vi "BRig_RT_start_v1,18__PortC.vi"() -> ()   [LabVIEW 2014]
uses:
  myRIO_BRig_RT__Case_Exp_stateList.ctl
  myRIO_BRig_RT__Case_NonExp_stateList.ctl
  <vilib>/WebDAVClient/Advanced/SessionHandle.ctl
  <vilib>/Platform/TimedLoop/XDataNode/timing_clust.ctl
  <vilib>/Platform/TimedLoop/XDataNode/nitl_modes.ctl
  <vilib>/Platform/TimedLoop/XDataNode/wakeup.ctl
  <vilib>/myRIO/Common/Instrument Driver Framework/myRIO v1.0/UART/vis/myRIO v1.0 Close UART.vi
  <vilib>/FPGAPlugInAG/myRIO-1900/niLvFpga_Open_myRIO-1900.vi
  <vilib>/rvi/interface/common/dynamic/niFpgaDynamicAddResources.vi
  <vilib>/Utility/error.llb/Error Cluster From Error Code.vi
  <vilib>/rvi/errors/niLvFpgaAdjustHostInterfaceError.vi
  <vilib>/Utility/file.llb/Read From Spreadsheet File (I64).vi
  <vilib>/Utility/file.llb/Write To Spreadsheet File (DBL).vi
  <vilib>/FPGAPlugInAG/Dynamic/niLvFpga_Close_Dynamic.vi
  <vilib>/myRIO/Common/Instrument Driver Framework/Utilities/vis/FPGA Ref Manager.vi
  <vilib>/myRIO/Common/Instrument Driver Framework/myRIO v1.0/myRIO v1.0 Reset FPGA.vi
  <vilib>/myRIO/Common/Instrument Driver Framework/myRIO v1.0/IRQ/vis/myRIO v1.0 IRQ Info FGV.vi
  <vilib>/myRIO/Common/Instrument Driver Framework/myRIO v1.0/IRQ/vis/myRIO v1.0 Timer IRQ Info FGV.vi
  <vilib>/myRIO/Common/Instrument Driver Framework/myRIO v1.0/IRQ/vis/myRIO v1.0 ISR Agent.vi
  <vilib>/rvi/interface/nirviOpenFPGA/nirviOpenFPGA.xnode
  BRig_FPGA_v3,94__PortC__build.lvbitx
  BRig_FPGA_v3,94__PortC.vi
  <vilib>/rvi/interface/nirviReadWriteControl/nirviReadWriteControl.xnode
  <vilib>/Platform/TimedLoop/XDataNode/XDataNode.xnode
  <vilib>/rvi/interface/nirviCloseFPGA/nirviCloseFPGA.xnode
  <vilib>/Platform/TimedLoop/XDataNode/XDNodeRunTimeDep.lvlib
  <vilib>/rvi/interface/Simulation/niFpgaSimulationCallBeginRW.vi
  <vilib>/myRIO/Instrument Drivers/Utilities/Utilities.lvlib
  NiFpgaLv.dll
  <vilib>/WebDAVClient/NI_WebDAV.lvlib
panel:
  out "DAB_flipLR":bool caption="Flip?\n(DAB)"
  in  "LaserFiber_V_l2":dbl
  in  "LaserFiber_V_l1":dbl
  out "Solenoid R":bool
  out "Solenoid L":bool
  out "Laser2":bool
  out "Laser1":bool
  out "FreeReward_c_R":u16
  out "FreeReward_c_L":u16
  in  "Laser2_LED":bool
  in  "Laser1_LED":bool
  in  "lick_Rising(F)_or_Falling(T)":bool
  out "T_ExpRun_min":dbl
  out "stop_TimedLoop":bool
  out "BTPR_avg_R":dbl
  out "T2R_avg_R":dbl
  out "BTPR_avg_L":dbl
  out "T2R_avg_L":dbl
  out "BTPR_block":u16
  out "T2R_block":u16
  in  "comm_WebDAV_connect":bool
  in  "I_sendData":bool
  in  "comm_TCP_connect":bool
  out "nRewards_total":u16 caption="# Rewards in Current Block"
  out "BUR_target":u16 caption="Target Trials Per Block"
  in  "input_Threshold_reset":bool
  out "nTrial":u16
  out "allReward_R":bool
  out "allReward_L":bool
  out "Threshold":bool
  out "tLoop":dbl format="%#_2g"
  out "L_Power_l2":dbl
  out "comm_TCP":bool
  in  "get_countPerMS":bool
  out "SolenoidReward":bool
  out "L_Power_l1":dbl caption="LaserPower"
  in  "Recording":bool
  out "FPGA_count2ms":dbl=159.0
  out "error out":errorcluster
  out "cSpout":enum16{"Left", "Right"}(ring) caption="Left or Right Spout"
  out "A4":u32 caption="LickCounter_Right"
  out "A2":u32 caption="LickCounter_Left"
  out "nRewards_Right":u16 caption="# Rewards Total (Right)"
  out "nRewards_Left":u16 caption="# Rewards Total (Left)"
  out "nRewards_cur":u16 caption="# Rewards in Current Block"
  out "TpB_target":u16 caption="Target Trials Per Block"
  out "cState_NonExp":T1 caption="WarmUp State"
  out "iBlock":u16 caption="Current Block"
  out "cState":T2 caption="Experimental State"
  out "iTrial":u16 caption="Current Trial"
  in  "Data Set Prefix":string="Exp1_TM2"
  out "comm_WebDAV":bool
  in  "Host Password":string="sabalab"
  in  "Host UserName":string="Test2"
  in  "STOP_abort":bool caption="Stop LabView\n(Stops myRio and FPGA)"
  in  "STOP_endBlock":bool caption="Stop Experiment\n@ End of Block"
  in  "STOP_endTrial":bool caption="Stop Experiment\n@ End of Trial"
  in  "START":bool caption="Start Experiment"
  # "Experimental Run"
  # "Recording Rig"
  # "FPGA Conversion\n[counts per ms]"
  # "RealTime Cycle\nShould be <5ms"
  # "STOP experiment at"
  # "Exp Run Time"
  # "Reset"
  # "min"
  # "Communication with Host"
  # "Lick Counter"
  # "Block Target"
  # "Give Water?\n(Reward)"
  # "# Blocks"
  # "Experimental State"
  # "Left/Right"
  # "# Trials"
  # "# Rewards"
  # "Left           Right"
  # "Bad Trials\nPost Reward"
  # "Trials 2 Reward"
  # "Direction\n(NonSpecific Licking)"
  # "Block"
  # "Laser1"
  # "Laser2"
  # "# Trials"
  # "# Rewards"
  # "Current\nBlock"
  # "L          R"
  # "Power [V]"
  # "avg L"
  # "Toggle\nLED"
  # "Total"
  # "# Rewards"
  # "Laser Trigger"
  # "# Trials"
  # "avg R"
  # "1          2"
  # "Fiber Angle\n[V]"
  # "Left           Right"
  # "FreeRewards"
  # "Solenoid Trigger"
  # "WarmUp State"
  # "Lick Detection\nRising (F) or Falling (T)"
  # "L          R"
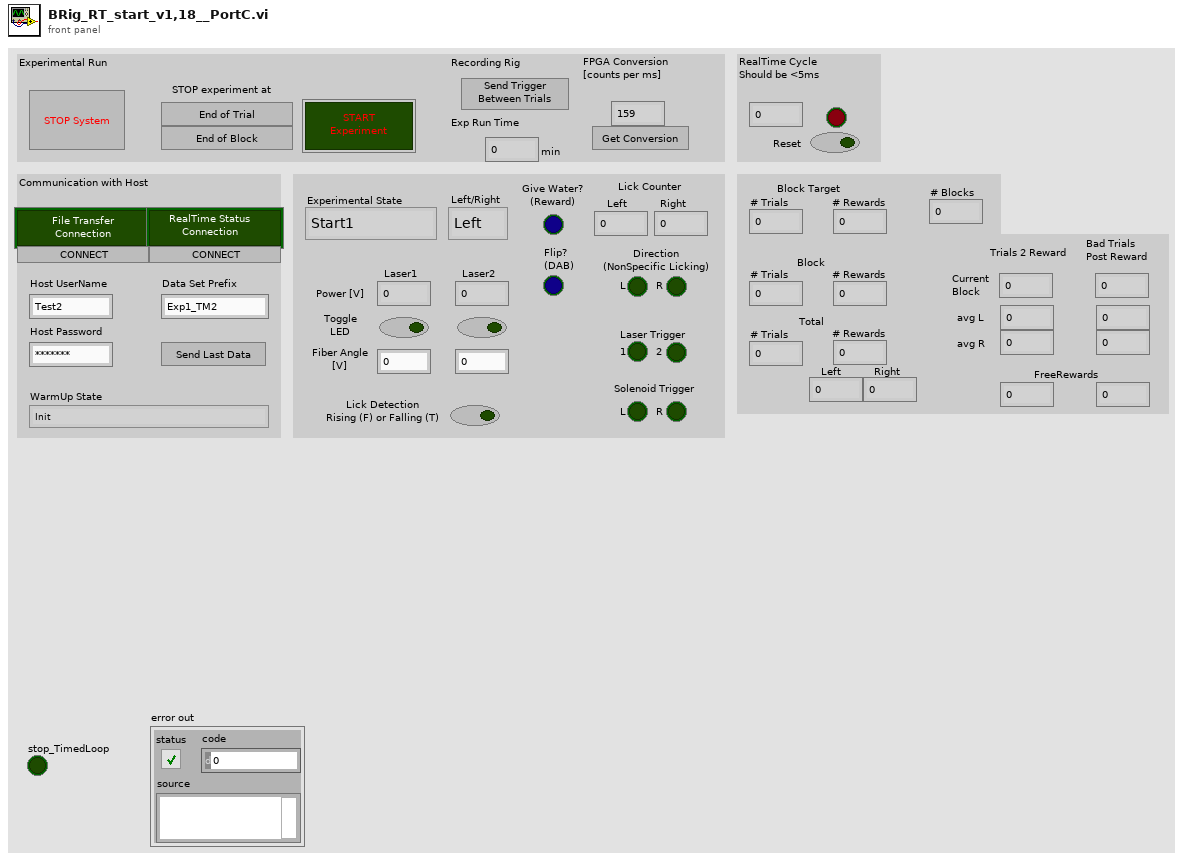
[diagram p1: front panel]
types:
  T1 = typedef "myRIO_BRig_RT__Case_NonExp_stateList.ctl" = enum16{"Init", "UploadSettings_pre", "UploadSettings_Read_dataExp", "UploadSettings_dataExp_1", "UploadSettings_dataExp_2", "UploadSettings_Read_dataLC", "UploadSettings_dataLC_1", "UploadSettings_dataLC_2", "UploadSettings_dataLC_3", "UploadSettings_dataLC_4", "UploadSettings_Read_dataMTrig", "UploadSettings_dataMTrig_1", "UploadSettings_post", "Idle_pre", "IdleEmpty", "IdleEmpty2", "IdleEmpty3", "IdleEmpty4", "Idle", "Idle_2", "Idle_3", "Idle_4", "Idle_5", "Idle_6", "Idle_post", "Cue_pre__pre", "Cue_pre", "Cue", "Cue_LED", "Cue_post", "RewardCalibration_pre", "RewardCalibration", "DispenseWater_pre__pre", "DispenseWater_pre", "DispenseWater", "DispenseWater_post", "TestConnection", "SendData", "Get_FPGA_count_per_ms", "End", "commTCP_connect"}
  T2 = typedef "myRIO_BRig_RT__Case_Exp_stateList.ctl" = enum16{"Start1", "Start2", "Start3", "saveSettings1", "saveSettings2", "saveSettings3", "saveSettings4", "saveSettings_LC_ENL_l1", "saveSettings_LC_ENL_l2", "saveSettings_LC_Cue_l1", "saveSettings_LC_Cue_l2", "saveSettings6_LC_l1_Other", "SaveSettings6_LC_l2_Other", "setSettings_Audio", "setSettings_Laser", "initBlock_pre", "initBlock", "initBlock2", "initBlock_post", "initTrial_pre", "initTrial", "initTrial2", "initTrial3", "initTrial4", "initTrial_LC_ENL1", "initTrial_LC_Cue1", "initTrial_LC_Cue1_2", "initTrial_LC_Sel", "initTrial_post", "ENL1_pre", "ENL1", "ENL1_post", "ENL1Penalty_pre", "ENL1Penalty", "ENL2_pre", "ENL2", "ENL2Penalty_pre", "ENL2Penalty", "Cue1_pre", "Cue1", "Cue1_post", "Cue1Penalty_pre", "Cue1Penalty", "Cue2_pre", "Cue2", "Cue2Penalty_pre", "Cue2Penalty", "Selection_pre", "Selection", "Select_post", "SelectReward_pre", "SelectReward", "SelectRewardPost_pre", "SelectRewardPost", "SelectWrong_pre", "SelectWrong", "SelectWrong_post", "SelectTimeout_pre", "SelectTimeout", "SelectTimeout_post", "endTrial_pre", "endTrial1", "endTrial2", "endTrial3", "endTrial_post", "endBlock_pre", "endBlock", "endBlock_post", "endExp", "commConnect", "commUpload_pre", "commUpload_dataBlock", "commUpload_dataCurrent", "commUpload_dataExp", "commUpload_dataLC", "commUpload_dataTrial", "commUpload_post", "saveData_pre", "saveData_dataBlock", "saveData_dataCurrent", "saveData_dataExp", "saveData_dataLC", "saveData_dataTrial", "saveData_post", "empty_endBlock1", "empty_endBlock2", "empty_endTrial1", "empty_endTrial2", "empty_endTrial3", "empty_endTrial4", "empty_endTrial5", "dummyState", "dummyState_endBlock", "FreeReward_pre", "FreeReward", "FreeRewardPost_pre", "FreeRewardPost"}
  T3 = enum8{"Enabled", "Disabled", "Disabled and Grayed Out"}
  T4 = typedef "NI_WebDAV.lvlib/SessionHandle.ctl" = refnum<k1>
  T5 = typedef "XDNodeRunTimeDep.lvlib/timing_clust.ctl" = cluster{"Expected End [f-1]":u64, "Actual End [f-1]":u64, "Finished Late? [f-1]":bool, "Expected End [i-1]":u64, "Actual End [i-1]":u64, "Finished Late? [i-1]":bool, "Expected Start [i]":u64, "Actual Start [i]":u64, "Expected Start [f]":u64, "Actual Start [f]":u64, "Source Name":string, "Structure Name":string, "Period":i64, "Deadline":i64, "Offset":i64, "Start":i64, "Priority":i32, "Timeout":i32, "Mode":T6, "Wakeup Reason":T7, "Error":errorcluster, "Source Type":string, "Secondary Source Type":string, "Global End Time":u64, "Global Start Time":u64, "Frame Duration":u64, "Iteration Duration":u64, "Assigned CPU":i32, "I/O Scan Engine Mode":u32}
  T6 = typedef "XDNodeRunTimeDep.lvlib/nitl_modes.ctl" = enum32{"No Change", "Process missed periods, maintain original phase", "Discard missed periods, maintain original phase", "Process missed periods, ignore original phase", "Discard missed periods, ignore original phase"}
  T7 = typedef "XDNodeRunTimeDep.lvlib/wakeup.ctl" = enum32{"Normal", "Aborted", "Asynchronous wakeup", "Timing source error", "Timed loop error", "Timeout"}
  T8 = cluster{"read mode":enum16{"polling", "blocking"}, "write mode":enum16{"polling", "blocking"}}
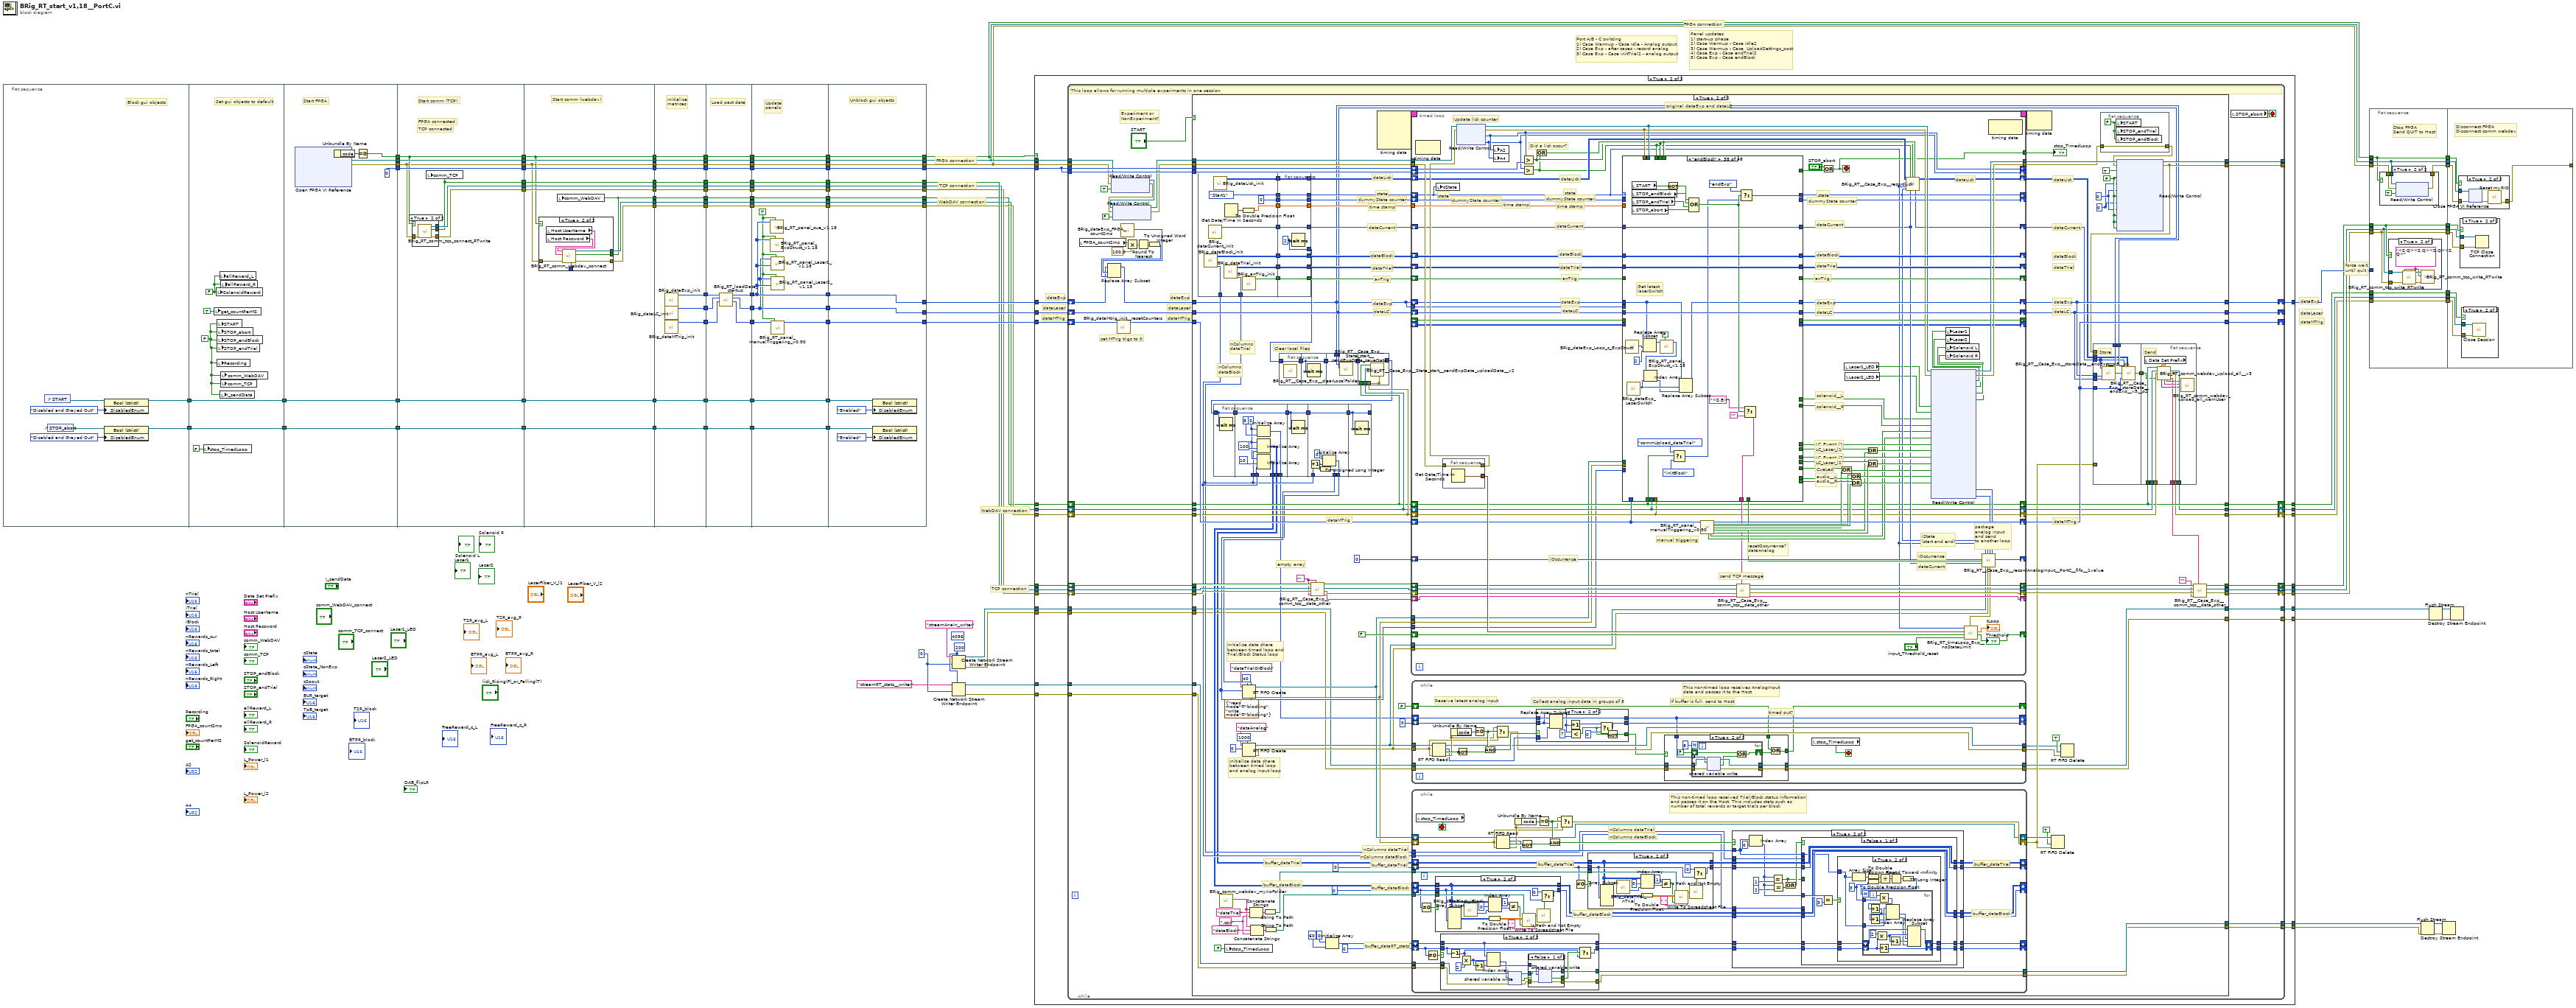
[diagram p0: block diagram]
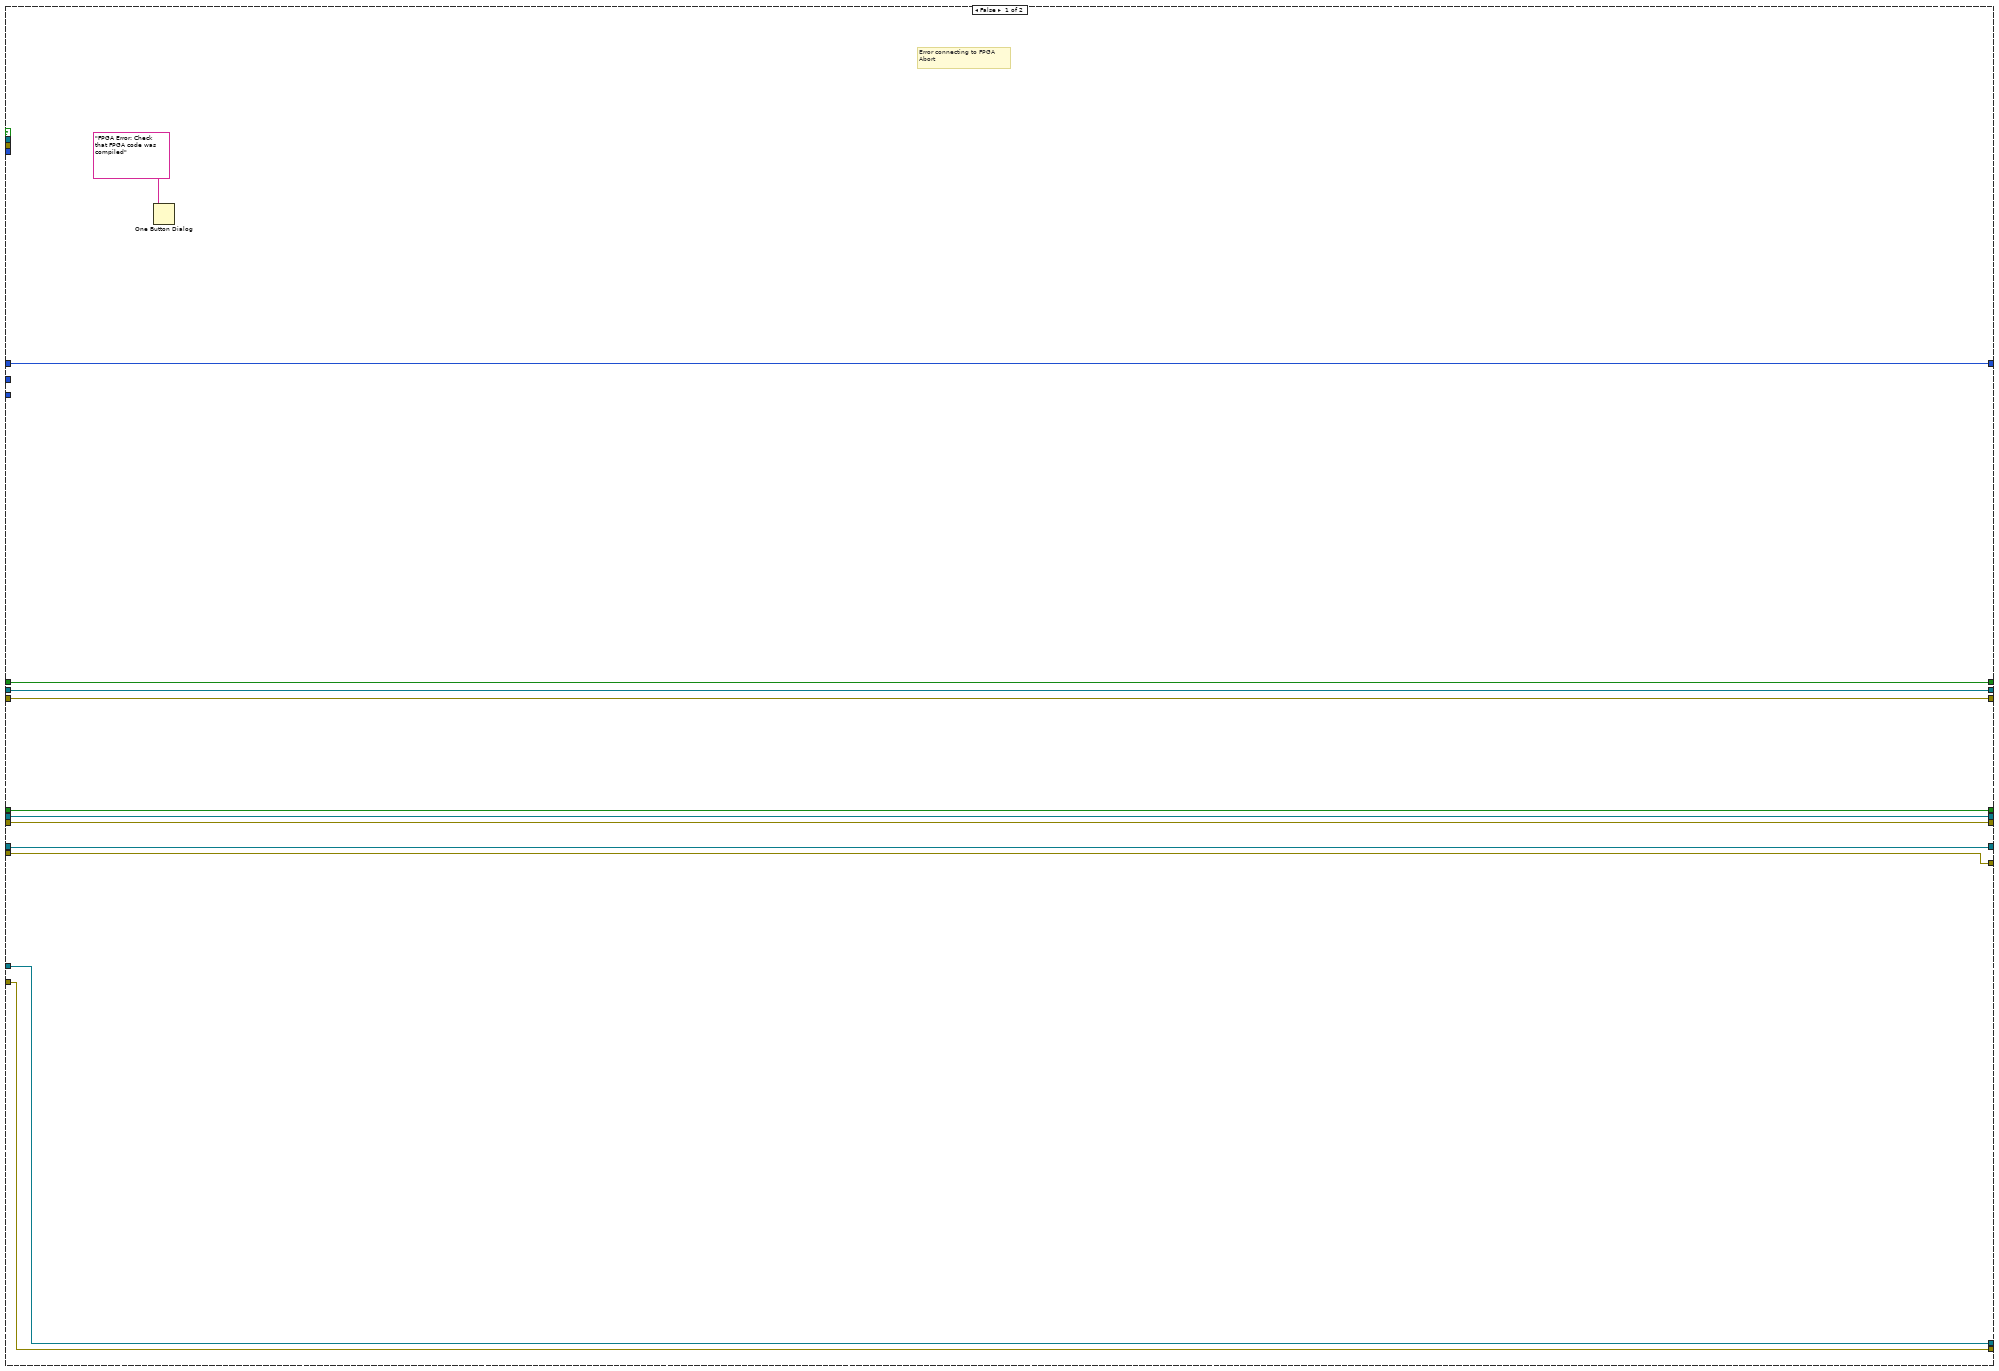
[diagram p2: hidden frame]
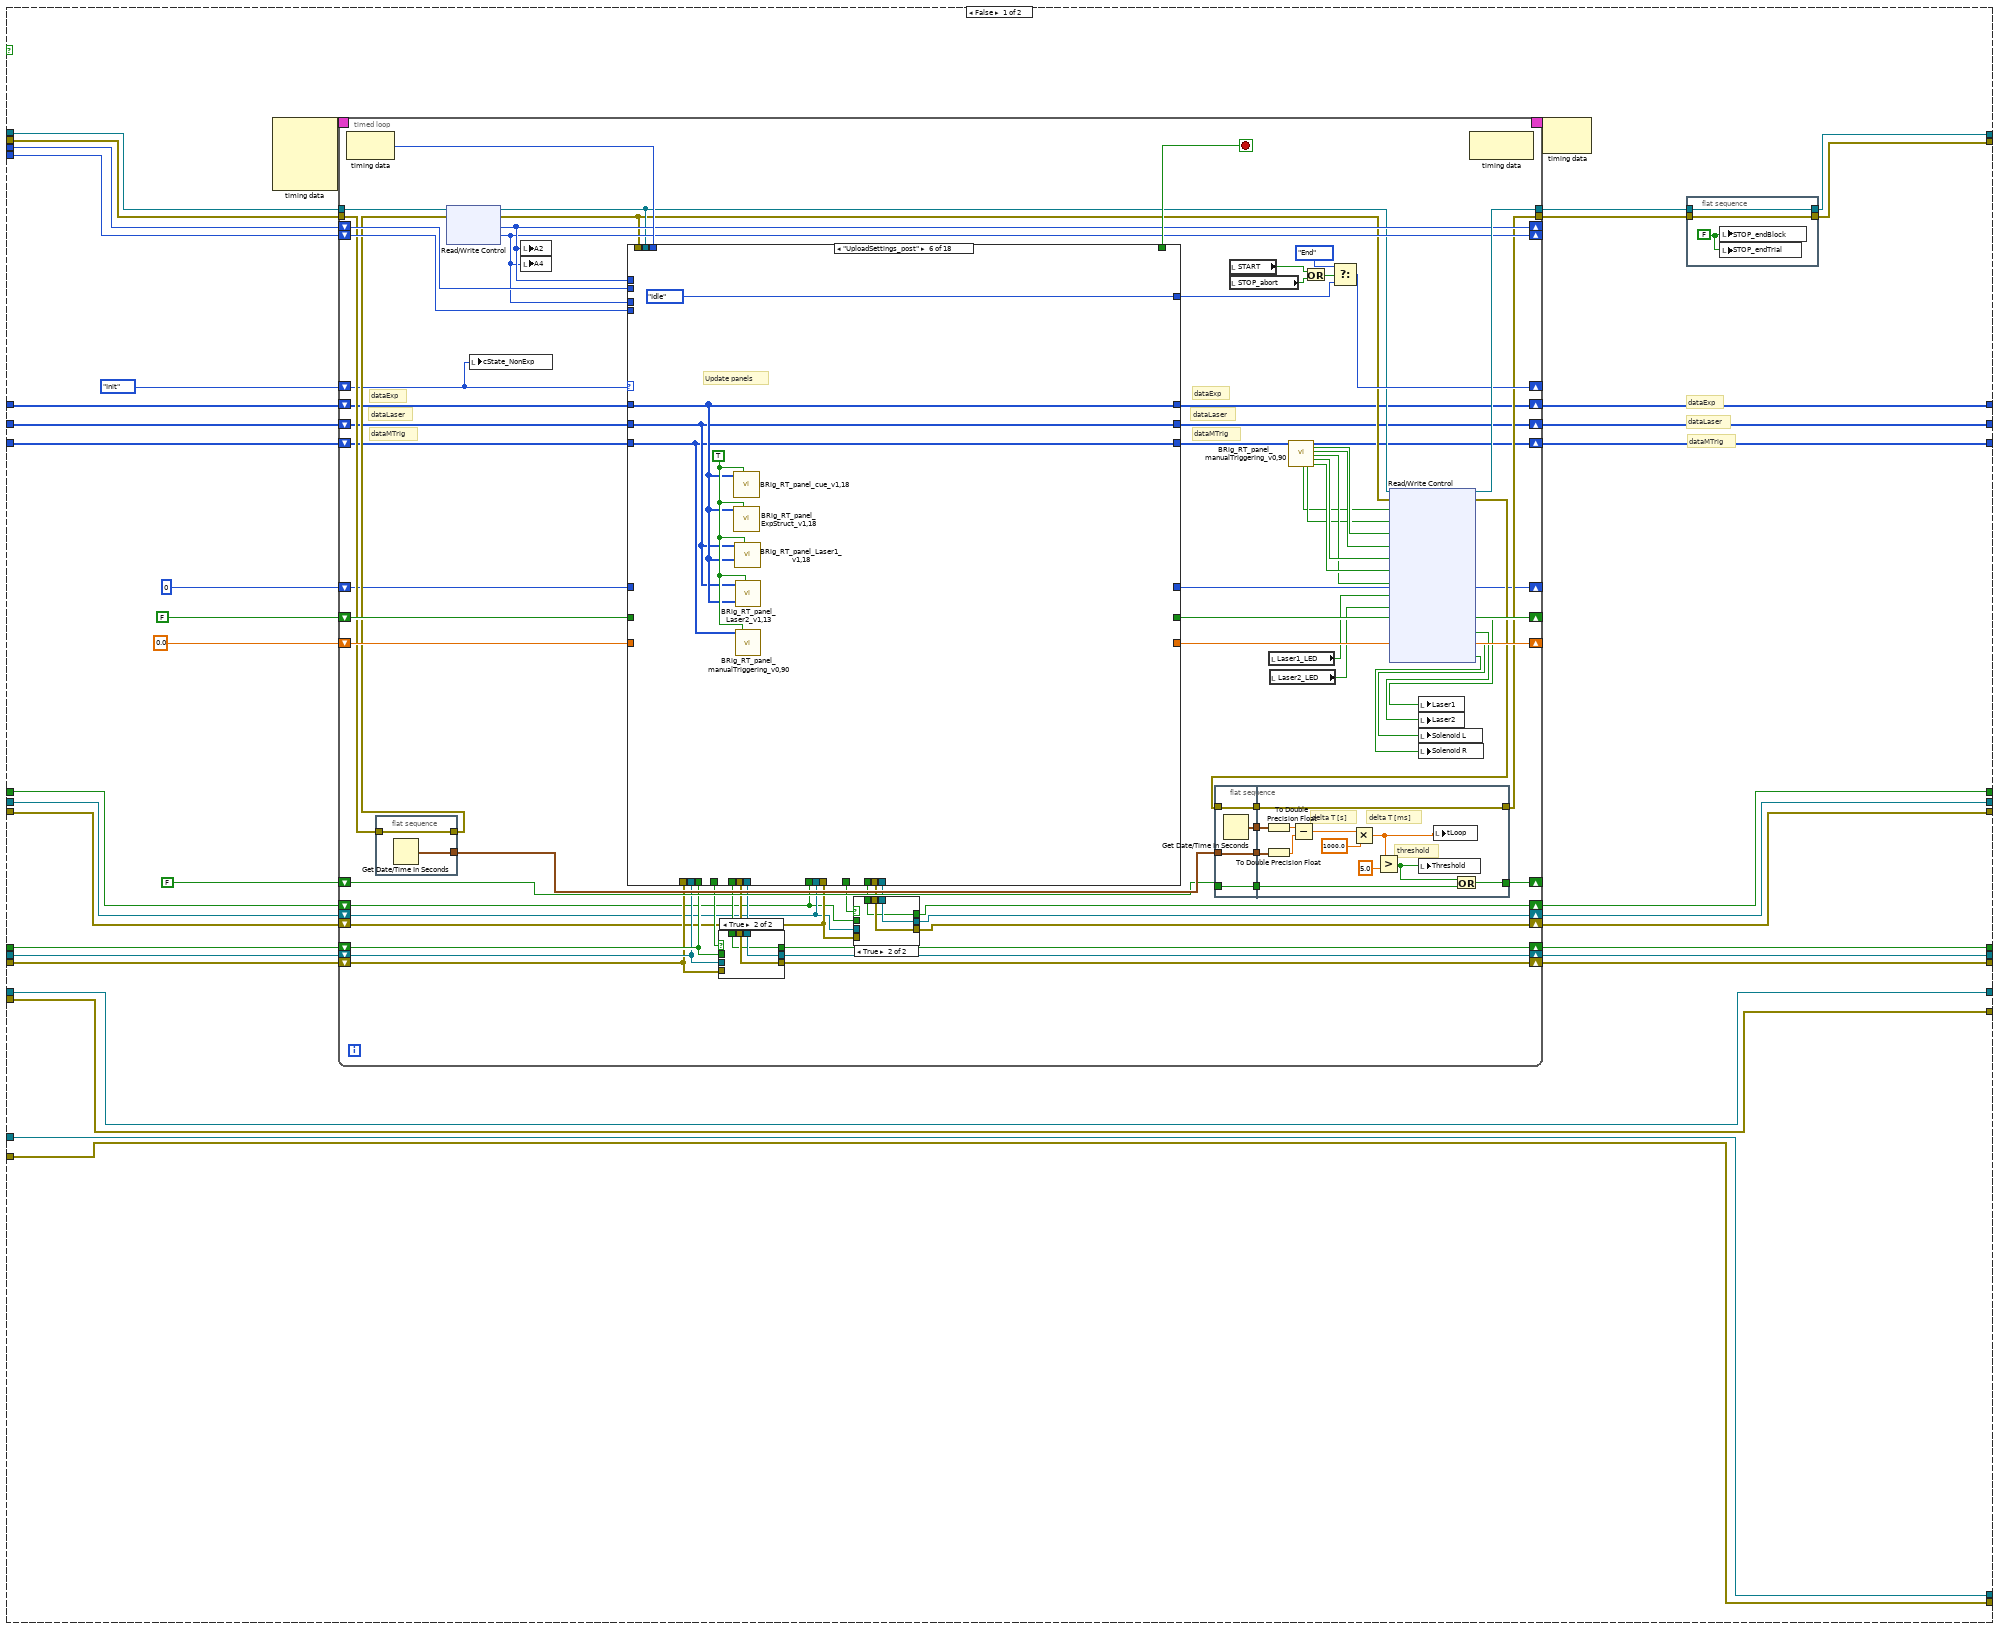
[diagram p3: hidden frame]
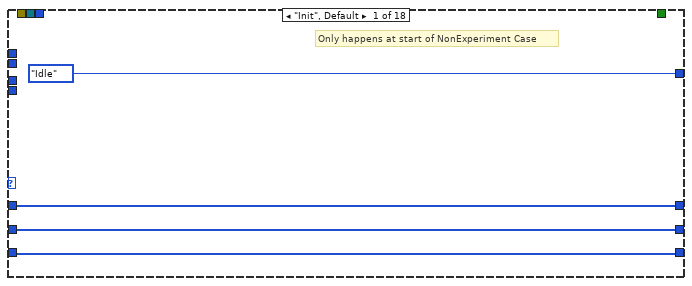
[diagram p6: hidden frame]
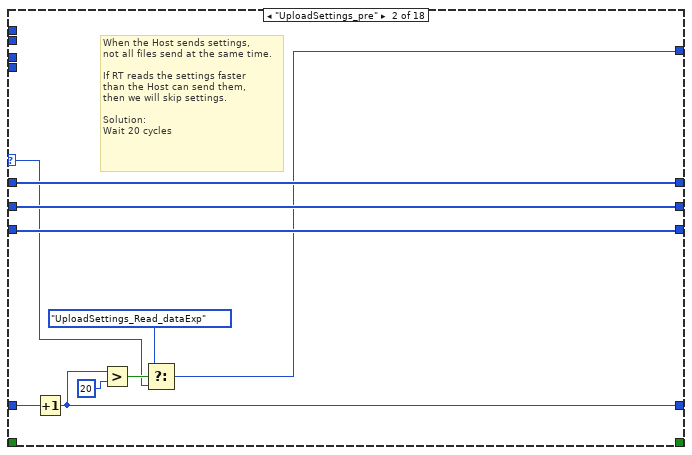
[diagram p7: hidden frame]
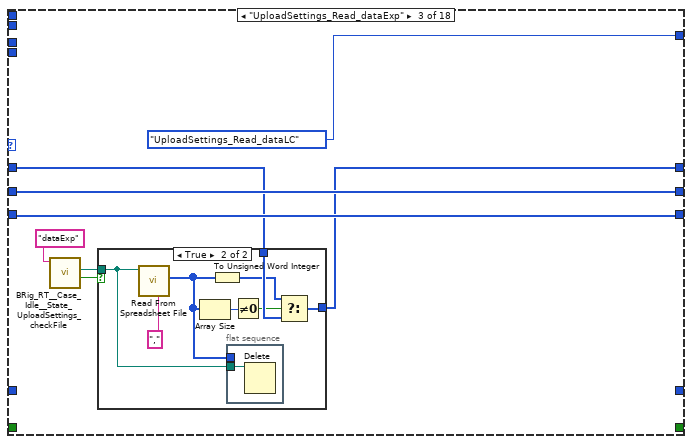
[diagram p8: hidden frame]
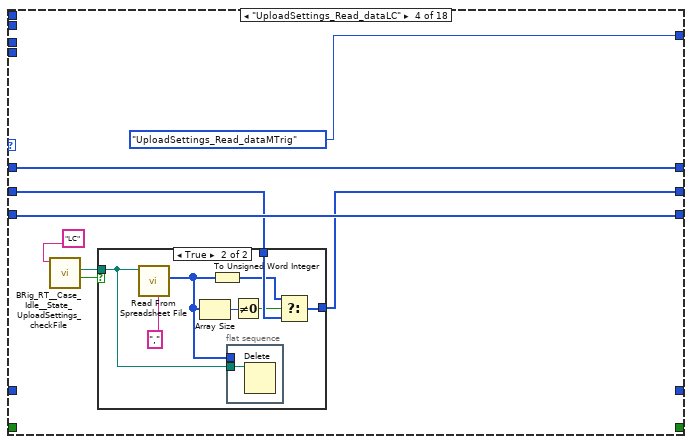
[diagram p10: hidden frame]
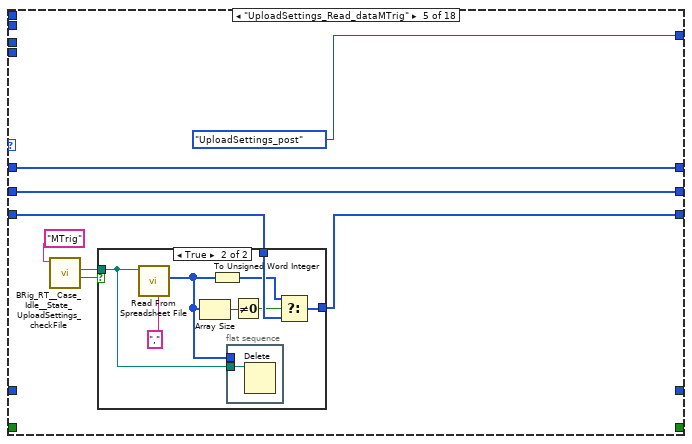
[diagram p12: hidden frame]
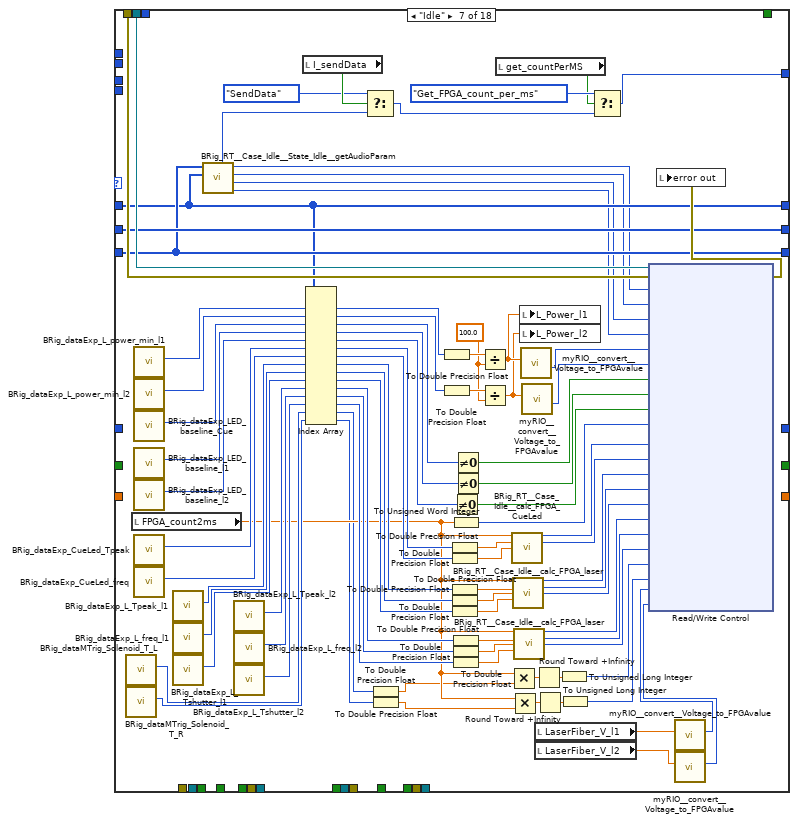
[diagram p14: hidden frame]
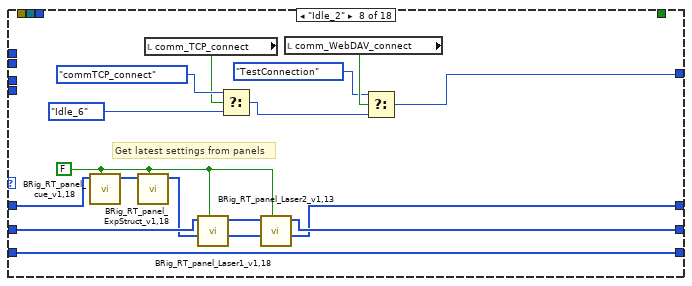
[diagram p15: hidden frame]
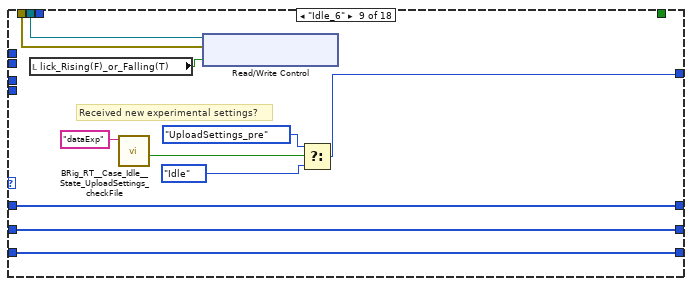
[diagram p16: hidden frame]
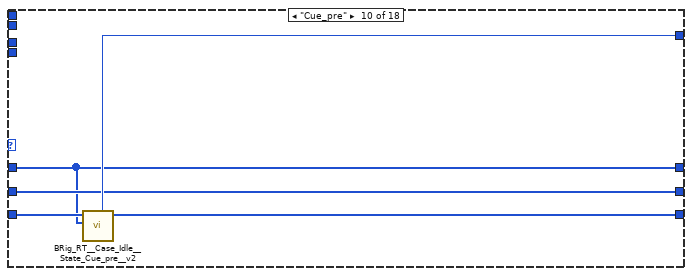
[diagram p17: hidden frame]
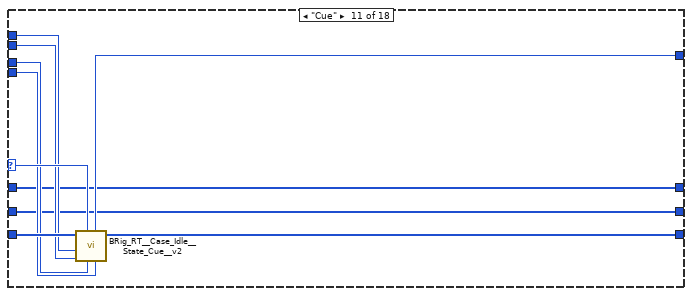
[diagram p18: hidden frame]
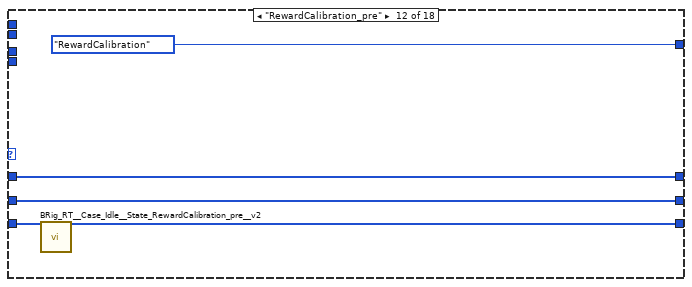
[diagram p19: hidden frame]
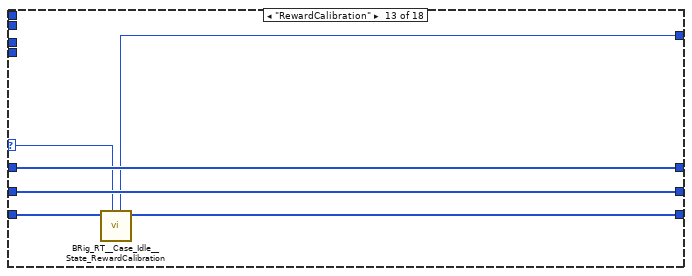
[diagram p20: hidden frame]
diagram:
  w8 = u16 0 ("element")
  (unwired) 4096 ("reader buffer size")
  w9 = 200 ("reader buffer size")
  # "Panel updates\n1) start-up phase\n2) Case Warmup - Case Idle2\n3) Case Warmup - Case  UploadSettings_post\n4) Case Exp - Case endTrial2\n5) Case Exp - Case endBlock"
  # "WebDAV connection"
  # "TCP connection"
  # "WebDAV connection"
  # "TCP connection"
  # "FPGA connection"
  # "FPGA connection"
  # "Port A/B - C switcing\n1) Case Warmup - Case Idle - Analog output\n2) Case Exp - after cases - record analog\n3) Case Exp - Case initTrial2 - analog output"
  # "force wait\nuntil quit"
  # "dataLaser"
  # "dataExp"
  # "dataMTrig"
  n1 = flat-sequence {
    tunnel: [w123] -> w106
    tunnel: [w122] -> w102
    tunnel: [w132] -> w107
    tunnel: w106 -> [w132]
    tunnel: [w131] -> w103
    tunnel: w102 -> [w131]
    tunnel: [w138] -> w120
    tunnel: [w140] -> w119
    tunnel: [u32 0] -> w118
    tunnel: [w136] -> w117
    tunnel: [w135] -> w108
    tunnel: w107 -> [w135]
    tunnel: [w134] -> w104
    tunnel: w103 -> [w134]
    tunnel: w120 -> [w146]
    tunnel: w119 -> [w149]
    tunnel: w118 -> [w148]
    tunnel: w117 -> [w147]
    tunnel: [w146] -> w116
    tunnel: [w149] -> w115
    tunnel: [w148] -> w114
    tunnel: [w147] -> w113
    tunnel: [w141] -> w112
    tunnel: [w145] -> w111
    tunnel: [w144] -> w110
    tunnel: [w143] -> w109
    tunnel: w108 -> [w143]
    tunnel: [w142] -> w105
    tunnel: w104 -> [w142]
    tunnel: w116 -> [w160]
    tunnel: w115 -> [w168]
    tunnel: w114 -> [w167]
    tunnel: w113 -> [w161]
    tunnel: w112 -> [w166]
    tunnel: w111 -> [w165]
    tunnel: w110 -> [w164]
    tunnel: [w160] -> w73
    tunnel: [w168] -> w72
    tunnel: [w167] -> w71
    tunnel: [w161] -> w70
    tunnel: [w166] -> w69
    tunnel: [w165] -> w68
    tunnel: [w164] -> w67
    tunnel: [w163] -> w66
    tunnel: w109 -> [w163]
    tunnel: [w162] -> w65
    tunnel: w105 -> [w162]
    tunnel: [w159] -> w64
    tunnel: [w157] -> w63
    tunnel: [w158] -> w62
    tunnel: w73 -> [w193]
    tunnel: [w193] -> w61
    tunnel: w72 -> [w192]
    tunnel: [w192] -> w60
    tunnel: w71 -> [w191]
    tunnel: [w191] -> w59
    tunnel: w70 -> [w190]
    tunnel: [w190] -> w58
    tunnel: w69 -> [w189]
    tunnel: [w189] -> w57
    tunnel: w68 -> [w188]
    tunnel: [w188] -> w56
    tunnel: w67 -> [w187]
    tunnel: [w187] -> w55
    tunnel: w66 -> [w186]
    tunnel: [w186] -> w54
    tunnel: w65 -> [w185]
    tunnel: [w185] -> w53
    tunnel: w64 -> [w184]
    tunnel: [w184] -> w52
    tunnel: w63 -> [w183]
    tunnel: [w183] -> w51
    tunnel: w62 -> [w182]
    tunnel: [w182] -> w50
    tunnel: [w181] -> w49
    tunnel: [w180] -> w48
    tunnel: [w179] -> w47
    tunnel: w61 -> [w211]
    tunnel: [w211] -> w46
    tunnel: w60 -> [w210]
    tunnel: [w210] -> w44
    tunnel: w59 -> [w209]
    tunnel: [w209] -> w42
    tunnel: w58 -> [w208]
    tunnel: [w208] -> w40
    tunnel: w57 -> [w207]
    tunnel: [w207] -> w38
    tunnel: w56 -> [w206]
    tunnel: [w206] -> w36
    tunnel: w55 -> [w205]
    tunnel: [w205] -> w34
    tunnel: w54 -> [w204]
    tunnel: [w204] -> w32
    tunnel: w53 -> [w203]
    tunnel: [w203] -> w30
    tunnel: w52 -> [w202]
    tunnel: [w202] -> w28
    tunnel: w51 -> [w201]
    tunnel: [w201] -> w26
    tunnel: w50 -> [w200]
    tunnel: [w200] -> w24
    tunnel: w49 -> [w195]
    tunnel: [w194] -> w22
    tunnel: w48 -> [w197]
    tunnel: [w196] -> w20
    tunnel: w47 -> [w199]
    tunnel: [w198] -> w19
    tunnel: w46 -> [w228]
    tunnel: [w228] -> w45
    tunnel: w44 -> [w227]
    tunnel: [w227] -> w43
    tunnel: w42 -> [w226]
    tunnel: [w226] -> w41
    tunnel: w40 -> [w225]
    tunnel: [w225] -> w39
    tunnel: w38 -> [w224]
    tunnel: [w224] -> w37
    tunnel: w36 -> [w223]
    tunnel: [w223] -> w35
    tunnel: w34 -> [w222]
    tunnel: [w222] -> w33
    tunnel: w32 -> [w221]
    tunnel: [w221] -> w31
    tunnel: w30 -> [w220]
    tunnel: [w220] -> w29
    tunnel: w28 -> [w219]
    tunnel: [w219] -> w27
    tunnel: w26 -> [w218]
    tunnel: [w218] -> w25
    tunnel: w24 -> [w217]
    tunnel: [w217] -> w23
    tunnel: w22 -> [w214]
    tunnel: [w213] -> w21
    tunnel: w20 -> [w215]
    tunnel: w19 -> [w216]
    tunnel: [w216] -> w18
    tunnel: [w215] -> w17
    tunnel: [w235] -> w83
    tunnel: [w236] -> w84
    tunnel: [w237] -> w85
    tunnel: [w242] -> w89
    tunnel: [w243] -> w121
    tunnel: [w244] -> w96
    tunnel: [w245] -> w95
    tunnel: w45 -> [w245]
    tunnel: w43 -> [w244]
    tunnel: w41 -> [w243]
    tunnel: w39 -> [w242]
    tunnel: w37 -> [w237]
    tunnel: w35 -> [w236]
    tunnel: w33 -> [w235]
    tunnel: w31 -> [w239]
    tunnel: w29 -> [w238]
    tunnel: w27 -> [w233]
    tunnel: w25 -> [w234]
    tunnel: w23 -> [w232]
    tunnel: [w234] -> w77
    tunnel: [w233] -> w78
    tunnel: [w232] -> w79
    tunnel: [w229] -> w92
    tunnel: [w230] -> w91
    tunnel: [w231] -> w90
    tunnel: w21 -> [w231]
    tunnel: w18 -> [w229]
    tunnel: w17 -> [w230]
    frame #0 {
      # "Block gui objects"
      n2 = control-ref of="START"() -> (w127:refnum<vi>)
      n3 = control-ref of="STOP_abort"() -> (w124:refnum<vi>)
      n4 = property class="Bool (strict)"(reference=w127, "DisabledEnum"=T3."Disabled and Grayed Out" ("Disabled")) -> (reference out=w123:refnum<vi>)  [unwired: 1 in, 1 out]
      n5 = property class="Bool (strict)"(reference=w124, "DisabledEnum"=T3."Disabled and Grayed Out" ("Disabled")) -> (reference out=w122:refnum<vi>)  [unwired: 1 in, 1 out]
    }
    frame #1 {
      w129 = FALSE ("SolenoidReward")
      w130 = FALSE
      # "Set gui objects to default"
      n6 = local write "stop_TimedLoop"(FALSE ("stop_TimedLoop")) -> ()
      n7 = local write "get_countPerMS"(TRUE ("get_countPerMS")) -> ()
      n8 = local write "SolenoidReward"(w129) -> ()
      n9 = local write "START"(w130) -> ()
      n10 = local write "STOP_abort"(w130) -> ()
      n11 = local write "STOP_endBlock"(w130) -> ()
      n12 = local write "STOP_endTrial"(w130) -> ()
      n13 = local write "Recording"(w130) -> ()
      n14 = local write "allReward_L"(w129) -> ()
      n15 = local write "I_sendData"(w130) -> ()
      n16 = local write "comm_WebDAV"(w130) -> ()
      n17 = local write "comm_TCP"(w130) -> ()
      n18 = local write "allReward_R"(w129) -> ()
    }
    frame #2 {
      # "Start FPGA"
      n19 = xnode "Open FPGA VI Reference"() -> ("FPGA VI Reference Out"=w140:refnum<k20>, "error out"=w138:errorcluster)  [unwired: 2 in]
      n20 = Unbundle By Name(w138) -> ("code"=w137:i32)
      n21 = Equal To 0?(x=w137) -> (x = 0?=w136:bool)
    }
    frame #3 {
      # "TCP connected"
      # "Start comm (TCP)"
      # "FPGA connected"
      n22 = case shown="True" w147 {
        selector: w147 -> [w150 _]
        tunnel: w146 -> [w152 w156]
        tunnel: [refnum<k5> refnum ("output_hTCP") w155] -> w145
        tunnel: [w150 w154] -> w141
        tunnel: [w152 w153] -> w144
        frame False {
        }
        frame True {
          n23 = call "BRig_RT_comm_tcp_connect_RTwrite.vi"("input_error"=w156) -> ("output_error"=w153:errorcluster, "output_connected"=w154:bool, "output_hTCP"=w155:refnum<k5>)  [unwired: 8 in]
        }
      }
      n24 = local write "comm_TCP"(w141) -> ()
    }
    frame #4 {
      # "Start comm (webdav)"
      n25 = case shown="True" w161 {
        selector: w161 -> [w170 _]
        tunnel: [w169 w176] -> w159
        tunnel: [w170 w175] -> w157
        tunnel: w160 -> [w171 w174]
        tunnel: [w171 w173] -> w158
        tunnel: [_ w172] -> _
        frame False {
          w169 = T4 refnum items=["Session NI_WebDAV"] ("output_hSession")
        }
        frame True {
          n26 = local read "Host UserName"() -> (w177:string)
          n27 = local read "Host Password"() -> (w178:string)
          n28 = call "BRig_RT_comm_webdav_connect.vi"("input_error"=w174, "input_password"=w178, "input_username"=w177) -> ("output_error"=w173:errorcluster, "output_Iconnected"=w175:bool, "output_hSession"=w176:T4, "output_code"=w172:u8)  [unwired: 5 in]
        }
      }
      n29 = local write "comm_WebDAV"(w157) -> ()
    }
    frame #5 {
      # "Initialize\nmatrices"
      n30 = call "BRig_dataExp_init.vi"() -> ("output_dataExp"=w179:u16[])  [unwired: 11 in]
      n31 = call "BRig_dataLC_init.vi"() -> ("output_dataLC"=w180:u16[])  [unwired: 11 in]
      n32 = call "BRig_dataMTrig_init.vi"() -> ("output_dataMTrig"=w181:u16[])  [unwired: 5 in]
    }
    frame #6 {
      # "Load past data"
      n33 = call "BRig_RT_loadData_startup.vi"("input_dataMTrig"=w195, "input_dataLC"=w197, "input_dataExp"=w199) -> ("output_dataMTrig"=w194:u16[], "output_dataLC"=w196:u16[], "output_dataExp"=w198:u16[])  [unwired: 6 in]
    }
    frame #7 {
      w212 = TRUE ("input_setValues")
      # "Update\npanels"
      n34 = call "BRig_RT_panel_cue_v1,18.vi"("input_setValues"=w212, "input_dataExp"=w216) -> ()  [unwired: 9 in, 1 out]
      n35 = call "BRig_RT_panel_ExpStruct_v1,18.vi"("input_setValues"=w212, "input_dataExp"=w216) -> ()  [unwired: 9 in, 1 out]
      n36 = call "BRig_RT_panel_Laser1_v1,18.vi"("input_setValues"=w212, "input_dataExp"=w216, "input_dataLC"=w215) -> ()  [unwired: 7 in, 2 out]
      n37 = call "BRig_RT_panel_Laser2_v1,13.vi"("input_setValues"=w212, "input_dataExp"=w216, "input_dataLC"=w215) -> ()  [unwired: 7 in, 2 out]
      n38 = call "BRig_RT_panel_manualTriggering_v0,90.vi"("input_dataMTrig"=w214, "input_setValues"=w212) -> ("output_dataMTrig"=w213:u16[])  [unwired: 10 in, 7 out]
    }
    frame #8 {
      # "Unblock gui objects"
      n39 = property class="Bool (strict)"(reference=w239, "DisabledEnum"=T3."Enabled" ("Disabled")) -> ()  [unwired: 1 in, 2 out]
      n40 = property class="Bool (strict)"(reference=w238, "DisabledEnum"=T3."Enabled" ("Disabled")) -> ()  [unwired: 1 in, 2 out]
    }
  }
  n41 = Create Network Stream Writer Endpoint(7:w9, 9:w8, 11:"streamAnaIn_writer" ("reader name")) -> (0:w10:errorcluster, 3:w11:refnum<k21>)  [unwired: 4 in]
  n42 = Create Network Stream Writer Endpoint(7:w9, 9:w8, 11:"streamRT_stats__writer" ("writer name")) -> (0:w5:errorcluster, 3:w6:refnum<k21>)  [unwired: 4 in]
  n43 = case shown="True" w89 {
    tunnel: w121 -> [_ w284]
    tunnel: w96 -> [_ w283]
    tunnel: w95 -> [_ w282]
    tunnel: [w257 w281] -> w93
    tunnel: w92 -> [w257 w280]
    tunnel: w91 -> [_ w279]
    tunnel: w90 -> [_ w278]
    tunnel: w85 -> [w256 w277]
    tunnel: w84 -> [w255 w276]
    tunnel: w83 -> [w254 w275]
    tunnel: [w256 w274] -> w82
    tunnel: [w255 w273] -> w81
    tunnel: [w254 w272] -> w80
    tunnel: w79 -> [w253 w271]
    tunnel: w78 -> [w252 w270]
    tunnel: w77 -> [w251 w269]
    tunnel: [w253 w268] -> w76
    tunnel: [w252 w267] -> w75
    tunnel: [w251 w266] -> w74
    tunnel: [w250 w265] -> w14
    tunnel: [w249 w264] -> w13
    tunnel: w11 -> [w250 w263]
    tunnel: w10 -> [w249 w262]
    tunnel: w6 -> [w247 w261]
    tunnel: w5 -> [w246 w260]
    tunnel: [w247 w259] -> w2
    tunnel: [w246 w258] -> w1
    frame False {
      # "Error connecting to FPGA\nAbort"
      n44 = One Button Dialog(message="FPGA Error: Check that FPGA code was compiled") -> ()  [unwired: 1 in, 1 out]
    }
    frame True {
      # "dataExp"
      # "dataLaser"
      # "dataMTrig"
      n45 = while {
        tunnel: w283 -> [w322]
        tunnel: w282 -> [w327]
        tunnel: w284 -> [w330]
        tunnel: w284 -> [w329]
        tunnel: [w320] -> _
        tunnel: [w319] -> _
        shift-right: [w318] -> _
        shift-left: w278 -> [w315]
        shift-right: [w316] -> _
        shift-left: w279 -> [w317]
        shift-right: [w286] -> w281
        shift-left: w280 -> [w295]
        shift-right: [w310] -> w274
        shift-left: w277 -> [w313]
        shift-right: [w309] -> w273
        shift-left: w276 -> [w312]
        shift-right: [w308] -> w272
        shift-left: w275 -> [w311]
        shift-right: [w304] -> w268
        shift-left: w271 -> [w307]
        shift-right: [w303] -> w267
        shift-left: w270 -> [w306]
        shift-right: [w302] -> w266
        shift-left: w269 -> [w305]
        tunnel: [w294] -> w265
        tunnel: [w293] -> w264
        tunnel: w263 -> [w292]
        tunnel: w262 -> [w291]
        tunnel: w261 -> [w290]
        tunnel: w260 -> [w289]
        tunnel: [w288] -> w259
        tunnel: [w287] -> w258
        stop <- w328 stop-if-true
        # "set MTrig trigs to 0"
        # "dataExp"
        # "dataLaser"
        # "dataMTrig"
        # "Experiment or\nNonExperiment?"
        # "This loop allows for running multiple experiments in one session"
        n46 = local read "FPGA_count2ms"() -> (w299:dbl)
        n47 = xnode "Read/Write Control"("FPGA VI Reference In"=w322, "error in"=w327, "Counts_Reset"=TRUE) -> ("FPGA VI Reference Out"=w324:refnum<k20>, "error out"=w325:errorcluster)
        n48 = xnode "Read/Write Control"("FPGA VI Reference In"=w324, "error in"=w325, "Counts_Reset"=FALSE) -> ("FPGA VI Reference Out"=w321:refnum<k20>, "error out"=w323:errorcluster)
        n49 = call "BRig_dataMtrig_init__resetCounters.vi"("input_dataMTrig"=w315) -> ("output_dataMTrig"=w314:u16[])  [unwired: 10 in]
        n50 = call "BRig_dataExp_FPGA_count2ms.vi"() -> ("output_FPGA_count2ms"=w300:i32)  [unwired: 11 in]
        n51 = Multiply(x=w299, y=100.0) -> (x*y=w297:dbl)
        n52 = Round To Nearest(number=w297) -> (nearest integer value=w296:dbl)
        n53 = To Unsigned Word Integer(number=w296) -> (unsigned 16bit integer=w301:u16)
        n54 = Replace Array Subset(array=w295, new element=w301, index=w300) -> (w285:u16[])
        n55 = case shown="True" "START" {
          tunnel: w330 -> [w366 w945]
          tunnel: w329 -> [w365 w944]
          tunnel: w323 -> [w363 w933]
          tunnel: w321 -> [w364 w934]
          tunnel: [w361 w942] -> w320
          tunnel: [w359 w911] -> w319
          tunnel: w314 -> [w355 w931]
          tunnel: [w354 w917] -> w318
          tunnel: w317 -> [w353 w881]
          tunnel: w285 -> [w333 w834]
          tunnel: [w352 w916] -> w316
          tunnel: [w351 w915] -> w286
          tunnel: w313 -> [w350 w925]
          tunnel: w312 -> [w349 w924]
          tunnel: w311 -> [w348 w923]
          tunnel: [w347 w900] -> w310
          tunnel: [w346 w899] -> w309
          tunnel: [w345 w898] -> w308
          tunnel: w307 -> [w344 w880]
          tunnel: w306 -> [w343 w879]
          tunnel: w305 -> [w342 w878]
          tunnel: [w341 w907] -> w304
          tunnel: [w340 w906] -> w303
          tunnel: [w339 w908] -> w302
          tunnel: w292 -> [w337 w839]
          tunnel: w291 -> [w336 w838]
          tunnel: [w337 w837] -> w294
          tunnel: [w336 w836] -> w293
          tunnel: w290 -> [w335 w830]
          tunnel: w289 -> [w334 w831]
          tunnel: [w335 w825] -> w288
          tunnel: [w334 w824] -> w287
          frame False {
            # "dataExp"
            # "dataLaser"
            # "dataMTrig"
            n56 = node-c288() -> (w369:T5)  [unwired: 4 in]
            n57 = timed-loop {
              timing: w369 -> [_]
              timing-out: [_] -> w368
              shift-right: [w437] -> _
              shift-left: myRIO_BRig_RT__Case_NonExp_stateList."Init" ("Enum") -> [w406]
              shift-right: [w435] -> _
              shift-left: w366 -> [w436]
              shift-right: [w433] -> _
              shift-left: w365 -> [w434]
              tunnel: [w443] -> w362
              tunnel: [w419] -> w360
              tunnel: w363 -> [w426]
              tunnel: w364 -> [w444]
              shift-right: [w429] -> _
              shift-left: FALSE -> [w430]
              shift-right: [w427] -> _
              shift-left: 0.0 -> [w428]
              shift-right: [w416] -> _
              shift-left: FALSE -> [w417]
              shift-right: [w415] -> w354
              shift-left: w355 -> [w407]
              shift-right: [w401] -> w351
              shift-left: w333 -> [w404]
              shift-right: [w402] -> w352
              shift-left: w353 -> [w403]
              shift-right: [w400] -> w347
              shift-left: w350 -> [w396]
              shift-right: [w399] -> w346
              shift-left: w349 -> [w395]
              shift-right: [w398] -> w345
              shift-left: w348 -> [w394]
              shift-right: [w384] -> w341
              shift-left: w344 -> [w390]
              shift-right: [w385] -> w340
              shift-left: w343 -> [w389]
              shift-right: [w386] -> w339
              shift-left: w342 -> [w388]
              shift-right: [w379] -> _
              shift-left: u16 0 ("y") -> [w380]
              stop <- w446 stop-if-true
              # "dataExp"
              # "dataLaser"
              # "dataExp"
              # "dataLaser"
              # "dataMTrig"
              # "dataMTrig"
              n58 = node-c288() -> (w445:i64)  [unwired: 1 in]
              n59 = flat-sequence {
                tunnel: w426 -> [w475]
                tunnel: [w476] -> w418
                tunnel: [w475] -> w425
                frame #0 {
                  n60 = Get Date/Time In Seconds() -> (seconds since 1Jan1904=w476:timestamp)
                }
              }
              n61 = xnode "Read/Write Control"("FPGA VI Reference In"=w444, "error in"=w425) -> ("FPGA VI Reference Out"=w432:refnum<k20>, "error out"=w431:errorcluster, "A2_LickL"=w435:u32, "A4_LickR"=w433:u32)
              n62 = local write "cState_NonExp"(w406) -> ()
              n63 = local write "A2"(w435) -> ()
              n64 = local write "A4"(w433) -> ()
              n65 = case shown="\"UploadSettings_post\"" w406 {
                selector: w406 -> [_ w483 _ _ _ _ _ _ _ _ w678 _ w686 _ _ w730 w773 w779]
                tunnel: [myRIO_BRig_RT__Case_NonExp_stateList."Idle" ("Enum") w484 myRIO_BRig_RT__Case_NonExp_stateList."UploadSettings_Read_dataLC" ("t") myRIO_BRig_RT__Case_NonExp_stateList."UploadSettings_Read_dataMTrig" ("t") myRIO_BRig_RT__Case_NonExp_stateList."UploadSettings_post" ("t") myRIO_BRig_RT__Case_NonExp_stateList."Idle" ("t") w569 w641 w661 w667 w676 myRIO_BRig_RT__Case_NonExp_stateList."RewardCalibration" ("Enum") w685 myRIO_BRig_RT__Case_NonExp_stateList."Idle" ("Enum") myRIO_BRig_RT__Case_NonExp_stateList."Idle" ("Enum") w729 w773 w780] -> w438
                tunnel: [w479 w490 w498 w516 w530 w545 w581 w653 w659 w668 w677 w680 w687 w701 w713 w739 w771 w788] -> w405
                tunnel: [_ _ _ _ _ _ _ _ _ _ _ _ _ _ _ _ TRUE _] -> w446
                tunnel: w407 -> [w479 w490 w498 w516 w527 w545 w581 w653 w659 w669 w679 w681 w688 w701 w713 w739 w771 w788]
                tunnel: w445 -> [_ _ _ _ _ _ _ _ _ _ _ _ _ _ _ _ _ _]
                tunnel: w436 -> [_ _ _ _ _ _ _ _ _ _ w674 _ _ _ _ _ _ _]
                tunnel: w435 -> [_ _ _ _ _ _ _ _ _ _ w675 _ _ _ _ _ _ _]
                tunnel: w434 -> [_ _ _ _ _ _ _ _ _ _ w672 _ _ _ _ _ _ _]
                tunnel: w433 -> [_ _ _ _ _ _ _ _ _ _ w673 _ _ _ _ _ _ _]
                tunnel: w432 -> [_ _ _ _ _ _ w636 _ w656 _ _ _ _ _ _ w734 _ _]
                tunnel: w431 -> [_ _ _ _ _ _ w635 _ w655 _ _ _ _ _ _ w733 _ _]
                tunnel: w430 -> [_ _ _ _ _ _ _ _ _ _ _ _ _ _ _ w738 _ _]
                tunnel: [_ _ _ _ _ _ _ _ _ _ _ _ _ _ _ TRUE _ _] -> w429
                tunnel: w428 -> [_ _ _ _ _ _ _ _ _ _ _ _ _ _ _ w736 _ _]
                tunnel: [_ _ _ _ _ _ _ _ _ _ _ _ _ _ _ w735 _ _] -> w427
                tunnel: w404 -> [w477 w488 w493 w515 w534 w547 w580 w640 w657 w665 w670 w683 w689 w698 w710 w726 w769 w786]
                tunnel: w403 -> [w478 w489 w497 w509 w531 w546 w582 w652 w658 w666 w671 w682 w690 w699 w711 w727 w770 w787]
                tunnel: [w478 w489 w497 w512 w531 w546 w582 w648 w658 w666 w671 w682 w690 w699 w711 w727 w770 w787] -> w402
                tunnel: [w477 w488 w492 w515 w534 w547 w580 w637 w657 w665 w670 w683 w689 w698 w710 w726 w769 w786] -> w401
                tunnel: [_ _ _ _ _ _ _ _ _ _ _ _ _ _ _ _ _ TRUE] -> w397
                tunnel: w396 -> [_ _ _ _ _ _ _ _ _ _ _ _ _ _ w704 _ _ w785]
                tunnel: w395 -> [_ _ _ _ _ _ _ _ _ _ _ _ _ _ w706 _ _ w781]
                tunnel: w394 -> [_ _ _ _ _ _ _ _ _ _ _ _ _ _ w705 _ _ w784]
                tunnel: [_ _ _ _ _ _ _ _ _ _ _ _ _ _ _ _ _ w783] -> w393
                tunnel: [_ _ _ _ _ _ _ _ _ _ _ _ _ _ _ _ _ w782] -> w392
                tunnel: [_ _ _ _ _ _ _ _ _ _ _ _ _ _ _ _ _ w774] -> w391
                tunnel: w388 -> [_ _ _ _ _ _ _ _ _ _ _ _ _ _ w703 _ _ _]
                tunnel: w389 -> [_ _ _ _ _ _ _ _ _ _ _ _ _ _ w709 _ _ _]
                tunnel: w390 -> [_ _ _ _ _ _ _ _ _ _ _ _ _ w691 w708 _ _ _]
                tunnel: [_ _ _ _ _ _ _ _ _ _ _ _ _ TRUE _ _ _ _] -> w387
                tunnel: [_ _ _ _ _ _ _ _ _ _ _ _ _ w693 _ _ _ _] -> w383
                tunnel: [_ _ _ _ _ _ _ _ _ _ _ _ _ w691 _ _ _ _] -> w382
                tunnel: [_ _ _ _ _ _ _ _ _ _ _ _ _ w692 _ _ _ _] -> w381
                tunnel: w380 -> [_ w482 _ _ _ _ _ _ _ _ _ _ _ _ _ _ _ _]
                tunnel: [_ w481 _ _ _ _ _ _ _ _ _ _ _ _ _ _ _ _] -> w379
                frame "Init", Default {
                  # "Only happens at start of NonExperiment Case"
                }
                frame "UploadSettings_pre" {
                  # "When the Host sends settings,\nnot all files send at the same time.\n\nIf RT reads the settings faster\nthan the Host can send them,\nthen we will skip settings.\n\nSolution:\nWait 20 cycles"
                  n66 = Increment(x=w482) -> (x+1=w481:u16)
                  n67 = Greater?(x=w481, y=u16 20) -> (0:w486:bool)
                  n68 = Select(t=myRIO_BRig_RT__Case_NonExp_stateList."UploadSettings_Read_dataExp", s=w486, f=w483) -> (s? t:f=w484:T1)
                }
                frame "UploadSettings_Read_dataExp" {
                  n69 = call "BRig_RT__Case_Idle__State_UploadSettings_checkFile.vi"("input_dataName"="dataExp") -> ("output_Iexist"=w495:bool, "output_dataPath"=w494:path)  [unwired: 9 in]
                  n70 = case shown="True" w495 {
                    tunnel: w494 -> [_ w501]
                    tunnel: w493 -> [w499 w505]
                    tunnel: [w499 w503] -> w492
                    frame False {
                    }
                    frame True {
                      n71 = call-poly <vilib>:"Read From Spreadsheet File.vi"("delimiter (\\t)"="," ("delimiter (\\t)"), "file path (dialog if empty)"=w501) -> ("first row"=w500:i64[])  [unwired: 5 in, 4 out]
                      n72 = Array Size(array=w500) -> (size(s)=w506:i32)
                      n73 = To Unsigned Word Integer(number=w500) -> (unsigned 16bit integer=w504:u16[])
                      n74 = flat-sequence {
                        tunnel: w501 -> [w508]
                        tunnel: w500 -> [_]
                        frame #0 {
                          n75 = Delete(path (use dialog)=w508) -> ()  [unwired: 4 in, 3 out]
                        }
                      }
                      n76 = Not Equal To 0?(x=w506) -> (x != 0?=w502:bool)
                      n77 = Select(t=w504, s=w502, f=w505) -> (s? t:f=w503:u16[])
                    }
                  }
                }
                frame "UploadSettings_Read_dataLC" {
                  n78 = call "BRig_RT__Case_Idle__State_UploadSettings_checkFile.vi"("input_dataName"="LC") -> ("output_Iexist"=w510:bool, "output_dataPath"=w511:path)  [unwired: 9 in]
                  n79 = case shown="True" w510 {
                    tunnel: w511 -> [_ w519]
                    tunnel: w509 -> [w517 w523]
                    tunnel: [w517 w521] -> w512
                    frame False {
                    }
                    frame True {
                      n80 = call-poly <vilib>:"Read From Spreadsheet File.vi"("delimiter (\\t)"="," ("delimiter (\\t)"), "file path (dialog if empty)"=w519) -> ("first row"=w518:i64[])  [unwired: 5 in, 4 out]
                      n81 = Array Size(array=w518) -> (size(s)=w524:i32)
                      n82 = To Unsigned Word Integer(number=w518) -> (unsigned 16bit integer=w522:u16[])
                      n83 = flat-sequence {
                        tunnel: w519 -> [w526]
                        tunnel: w518 -> [_]
                        frame #0 {
                          n84 = Delete(path (use dialog)=w526) -> ()  [unwired: 4 in, 3 out]
                        }
                      }
                      n85 = Not Equal To 0?(x=w524) -> (x != 0?=w520:bool)
                      n86 = Select(t=w522, s=w520, f=w523) -> (s? t:f=w521:u16[])
                    }
                  }
                }
                frame "UploadSettings_Read_dataMTrig" {
                  n87 = call "BRig_RT__Case_Idle__State_UploadSettings_checkFile.vi"("input_dataName"="MTrig") -> ("output_Iexist"=w528:bool, "output_dataPath"=w529:path)  [unwired: 9 in]
                  n88 = case shown="True" w528 {
                    tunnel: w529 -> [_ w537]
                    tunnel: w527 -> [w535 w541]
                    tunnel: [w535 w539] -> w530
                    frame False {
                    }
                    frame True {
                      n89 = call-poly <vilib>:"Read From Spreadsheet File.vi"("delimiter (\\t)"="," ("delimiter (\\t)"), "file path (dialog if empty)"=w537) -> ("first row"=w536:i64[])  [unwired: 5 in, 4 out]
                      n90 = Array Size(array=w536) -> (size(s)=w542:i32)
                      n91 = To Unsigned Word Integer(number=w536) -> (unsigned 16bit integer=w540:u16[])
                      n92 = flat-sequence {
                        tunnel: w537 -> [w544]
                        tunnel: w536 -> [_]
                        frame #0 {
                          n93 = Delete(path (use dialog)=w544) -> ()  [unwired: 4 in, 3 out]
                        }
                      }
                      n94 = Not Equal To 0?(x=w542) -> (x != 0?=w538:bool)
                      n95 = Select(t=w540, s=w538, f=w541) -> (s? t:f=w539:u16[])
                    }
                  }
                }
                frame "UploadSettings_post" {
                  w548 = TRUE ("input_setValues")
                  # "Update panels"
                  n96 = call "BRig_RT_panel_cue_v1,18.vi"("input_setValues"=w548, "input_dataExp"=w547) -> ()  [unwired: 9 in, 1 out]
                  n97 = call "BRig_RT_panel_ExpStruct_v1,18.vi"("input_setValues"=w548, "input_dataExp"=w547) -> ()  [unwired: 9 in, 1 out]
                  n98 = call "BRig_RT_panel_Laser1_v1,18.vi"("input_setValues"=w548, "input_dataExp"=w547, "input_dataLC"=w546) -> ()  [unwired: 7 in, 2 out]
                  n99 = call "BRig_RT_panel_Laser2_v1,13.vi"("input_setValues"=w548, "input_dataExp"=w547, "input_dataLC"=w546) -> ()  [unwired: 7 in, 2 out]
                  n100 = call "BRig_RT_panel_manualTriggering_v0,90.vi"("input_dataMTrig"=w545, "input_setValues"=w548) -> ()  [unwired: 10 in, 8 out]
                }
                frame "Idle" {
                  w626 = 100.0 ("y")
                  n101 = call "BRig_dataMTrig_Solenoid_T_L.vi"() -> ("output_Solenoid_T_L"=w564:i32)  [unwired: 11 in]
                  n102 = call "BRig_dataMTrig_Solenoid_T_R.vi"() -> ("output_Solenoid_T_R"=w563:i32)  [unwired: 11 in]
                  n103 = local read "FPGA_count2ms"() -> (w562:dbl)
                  n104 = call "BRig_dataExp_L_power_min_l1.vi"() -> ("output_L_power_min_l1"=w631:i32)  [unwired: 11 in]
                  n105 = call "BRig_dataExp_L_power_min_l2.vi"() -> ("output_L_power_min_l2"=w630:i32)  [unwired: 11 in]
                  n106 = call "BRig_dataExp_LED_baseline_Cue.vi"() -> ("output_LED_baseline_Cue"=w624:i32)  [unwired: 11 in]
                  n107 = call "BRig_dataExp_LED_baseline_l1.vi"() -> ("output_LED_baseline_l1"=w623:i32)  [unwired: 11 in]
                  n108 = call "BRig_dataExp_LED_baseline_l2.vi"() -> ("output_LED_baseline_l2"=w622:i32)  [unwired: 11 in]
                  n109 = call "BRig_dataExp_CueLed_Tpeak.vi"() -> ("output_CueLed_Tpeak"=w614:i32)  [unwired: 11 in]
                  n110 = call "BRig_dataExp_CueLed_freq.vi"() -> ("output_CueLed_Freq"=w613:i32)  [unwired: 11 in]
                  n111 = call "BRig_dataExp_L_Tpeak_l1.vi"() -> ("output_L_Tpeak_l1"=w606:i32)  [unwired: 11 in]
                  n112 = call "BRig_dataExp_L_freq_l1.vi"() -> ("output_L_freq_l1"=w605:i32)  [unwired: 11 in]
                  n113 = call "BRig_dataExp_L_Tshutter_l1.vi"() -> ("output_L_Tshutter_l1"=w604:i32)  [unwired: 11 in]
                  n114 = call "BRig_RT__Case_Idle__State_Idle__getAudioParam.vi"("input_dataExp"=w580, "input_dataMTrig"=w581) -> ("output_Audio_freq_R"=w576:u8, "output_Audio_amp_R"=w577:u16, "output_Audio_freq_L"=w578:u8, "output_Audio_amp_L"=w579:u16, "output_state"=w575:T1)  [unwired: 5 in]
                  n115 = call "BRig_dataExp_L_Tpeak_l2.vi"() -> ("output_L_Tpeak_l2"=w588:i32)  [unwired: 11 in]
                  n116 = call "BRig_dataExp_L_freq_l2.vi"() -> ("output_L_freq_l2"=w587:i32)  [unwired: 11 in]
                  n117 = call "BRig_dataExp_L_Tshutter_l2.vi"() -> ("output_L_Tshutter_l2"=w586:i32)  [unwired: 11 in]
                  n118 = local read "I_sendData"() -> (w574:bool)
                  n119 = Index Array(array=w580, index #1=w631, index #2=w630, index #3=w624, index #4=w623, index #5=w622, index #6=w614, index #7=w613, index #8=w606, index #9=w605, index #10=w604, index #11=w588, index #12=w587, index #13=w586, index #14=w564, index #15=w563) -> (element #1=w629:u16, element #2=w625:u16, element #3=w621:u16, element #4=w620:u16, element #5=w619:u16, element #6=w610:u16, element #7=w609:u16, element #8=w603:u16, element #9=w602:u16, element #10=w601:u16, element #11=w591:u16, element #12=w590:u16, element #13=w589:u16, element #14=w561:u16, element #15=w560:u16)
                  n120 = Select(t=myRIO_BRig_RT__Case_NonExp_stateList."SendData" ("Enum"), s=w574, f=w575) -> (s? t:f=w571:T1)
                  n121 = To Double Precision Float(number=w561) -> (double precision float=w559:dbl)
                  n122 = To Double Precision Float(number=w560) -> (double precision float=w558:dbl)
                  n123 = To Double Precision Float(number=w629) -> (double precision float=w628:dbl)
                  n124 = To Double Precision Float(number=w625) -> (double precision float=w627:dbl)
                  n125 = To Double Precision Float(number=w610) -> (double precision float=w612:dbl)
                  n126 = To Double Precision Float(number=w609) -> (double precision float=w611:dbl)
                  n127 = To Double Precision Float(number=w603) -> (double precision float=w600:dbl)
                  n128 = To Double Precision Float(number=w602) -> (double precision float=w599:dbl)
                  n129 = To Double Precision Float(number=w601) -> (double precision float=w598:dbl)
                  n130 = To Unsigned Word Integer(number=w562) -> (unsigned 16bit integer=w615:u16)
                  n131 = To Double Precision Float(number=w591) -> (double precision float=w592:dbl)
                  n132 = To Double Precision Float(number=w590) -> (double precision float=w593:dbl)
                  n133 = To Double Precision Float(number=w589) -> (double precision float=w594:dbl)
                  n134 = Not Equal To 0?(x=w619) -> (x != 0?=w616:bool)
                  n135 = Not Equal To 0?(x=w621) -> (x != 0?=w618:bool)
                  n136 = Not Equal To 0?(x=w620) -> (x != 0?=w617:bool)
                  n137 = Divide(x=w628, y=w626) -> (x/y=w555:dbl)
                  n138 = Divide(x=w627, y=w626) -> (x/y=w554:dbl)
                  n139 = local read "get_countPerMS"() -> (w570:bool)
                  n140 = Multiply(x=w562, y=w559) -> (x*y=w568:dbl)
                  n141 = Multiply(x=w562, y=w558) -> (x*y=w566:dbl)
                  n142 = call "BRig_RT__Case_Idle__calc_FPGA_CueLed.vi"("input_FPGA_ms2count"=w562, "input_Tpeak"=w612, "input_Freq"=w611) -> ("output_laser_Npeak"=w608:u32, "output_laser_Nvalley"=w607:u32)  [unwired: 11 in]
                  n143 = call "BRig_RT__Case_Idle__calc_FPGA_laser.vi"("input_FPGA_ms2count"=w562, "input_Tpeak"=w600, "input_Freq"=w599, "input_Tshutter"=w598) -> ("output_laser_Npeak"=w597:u32, "output_laser_Nvalley"=w596:u32, "output_laser_Nshutter"=w595:u32)  [unwired: 9 in]
                  n144 = call "BRig_RT__Case_Idle__calc_FPGA_laser.vi"("input_FPGA_ms2count"=w562, "input_Tpeak"=w592, "input_Freq"=w593, "input_Tshutter"=w594) -> ("output_laser_Npeak"=w585:u32, "output_laser_Nvalley"=w584:u32, "output_laser_Nshutter"=w583:u32)  [unwired: 9 in]
                  n145 = local write "L_Power_l1"(w555) -> ()
                  n146 = local write "L_Power_l2"(w554) -> ()
                  n147 = call "myRIO__convert__Voltage_to_FPGAvalue.vi"("input_voltage"=w555) -> ("output_PortC"=w632:i16)  [unwired: 9 in, 1 out]
                  n148 = call "myRIO__convert__Voltage_to_FPGAvalue.vi"("input_voltage"=w554) -> ("output_PortC"=w633:i16)  [unwired: 9 in, 1 out]
                  n149 = Round Toward +Infinity(x=w568) -> (ceil(x): smallest int >= x=w567:dbl)
                  n150 = Round Toward +Infinity(x=w566) -> (ceil(x): smallest int >= x=w565:dbl)
                  n151 = local read "LaserFiber_V_l1"() -> (w552:dbl)
                  n152 = local read "LaserFiber_V_l2"() -> (w553:dbl)
                  n153 = To Unsigned Long Integer(number=w567) -> (unsigned 32bit integer=w557:u32)
                  n154 = To Unsigned Long Integer(number=w565) -> (unsigned 32bit integer=w556:u32)
                  n155 = Select(t=myRIO_BRig_RT__Case_NonExp_stateList."Get_FPGA_count_per_ms" ("Enum"), s=w570, f=w571) -> (s? t:f=w569:T1)
                  n156 = call "myRIO__convert__Voltage_to_FPGAvalue.vi"("input_voltage"=w552) -> ("output_PortA"=w551:u16)  [unwired: 9 in, 1 out]
                  n157 = call "myRIO__convert__Voltage_to_FPGAvalue.vi"("input_voltage"=w553) -> ("output_PortA"=w550:u16)  [unwired: 9 in, 1 out]
                  n158 = xnode "Read/Write Control"("FPGA VI Reference In"=w636, "error in"=w635, "audioAmp_L"=w579, "audioFreq_L_kHz"=w578, "audioAmp_R"=w577, "audioFreq_R_kHz"=w576, "AnaOut_0"=w632, "AnaOut_1"=w633, "CueLed_Baseline"=w618, "L1Led_Baseline"=w617, "L2Led_Baseline"=w616, "k1__counter_per_ms"=w615, "CueLed_nPeak"=w608, "CueLed_nValley"=w607, "LC_nPeak_l1"=w597, "LC_nValley_l1"=w596, "LC_nShutter_l1"=w595, "LC_nPeak_l2"=w585, "LC_nValley_l2"=w584, "LC_nShutter_l2"=w583, "Solenoid_nTotal_L"=w557, "Solenoid_nTotal_R"=w556, "AnaOut0_Pair"=w551, "AnaOut1_Pair"=w550) -> ("error out"=w634:errorcluster)  [unwired: 1 out]
                  n159 = local write "error out"(w634) -> ()
                }
                frame "Idle_2" {
                  w646 = FALSE
                  # "Get latest settings from panels"
                  n160 = call "BRig_RT_panel_cue_v1,18.vi"("input_setValues"=w646, "input_dataExp"=w640) -> ("output_dataExp"=w639:u16[])  [unwired: 9 in]
                  n161 = call "BRig_RT_panel_ExpStruct_v1,18.vi"("input_setValues"=w646, "input_dataExp"=w639) -> ("output_dataExp"=w638:u16[])  [unwired: 9 in]
                  n162 = local read "comm_TCP_connect"() -> (w645:bool)
                  n163 = call "BRig_RT_panel_Laser1_v1,18.vi"("input_setValues"=w646, "input_dataExp"=w638, "input_dataLC"=w652) -> ("output_dataExp"=w647:u16[], "output_dataLC"=w649:u16[])  [unwired: 7 in]
                  n164 = Select(t=myRIO_BRig_RT__Case_NonExp_stateList."commTCP_connect" ("Enum"), s=w645, f=myRIO_BRig_RT__Case_NonExp_stateList."Idle_6" ("Enum")) -> (s? t:f=w643:T1)
                  n165 = call "BRig_RT_panel_Laser2_v1,13.vi"("input_setValues"=w646, "input_dataExp"=w647, "input_dataLC"=w649) -> ("output_dataExp"=w637:u16[], "output_dataLC"=w648:u16[])  [unwired: 7 in]
                  n166 = local read "comm_WebDAV_connect"() -> (w644:bool)
                  n167 = Select(t=myRIO_BRig_RT__Case_NonExp_stateList."TestConnection" ("Enum"), s=w644, f=w643) -> (s? t:f=w641:T1)
                }
                frame "Idle_6" {
                  # "Received new experimental settings?"
                  n168 = local read "lick_Rising(F)_or_Falling(T)"() -> (w654:bool)
                  n169 = call "BRig_RT__Case_Idle__State_UploadSettings_checkFile.vi"("input_dataName"="dataExp") -> ("output_Iexist"=w663:bool)  [unwired: 9 in, 1 out]
                  n170 = xnode "Read/Write Control"("FPGA VI Reference In"=w656, "error in"=w655, "Rising(F)_or_Falling(T)"=w654) -> ()  [unwired: 2 out]
                  n171 = Select(t=myRIO_BRig_RT__Case_NonExp_stateList."UploadSettings_pre" ("Enum"), s=w663, f=myRIO_BRig_RT__Case_NonExp_stateList."Idle") -> (s? t:f=w661:T1)
                }
                frame "Cue_pre" {
                  n172 = call "BRig_RT__Case_Idle__State_Cue_pre__v2.vi"("input_dataExp"=w665, "input_dataMTrig"=w669) -> ("output_dataMTrig"=w668:u16[], "output_state"=w667:T1)  [unwired: 8 in]
                }
                frame "Cue" {
                  n173 = call "BRig_RT__Case_Idle__State_Cue__v2.vi"("input_cLick_R_prev"=w672, "input_cLick_R"=w673, "input_state"=w678, "input_cLick_L_prev"=w674, "input_cLick_L"=w675, "input_dataMTrig"=w679) -> ("output_dataMTrig"=w677:u16[], "output_state"=w676:T1)  [unwired: 4 in]
                }
                frame "RewardCalibration_pre" {
                  n174 = call "BRig_RT__Case_Idle__State_RewardCalibration_pre__v2.vi"("input_dataMTrig"=w681) -> ("output_dataMTrig"=w680:u16[])  [unwired: 26 in]
                }
                frame "RewardCalibration" {
                  n175 = call "BRig_RT__Case_Idle__State_RewardCalibration.vi"("input_state"=w686, "input_dataMTrig"=w688) -> ("output_dataMtrig"=w687:u16[], "output_state"=w685:T1)  [unwired: 8 in]
                }
                frame "TestConnection" {
                  n176 = local read "Host Password"() -> (w694:string)
                  n177 = local read "Host UserName"() -> (w695:string)
                  n178 = call "BRig_RT_comm_webdav_connect.vi"("input_password"=w694, "input_username"=w695) -> ("output_Iconnected"=w693:bool, "output_hSession"=w692:T4)  [unwired: 6 in, 2 out]
                  n179 = local write "comm_WebDAV_connect"(FALSE ("comm_WebDAV_connect")) -> ()
                  n180 = local write "comm_WebDAV"(w693) -> ()
                }
                frame "SendData" {
                  n181 = And(x=w704, y=w703) -> (x .and. y?=w702:bool)
                  n182 = case shown="True" w702 {
                    tunnel: w703 -> [_ w721]
                    tunnel: w709 -> [_ w720]
                    tunnel: w708 -> [_ w719]
                    tunnel: w706 -> [_ w717]
                    tunnel: w705 -> [_ w716]
                    frame False {
                      n183 = One Button Dialog(message="Unable to send data:\n Missing one or more\n connections") -> ()  [unwired: 1 in, 1 out]
                    }
                    frame True {
                      n184 = local read "Data Set Prefix"() -> (w722:string)
                      n185 = call "BRig_RT_comm_webdav_upload_all__v3.vi"("input_I_connected_webdav"=w721, "input_fileName_prefix"=w722, "input_hSession"=w720, "input_error"=w719, "input_True"=TRUE) -> ("output_nFilenames"=w723:i32, "output_arrFilenames"=w724:string[], "output_uploaded"=w725:bool[], "output_strCmd"=w718:string)  [unwired: 5 in, 2 out]
                      n186 = call "BRig_RT_comm_tcp_write_RTwrite.vi"("input_error"=w716, "input_packet"=w718, "input_hTCP"=w717) -> ()  [unwired: 5 in, 4 out]
                      n187 = call "BRig_RT_comm_webdav_upload_all_warnUser.vi"("input_n"=w723, "input_arrFilenames"=w724, "input_arrUploaded"=w725) -> ()  [unwired: 9 in]
                    }
                  }
                  n188 = local write "I_sendData"(FALSE ("I_sendData")) -> ()
                }
                frame "Get_FPGA_count_per_ms" {
                  # "Used to automatically determine how many FPGA cycles in 1 ms"
                  n189 = case shown="True" w738 {
                    selector: w738 -> [w740 _]
                    tunnel: w736 -> [_ w753]
                    tunnel: [w744 w753] -> w735
                    tunnel: w734 -> [w743 w751]
                    tunnel: w733 -> [w742 w750]
                    tunnel: [w741 w748] -> w728
                    tunnel: [w740 w747] -> w732
                    frame False {
                      n190 = Get Date/Time In Seconds() -> (seconds since 1Jan1904=w745:timestamp)
                      n191 = To Double Precision Float(number=w745) -> (double precision float=w744:dbl)
                      n192 = xnode "Read/Write Control"("FPGA VI Reference In"=w743, "error in"=w742, "timeTrial_trig"=TRUE ("timeTrial")) -> ("error out"=w741:errorcluster)  [unwired: 1 out]
                      n193 = local write "get_countPerMS"(w740) -> ()
                    }
                    frame True {
                      w749 = 1.0
                      # "units are\nseconds"
                      n194 = Get Date/Time In Seconds() -> (seconds since 1Jan1904=w754:timestamp)
                      n195 = To Double Precision Float(number=w754) -> (double precision float=w755:dbl)
                      n196 = Subtract(x=w755, y=w753) -> (x-y=w752:dbl)
                      n197 = Less Or Equal?(x=w749, y=w752) -> (x <= y?=w747:bool)
                      n198 = case shown="True" w747 {
                        tunnel: w751 -> [_ w768]
                        tunnel: w750 -> [w756 w767]
                        tunnel: w749 -> [_ w758]
                        tunnel: [w756 w757] -> w748
                        frame False {
                        }
                        frame True {
                          n199 = xnode "Read/Write Control"("FPGA VI Reference In"=w768, "error in"=w767) -> ("FPGA VI Reference Out"=w765:refnum<k20>, "error out"=w764:errorcluster, "timeTrial_count"=w759:u32)
                          n200 = Multiply(x=w758, y=1000.0) -> (x*y=w762:dbl)
                          n201 = To Double Precision Float(number=w759) -> (double precision float=w761:dbl)
                          n202 = Divide(x=w761, y=w762) -> (x/y=w763:dbl)
                          n203 = local write "FPGA_count2ms"(w763) -> ()
                          n204 = xnode "Read/Write Control"("FPGA VI Reference In"=w765, "error in"=w764, "timeTrial_trig"=FALSE ("timeTrial")) -> ("error out"=w757:errorcluster)  [unwired: 1 out]
                        }
                      }
                    }
                  }
                  n205 = Select(t=myRIO_BRig_RT__Case_NonExp_stateList."Idle" ("Enum"), s=w732, f=w730) -> (s? t:f=w729:T1)
                  n206 = local write "error out"(w728) -> ()
                }
                frame "End" {
                }
                frame "commTCP_connect" {
                  n207 = case shown="True" w785 {
                    tunnel: w784 -> [w795 w804]
                    tunnel: [w794 w800] -> w782
                    tunnel: [w793 w797] -> w774
                    tunnel: [w792 w798] -> w783
                    tunnel: w781 -> [_ w805]
                    frame False {
                      n208 = call "BRig_RT_comm_tcp_connect_RTwrite.vi"("input_error"=w795) -> ("output_error"=w792:errorcluster, "output_connected"=w793:bool, "output_hTCP"=w794:refnum<k5>)  [unwired: 8 in]
                    }
                    frame True {
                      n209 = call "BRig_RT_comm_tcp_write_RTwrite.vi"("input_error"=w804, "input_packet"="<test>", "input_hTCP"=w805) -> ("output_error"=w799:errorcluster, "output_I_NotDisconnected"=w796:bool, "output_I_write"=w802:bool, "output_hTCP"=w801:refnum<k5>)  [unwired: 5 in]
                      n210 = case shown="False" w802 {
                        selector: w802 -> [_ w816]
                        tunnel: w801 -> [w811 w818]
                        tunnel: [w806 w818] -> w800
                        tunnel: w799 -> [w810 w817]
                        tunnel: [w808 w817] -> w798
                        tunnel: [w807 w816] -> w797
                        tunnel: w796 -> [w812 _]
                        frame False {
                          n211 = case shown="True" w812 {
                            tunnel: w811 -> [_ w815]
                            tunnel: w810 -> [w813 w814]
                            tunnel: [w813 w814] -> w809
                            frame False {
                            }
                            frame True {
                              n212 = TCP Close Connection(connection ID=w815, error in (no error)=w814) -> ()  [unwired: 1 in, 2 out]
                            }
                          }
                          n213 = call "BRig_RT_comm_tcp_connect_RTwrite.vi"("input_error"=w809) -> ("output_error"=w808:errorcluster, "output_connected"=w807:bool, "output_hTCP"=w806:refnum<k5>)  [unwired: 8 in]
                        }
                        frame True {
                        }
                      }
                    }
                  }
                  n214 = local read "comm_TCP_connect"() -> (w778:bool)
                  n215 = Not(x=w778) -> (.not. x?=w777:bool)
                  n216 = Or(x=w777, y=w774) -> (x .or. y?=w776:bool)
                  n217 = case shown="True" w776 {
                    tunnel: [w789 myRIO_BRig_RT__Case_NonExp_stateList."Idle" ("Enum")] -> w780
                    tunnel: w779 -> [w789 _]
                    frame False {
                    }
                    frame True {
                      n218 = local write "comm_TCP_connect"(FALSE) -> ()
                    }
                  }
                  n219 = local write "comm_TCP"(w774) -> ()
                }
              }
              n220 = case shown="True" w397 {
                tunnel: [w455 w456] -> w400
                tunnel: [w454 w457] -> w399
                tunnel: [w453 w458] -> w398
                tunnel: w396 -> [w455 _]
                tunnel: w395 -> [w454 _]
                tunnel: w394 -> [w453 _]
                tunnel: w393 -> [_ w458]
                tunnel: w392 -> [_ w457]
                tunnel: w391 -> [_ w456]
                frame False {
                }
                frame True {
                }
              }
              n221 = case shown="True" w387 {
                tunnel: [w449 w450] -> w386
                tunnel: [w448 w451] -> w385
                tunnel: [w447 w452] -> w384
                tunnel: w388 -> [w449 _]
                tunnel: w389 -> [w448 _]
                tunnel: w390 -> [w447 _]
                tunnel: w382 -> [_ w452]
                tunnel: w381 -> [_ w451]
                tunnel: w383 -> [_ w450]
                frame False {
                }
                frame True {
                }
              }
              n222 = flat-sequence {
                tunnel: w420 -> [w462]
                tunnel: w418 -> [w460]
                tunnel: [w462] -> w424
                tunnel: [w461] -> w423
                tunnel: [w460] -> w422
                tunnel: [w459] -> w421
                tunnel: w417 -> [w459]
                tunnel: [w474] -> w419
                tunnel: w424 -> [w474]
                tunnel: w423 -> [w473]
                tunnel: w422 -> [w471]
                tunnel: w421 -> [w466]
                tunnel: [w465] -> w416
                frame #0 {
                  n223 = Get Date/Time In Seconds() -> (seconds since 1Jan1904=w461:timestamp)
                }
                frame #1 {
                  # "threshold"
                  # "delta T [ms]"
                  # "delta T [s]"
                  n224 = To Double Precision Float(number=w473) -> (double precision float=w472:dbl)
                  n225 = To Double Precision Float(number=w471) -> (double precision float=w470:dbl)
                  n226 = Subtract(x=w472, y=w470) -> (x-y=w469:dbl)
                  n227 = Multiply(x=w469, y=1000.0) -> (x*y=w464:dbl)
                  n228 = Greater?(x=w464, y=5.0) -> (0:w463:bool)
                  n229 = local write "Threshold"(w463) -> ()
                  n230 = local write "tLoop"(w464) -> ()
                  n231 = Or(x=w463, y=w466) -> (x .or. y?=w465:bool)
                }
              }
              n232 = local read "START"() -> (w441:bool)
              n233 = local read "STOP_abort"() -> (w440:bool)
              n234 = local read "Laser1_LED"() -> (w378:bool)
              n235 = local read "Laser2_LED"() -> (w377:bool)
              n236 = call "BRig_RT_panel_manualTriggering_v0,90.vi"("input_dataMTrig"=w405) -> ("output_Solenoid_R"=w408:bool, "output_Solenoid_L"=w409:bool, "output_dataMTrig"=w415:u16[], "output_Audio_L"=w410:bool, "output_Audio_R"=w411:bool, "output_CueLed"=w412:bool, "output_Laser_l1"=w413:bool, "output_Laser_l2"=w414:bool)  [unwired: 11 in]
              n237 = Or(x=w441, y=w440) -> (x .or. y?=w439:bool)
              n238 = Select(t=myRIO_BRig_RT__Case_NonExp_stateList."End" ("Enum"), s=w439, f=w438) -> (s? t:f=w437:T1)
              n239 = xnode "Read/Write Control"("FPGA VI Reference In"=w432, "error in"=w431, "A1_SR"=w408, "A3_SL"=w409, "audioTrigger_L"=w410, "audioTrigger_R"=w411, "LC_Laser_l1"=w413, "LC_Laser_l2"=w414, "CueLed_Event"=w412, "L1Led_ON"=w378, "L2Led_ON"=w377) -> ("FPGA VI Reference Out"=w443:refnum<k20>, "error out"=w420:errorcluster, "fpga_laser1"=w373:bool, "fpga_laser2"=w374:bool, "fpga_solenoid_L"=w375:bool, "fpga_solenoid_R"=w376:bool)
              n240 = local write "Laser1"(w373) -> ()
              n241 = local write "Laser2"(w374) -> ()
              n242 = local write "Solenoid L"(w375) -> ()
              n243 = local write "Solenoid R"(w376) -> ()
              n244 = node-c288() -> ()  [unwired: 1 in, 1 out]
            }
            n245 = node-c288(w368) -> ()  [unwired: 1 out]
            n246 = flat-sequence {
              tunnel: w362 -> [w372]
              tunnel: [w372] -> w361
              tunnel: w360 -> [w371]
              tunnel: [w371] -> w359
              frame #0 {
                w370 = FALSE
                n247 = local write "STOP_endBlock"(w370) -> ()
                n248 = local write "STOP_endTrial"(w370) -> ()
              }
            }
          }
          frame True {
            w888 = ".csv" ("string")
            w918 = ""
            w927 = u8 0
            w928 = u16 0 ("AudioLeft_phase_inc")
            w929 = FALSE
            # "Initialize data share\nbetween timed loop and\nTrial/Block Status loop"
            # "Initialize data share\nbetween timed loop\nand analog input loop"
            # "buffer_dataRT_stats"
            # "Clear local files"
            # "empty array"
            # "buffer_dataBlock"
            # "buffer_dataTrial"
            # "nColumns dataBlock"
            # "nColumns dataTrial"
            # "buffer_dataBlock"
            # "buffer_dataTrial"
            # "nColumns\ndataBlock"
            # "nColumns\ndataTrial"
            # "original dataExp and dataLC"
            # "dataLick"
            # "dataTrial"
            # "dataBlock"
            # "dataCurrent"
            # "arrTrig"
            # "time stamp"
            # "dummyState counter"
            # "dataTrial"
            # "dataLick"
            # "dataLC"
            # "dataLC"
            # "dataBlock"
            # "dataMTrig"
            # "dataMTrig"
            # "dataExp"
            # "dataExp"
            # "dataCurrent"
            # "state"
            n249 = flat-sequence {
              tunnel: [w1025] -> w858
              tunnel: [w1024] -> w862
              tunnel: [w1033] -> w876
              tunnel: [w1032] -> w875
              tunnel: [myRIO_BRig_RT__Case_Exp_stateList."Start1" ("Enum")] -> w874
              tunnel: [w1030] -> w873
              tunnel: [u16 0] -> w872
              tunnel: [w1028] -> w871
              tunnel: [w1027] -> w870
              tunnel: [w1026] -> w869
              tunnel: [w1035] -> w884
              tunnel: [w1036] -> w885
              tunnel: [w1037] -> w935
              tunnel: [w1038] -> w937
              tunnel: [w1039] -> w938
              tunnel: [w1040] -> w939
              tunnel: [w1041] -> w940
              tunnel: [w1042] -> w941
              tunnel: w876 -> [w1042]
              tunnel: w875 -> [w1041]
              tunnel: w874 -> [w1040]
              tunnel: w873 -> [w1039]
              tunnel: w872 -> [w1038]
              tunnel: w871 -> [w1037]
              tunnel: w870 -> [w1036]
              tunnel: w869 -> [w1035]
              tunnel: [w1034] -> w867
              frame #0 {
                n250 = call "BRig_dataBlock_init.vi"() -> ("output_nCol"=w1024:i32, "output_dataBlock"=w1026:u16[][])  [unwired: 10 in]
                n251 = call "BRig_dataCurrent_init.vi"() -> ("output_dataCurrent"=w1033:u16[])  [unwired: 11 in]
                n252 = call "BRig_dataLick_init.vi"() -> ("output_dataLick"=w1032:u16[][])  [unwired: 11 in]
                n253 = call "BRig_dataTrial_init.vi"() -> ("output_nCol"=w1025:i32, "output_dataTrial"=w1027:u16[][])  [unwired: 10 in]
                n254 = Get Date/Time In Seconds() -> (seconds since 1Jan1904=w1023:timestamp)
                n255 = To Double Precision Float(number=w1023) -> (double precision float=w1030:dbl)
                n256 = call "BRig_arrTrig_init.vi"() -> ("output_arrTrig"=w1028:bool[])  [unwired: 11 in]
              }
              frame #1 {
                w1034 = u32 2 ("milliseconds to wait")
                n257 = Wait (ms)(milliseconds to wait=w1034) -> ()  [unwired: 1 out]
              }
            }
            n258 = flat-sequence {
              tunnel: w864 -> [w1004]
              tunnel: [w1004] -> w863
              tunnel: w863 -> [w1013]
              tunnel: [w1011] -> w846
              tunnel: [w1010] -> w833
              tunnel: [w1007] -> w861
              tunnel: w862 -> [w1006]
              tunnel: w858 -> [w1005]
              tunnel: [w1013] -> w860
              tunnel: w860 -> [w1015]
              tunnel: [w1015] -> w859
              tunnel: w859 -> [w1021]
              tunnel: w858 -> [w1020]
              tunnel: [w1018] -> w853
              tunnel: [w1016] -> w856
              tunnel: [w1021] -> w857
              tunnel: [w1022] -> _
              tunnel: w857 -> [w1022]
              frame #0 {
                n259 = Wait (ms)(milliseconds to wait=w1004) -> ()  [unwired: 1 out]
              }
              frame #1 {
                w1008 = u16 0 ("element")
                n260 = Initialize Array(w1008, 8 ("dimension size")) -> (w1011:u16[])
                n261 = Initialize Array(w1008, 100 ("dimension size"), w1005) -> (w1010:u16[][])
                n262 = Initialize Array(w1008, 10 ("dimension size"), w1006) -> (w1007:u16[][])
              }
              frame #2 {
                n263 = Wait (ms)(milliseconds to wait=w1015) -> ()  [unwired: 1 out]
              }
              frame #3 {
                n264 = Increment(x=w1020) -> (x+1=w1017:i32)
                n265 = To Unsigned Long Integer(number=w1017) -> (unsigned 32bit integer=w1016:u32)
                n266 = Initialize Array(u16 0 ("element"), w1017) -> (w1018:u16[])
              }
              frame #4 {
                n267 = Wait (ms)(milliseconds to wait=w1022) -> ()  [unwired: 1 out]
              }
            }
            n268 = call "BRig_comm_webdav_myrioFolder.vi"() -> ("output_myrioFolder"=w889:string)  [unwired: 11 in]
            n269 = local write "stop_TimedLoop"(FALSE ("stop_TimedLoop")) -> ()
            n270 = RT FIFO Create(0:"dataTrialOrBlock" ("name (unnamed)"), 1:w853, 4:u32 40 ("size (10)"), 6:w856, 7:T8 {"read mode"=enum."blocking", "write mode"=enum."blocking"} ("r/w modes (polling,polling)")) -> (8:w855:refnum<k33>, 11:w854:errorcluster)  [unwired: 3 in, 1 out]
            n271 = RT FIFO Create(0:"dataAnalog" ("name (unnamed)"), 1:u16 0 ("element"), 4:u32 1000 ("size (10)")) -> (8:w841:refnum<k33>, 11:w840:errorcluster)  [unwired: 5 in, 1 out]
            n272 = Concatenate Strings(w889, "dataTrial" ("input_filename"), w888) -> (w890:string)
            n273 = Concatenate Strings(w889, "dataBlock" ("input_filename"), w888) -> (w891:string)
            n274 = String To Path(string=w890) -> (path=w894:path)
            n275 = String To Path(string=w891) -> (path=w886:path)
            n276 = flat-sequence {
              tunnel: [w1043] -> w868
              tunnel: w867 -> [w1043]
              tunnel: w868 -> [w1044]
              tunnel: [w1044] -> w865
              tunnel: w881 -> [w1047]
              tunnel: w834 -> [w1046]
              tunnel: [w1045] -> w866
              tunnel: w865 -> [w1045]
              tunnel: [w1051] -> _
              tunnel: w880 -> [w1051]
              tunnel: w879 -> [w1050]
              tunnel: w878 -> [w1049]
              tunnel: [w1048] -> w864
              tunnel: w866 -> [w1048]
              frame #0 {
                n277 = call "BRig_RT__Case_Exp__clearLocalFolder.vi"() -> ()  [unwired: 12 in]
              }
              frame #1 {
                n278 = Wait (ms)(milliseconds to wait=w1044) -> ()  [unwired: 1 out]
              }
              frame #2 {
                n279 = call "BRig_RT__Case_Exp__State_start__sendExpData_saveData.vi"("input_dataLC"=w1047, "input_dataExp"=w1046) -> ()  [unwired: 10 in]
              }
              frame #3 {
                n280 = call "BRig_RT__Case_Exp__State_start__sendExpData_uploadData__v2.vi"("input_error"=w1051, "input_hSession"=w1050, "input_connected"=w1049) -> ()  [unwired: 8 in, 1 out]
              }
            }
            n281 = call "BRig_RT__Case_Exp__comm_tcp__data_other.vi"("input_strState"=w918, "input_strAccum"=w918, "input_error"=w923, "input_hTCP"=w924, "input_I_connected_TCP"=w925) -> ("output_strAccum"=w919:string, "output_error"=w920:errorcluster, "output_hTCP"=w921:refnum<k5>, "output_I_connect_TCP"=w922:bool)  [unwired: 3 in]
            n282 = Initialize Array(u16 0 ("element"), 60 ("dimension size")) -> (w828:u16[])
            n283 = node-c288() -> (w947:T5)  [unwired: 4 in]
            n284 = timed-loop {
              timing: w947 -> [_]
              timing-out: [_] -> w946
              shift-right: [w1337] -> _
              shift-left: w939 -> [w1292]
              tunnel: w934 -> [w1381]
              tunnel: w933 -> [w1361]
              shift-right: [w1325] -> _
              shift-left: w945 -> [w1380]
              shift-right: [w1324] -> _
              shift-left: w944 -> [w1379]
              tunnel: [w1372] -> w926
              tunnel: [w1373] -> w943
              shift-right: [w1335] -> w914
              shift-left: w941 -> [w1309]
              shift-right: [w1378] -> w915
              shift-left: w834 -> [w1311]
              shift-right: [w1355] -> w917
              shift-left: w931 -> [w1312]
              shift-right: [w1376] -> _
              shift-left: w884 -> [w1377]
              shift-right: [w1374] -> w916
              shift-left: w881 -> [w1375]
              shift-right: [w1331] -> w913
              shift-left: w940 -> [w1338]
              shift-right: [w1371] -> _
              shift-left: w885 -> [w1310]
              tunnel: w938 -> [w1370]
              shift-right: [w1344] -> _
              shift-left: u16 0 -> [w1343]
              shift-right: [w1364] -> _
              shift-left: w937 -> [w1365]
              shift-right: [w1362] -> _
              shift-left: w935 -> [w1363]
              shift-right: [w1356] -> _
              shift-left: FALSE -> [w1358]
              shift-right: [w1300] -> w905
              shift-left: w922 -> [w1319]
              shift-right: [w1299] -> w904
              shift-left: w921 -> [w1318]
              shift-right: [w1297] -> w903
              shift-left: w920 -> [w1317]
              shift-right: [w1298] -> _
              shift-left: w919 -> [w1316]
              shift-right: [w1306] -> w910
              shift-left: w880 -> [w1306]
              shift-right: [w1308] -> w908
              shift-left: w878 -> [w1308]
              shift-right: [w1307] -> w909
              shift-left: w879 -> [w1307]
              shift-right: [w1305] -> _
              shift-left: _ -> [w1303]
              shift-right: [w1304] -> _
              shift-left: _ -> [w1302]
              tunnel: [w1301] -> w897
              tunnel: w855 -> [w1295]
              tunnel: w854 -> [w1294]
              tunnel: w853 -> [w1293]
              tunnel: w841 -> [w1291]
              tunnel: w840 -> [w1290]
              tunnel: w834 -> [w1289]
              stop <- w1301 stop-if-true
              # "send TCP message"
              # "dataCurrent"
              # "package\nanalog input\nand send\nto another loop"
              # "arrTrig"
              # "time stamp"
              # "dummyState counter"
              # "dataTrial"
              # "dataLC"
              # "dataBlock"
              # "dataExp"
              # "dataCurrent"
              # "state"
              # "iOccurrence"
              # "resetOccurrence?\ndataAnalog"
              # "dataLick"
              # "dataLick"
              # "dummyState counter"
              # "dummyState counter"
              # "iOccurrence"
              # "arrTrig"
              # "CueLed"
              # "LC_Laser_l2"
              # "LC_Event_l2"
              # "LC_Laser_l1"
              # "LC_Event_l1"
              # "iState\n(start and end)"
              # "manual triggering"
              # "dataTrial"
              # "dataBlock"
              # "dataExp"
              # "dataCurrent"
              # "time stamp"
              # "audio__L\naudio__R"
              # "dataLC"
              # "solenoid__R"
              # "solenoid__L"
              # "Did a lick occur?"
              # "Update lick counter"
              # "state"
              # "state"
              n285 = node-c288() -> ()  [unwired: 1 in, 1 out]
              n286 = local write "cState"(w1292) -> ()
              n287 = flat-sequence {
                tunnel: w1361 -> [w1382]
                tunnel: [w1383] -> w1359
                tunnel: [w1382] -> w1360
                frame #0 {
                  n288 = Get Date/Time In Seconds() -> (seconds since 1Jan1904=w1383:timestamp)
                }
              }
              n289 = xnode "Read/Write Control"("FPGA VI Reference In"=w1381, "error in"=w1360) -> ("FPGA VI Reference Out"=w1367:refnum<k20>, "error out"=w1366:errorcluster, "A2_LickL"=w1325:u32, "A4_LickR"=w1324:u32)
              n290 = local write "A2"(w1325) -> ()
              n291 = local write "A4"(w1324) -> ()
              n292 = Greater?(x=w1325, y=w1380) -> (0:w1333:bool)
              n293 = Greater?(x=w1324, y=w1379) -> (0:w1332:bool)
              n294 = Or(x=w1333, y=w1332) -> (x .or. y?=w1334:bool)
              n295 = case shown="\"endBlock\"" w1292 {
                selector: w1292 -> [_ _ _ _ _ _ _ _ _ _ _ _ _ _ w1691 w1707 _ w1736 _ _ w1815 w1842 _ w1868 _ w1912 _ w2009 _ w2028 _ _ w2180 w2190 _ _ _ _ w2326 _ w2350 w2381 w2402 w2427 _ w2492 w2502 _]
                tunnel: [myRIO_BRig_RT__Case_Exp_stateList."Start2" ("Enum") myRIO_BRig_RT__Case_Exp_stateList."Start3" ("Enum") myRIO_BRig_RT__Case_Exp_stateList."saveSettings1" ("Enum") myRIO_BRig_RT__Case_Exp_stateList."initBlock" ("Enum") myRIO_BRig_RT__Case_Exp_stateList."initTrial_LC_ENL1" ("Enum") myRIO_BRig_RT__Case_Exp_stateList."initTrial" ("Enum") myRIO_BRig_RT__Case_Exp_stateList."initTrial2" ("Enum") myRIO_BRig_RT__Case_Exp_stateList."setSettings_Laser" ("Enum") myRIO_BRig_RT__Case_Exp_stateList."ENL1_pre" ("Enum") myRIO_BRig_RT__Case_Exp_stateList."initTrial_LC_Cue1" ("Enum") myRIO_BRig_RT__Case_Exp_stateList."initTrial_LC_Sel" ("Enum") myRIO_BRig_RT__Case_Exp_stateList."initTrial4" ("Enum") w1670 w1681 w1689 w1705 myRIO_BRig_RT__Case_Exp_stateList."ENL1Penalty" ("Enum") w1734 w1749 w1772 w1814 w1841 myRIO_BRig_RT__Case_Exp_stateList."Cue1Penalty" ("Enum") w1869 w1885 w1907 myRIO_BRig_RT__Case_Exp_stateList."SelectReward" ("Enum") w2008 myRIO_BRig_RT__Case_Exp_stateList."SelectRewardPost" ("Enum") w2027 myRIO_BRig_RT__Case_Exp_stateList."SelectWrong" ("Enum") myRIO_BRig_RT__Case_Exp_stateList."SelectTimeout" ("Enum") w2179 w2189 myRIO_BRig_RT__Case_Exp_stateList."saveData_dataTrial" ("Enum") w2224 w2268 w2315 w2326 myRIO_BRig_RT__Case_Exp_stateList."initBlock" ("Enum") w2348 w2382 w2401 w2426 myRIO_BRig_RT__Case_Exp_stateList."FreeReward" ("Enum") w2490 w2500 myRIO_BRig_RT__Case_Exp_stateList."FreeRewardPost" ("Enum")] -> w1337
                tunnel: w1334 -> [_ _ _ _ _ _ _ _ _ _ _ _ w1671 w1682 w1690 w1706 _ _ w1750 w1773 w1816 w1843 _ _ _ _ _ _ _ _ _ _ _ _ _ _ _ _ _ _ _ _ _ _ _ _ _ _]
                tunnel: w1333 -> [_ _ _ _ _ _ _ _ _ _ _ _ _ _ _ _ _ _ _ _ _ _ _ _ w1878 w1908 _ _ _ _ _ _ _ _ _ _ _ _ _ _ _ _ _ _ _ _ _ _]
                tunnel: w1332 -> [_ _ _ _ _ _ _ _ _ _ _ _ _ _ _ _ _ _ _ _ _ _ _ _ w1877 w1909 _ _ _ _ _ _ _ _ _ _ _ _ _ _ _ _ _ _ _ _ _ _]
                tunnel: w1309 -> [w1393 w1399 w1441 w1468 w1471 w1544 w1558 w1575 w1604 w1629 w1639 w1656 w1669 w1680 w1698 w1714 w1725 w1733 w1751 w1774 w1817 w1844 w1861 w1867 w1888 w1905 w1948 w2006 w2018 w2026 w2056 w2127 w2178 w2188 w2204 w2230 w2276 w2305 w2325 w2332 w2351 w2384 w2400 w2417 w2462 w2488 w2499 w2510]
                tunnel: w1311 -> [w1384 w1398 w1431 w1466 w1472 w1543 w1546 w1574 w1598 w1628 w1638 w1648 w1663 w1676 w1701 w1717 w1724 w1741 w1742 w1754 w1820 w1847 w1854 w1875 w1876 w1904 w1934 w2007 w2016 w2033 w2039 w2110 w2185 w2195 w2196 w2222 w2257 w2288 w2316 w2329 w2353 w2386 w2412 w2432 w2445 w2493 w2503 w2509]
                tunnel: [w1393 w1399 w1441 w1468 w1471 w1542 w1557 w1570 w1604 w1632 w1646 w1655 w1662 w1683 w1697 w1713 w1726 w1732 w1743 w1769 w1800 w1827 w1860 w1866 w1884 w1906 w1921 w2010 w2017 w2024 w2050 w2121 w2176 w2187 w2206 w2230 w2276 w2305 w2325 w2332 w2351 w2384 w2400 w2417 w2468 w2489 w2498 w2508] -> w1336
                tunnel: [w1384 w1398 w1430 w1466 w1472 w1543 w1546 w1574 w1598 w1628 w1638 w1648 w1663 w1676 w1701 w1717 w1724 w1741 w1742 w1754 w1820 w1847 w1854 w1875 w1876 w1904 w1934 w2007 w2016 w2033 w2039 w2110 w2185 w2195 w2196 w2219 w2264 w2291 w2316 w2329 w2353 w2386 w2412 w2432 w2446 w2493 w2503 w2509] -> w1378
                tunnel: [_ _ _ _ _ _ _ _ _ _ _ _ _ _ _ _ _ _ _ _ _ _ _ _ _ _ _ w2000 _ _ _ _ _ _ _ _ _ _ _ _ _ _ _ _ _ w2482 _ _] -> w1321
                tunnel: [_ _ _ _ _ _ _ _ _ _ _ _ _ _ _ _ _ _ _ _ _ _ _ _ _ _ _ w1999 _ _ _ _ _ _ _ _ _ _ _ _ _ _ _ _ _ w2483 _ _] -> w1320
                tunnel: w1377 -> [w1392 w1396 w1439 w1470 w1503 w1540 w1562 w1590 w1615 w1634 w1645 w1653 w1673 w1685 w1700 w1716 w1721 w1739 w1753 w1776 w1819 w1846 w1859 w1872 w1894 w1916 w1947 w2011 w2022 w2031 w2054 w2125 w2183 w2194 w2200 w2231 w2266 w2307 w2323 w2331 w2333 w2387 w2410 w2430 w2471 w2495 w2505 w2517]
                tunnel: [w1392 w1396 w1439 w1470 w1503 w1539 w1561 w1590 w1615 w1634 w1645 w1653 w1673 w1685 w1700 w1716 w1721 w1739 w1753 w1776 w1819 w1846 w1859 w1872 w1894 w1916 w1946 w2011 w2022 w2031 w2053 w2124 w2183 w2194 w2200 w2231 w2266 w2307 w2323 w2331 w2333 w2387 w2410 w2430 w2471 w2495 w2505 w2517] -> w1376
                tunnel: w1375 -> [w1385 w1397 w1440 w1469 w1498 w1545 w1569 w1591 w1616 w1633 w1640 w1654 w1672 w1684 w1699 w1715 w1722 w1740 w1752 w1775 w1818 w1845 w1858 w1874 w1893 w1917 w1923 w1998 w2013 w2032 w2034 w2105 w2184 w2193 w2213 w2221 w2277 w2309 w2324 w2328 w2352 w2385 w2411 w2431 w2472 w2496 w2506 w2518]
                tunnel: [w1385 w1397 w1440 w1469 w1498 w1545 w1569 w1591 w1616 w1633 w1640 w1654 w1672 w1684 w1699 w1715 w1722 w1740 w1752 w1775 w1818 w1845 w1858 w1874 w1893 w1917 w1923 w1998 w2013 w2032 w2034 w2105 w2184 w2193 w2213 w2220 w2277 w2309 w2324 w2328 w2352 w2385 w2411 w2431 w2472 w2496 w2506 w2518] -> w1374
                tunnel: [_ _ _ _ _ _ _ _ _ _ _ _ _ _ _ _ _ _ _ _ _ _ _ _ _ _ _ _ _ _ _ _ _ _ _ _ _ _ TRUE _ _ _ _ _ _ _ _ _] -> w1339
                tunnel: [_ _ _ _ _ _ _ _ _ _ _ _ _ _ _ _ _ _ _ _ w1802 w1829 _ _ _ _ _ _ _ _ _ _ _ _ _ _ _ _ _ _ _ _ _ _ _ _ _ _] -> w1369
                tunnel: [_ _ _ _ _ _ _ _ _ _ _ _ _ _ _ _ _ _ _ _ w1801 w1828 _ _ _ _ _ _ _ _ _ _ _ _ _ _ _ _ _ _ _ _ _ _ _ _ _ _] -> w1368
                tunnel: w1310 -> [w1390 w1395 w1437 w1467 w1502 w1538 w1565 w1592 w1608 w1635 w1644 w1652 w1668 w1679 w1688 w1704 w1718 w1738 w1748 w1771 w1805 w1832 w1856 w1871 w1892 w1896 w1945 w1997 w2012 w2030 w2052 w2123 w2182 w2192 w2212 w2229 w2275 w2306 w2321 w2330 w2337 w2364 w2409 w2429 w2466 w2494 w2504 w2516]
                tunnel: [w1390 w1395 w1437 w1467 w1502 w1537 w1560 w1576 w1602 w1631 w1643 w1651 w1667 w1678 w1687 w1703 w1718 w1738 w1747 w1770 w1804 w1831 w1856 w1871 w1892 w1895 w1919 w1997 w2012 w2030 w2049 w2120 w2182 w2192 w2211 w2229 w2275 w2306 w2321 w2330 w2337 w2364 w2409 w2429 w2466 w2494 w2504 w2516] -> w1371
                tunnel: w1370 -> [_ _ _ _ _ _ _ _ _ _ _ _ _ _ _ _ _ _ _ _ _ _ _ _ _ _ _ _ _ _ _ _ _ _ w2205 _ _ _ _ _ _ _ _ _ _ _ _ _]
                tunnel: w1367 -> [w1389 _ _ _ w1499 w1532 w1568 w1596 w1613 _ _ w1659 _ _ _ _ _ _ _ w1756 w1806 w1833 _ _ w1890 w1915 w1944 _ _ _ _ _ _ _ w2208 _ _ _ w2319 _ _ _ _ _ w2452 _ _ _]
                tunnel: w1366 -> [w1388 _ _ _ w1500 w1531 w1559 w1595 w1612 _ _ w1658 _ _ _ _ _ _ _ w1755 w1807 w1834 _ _ w1891 w1914 w1943 _ _ _ _ _ _ _ w2207 _ _ _ w2318 _ _ _ _ _ w2451 _ _ _]
                tunnel: [_ _ _ _ _ _ _ _ _ _ _ _ _ _ w1696 w1712 _ _ _ _ w1812 w1839 _ _ w1883 w1902 _ w1993 _ _ _ _ _ _ _ _ _ _ _ _ _ _ _ _ _ _ _ _] -> w1345
                tunnel: [_ _ _ _ _ _ _ _ _ _ _ _ _ _ w1695 w1711 _ _ _ _ w1811 w1838 _ _ w1882 w1901 _ w1994 _ _ _ _ _ _ _ _ _ _ _ _ _ _ _ _ _ _ _ _] -> w1326
                tunnel: [_ _ _ _ _ _ _ _ TRUE ("Recording") _ _ _ _ _ _ _ _ _ _ _ _ _ _ _ _ _ _ _ _ _ _ _ _ _ _ _ _ _ _ _ _ _ _ _ _ _ _ _] -> w1342
                tunnel: w1365 -> [_ _ _ _ _ _ _ _ _ _ _ _ _ _ _ _ _ _ _ _ _ _ _ _ _ _ _ _ _ _ _ _ _ _ _ _ _ _ _ _ w2349 w2380 w2407 w2414 _ _ _ _]
                tunnel: [_ _ _ _ _ _ _ _ _ _ _ _ _ _ _ _ _ _ _ _ _ _ _ _ _ _ _ _ _ _ _ _ _ _ _ _ _ _ _ _ w2347 w2379 w2405 w2415 _ _ _ _] -> w1364
                tunnel: w1363 -> [_ _ _ _ w1479 _ _ _ w1609 w1636 w1642 w1650 w1665 w1675 w1692 w1708 w1719 w1737 w1746 w1768 w1813 w1840 w1855 w1870 w1879 w1903 _ _ _ _ _ _ _ _ _ _ _ _ _ _ _ _ _ _ _ _ _ _]
                tunnel: [_ _ _ _ w1479 _ _ w1577 w1609 w1630 w1641 w1649 w1664 w1674 w1692 w1708 w1719 w1737 w1745 w1767 w1813 w1840 w1855 w1870 w1879 w1903 _ _ _ _ _ _ _ _ _ _ _ _ _ _ _ _ _ _ _ _ _ _] -> w1362
                tunnel: [_ _ _ _ _ _ _ _ _ _ _ _ _ _ w1694 w1710 _ _ _ _ w1810 w1837 _ _ w1881 w1900 _ w1995 _ _ _ _ _ _ _ _ _ _ _ _ _ _ _ _ _ _ _ _] -> w1349
                tunnel: [_ _ _ _ _ _ _ _ _ _ _ _ _ _ w1693 w1709 _ _ _ _ w1809 w1836 _ _ w1880 w1899 _ w1996 _ _ _ _ _ _ _ _ _ _ _ _ _ _ _ _ _ _ _ _] -> w1350
                tunnel: [_ _ _ _ _ _ _ _ _ _ _ _ _ _ _ _ _ _ _ _ w1803 w1830 _ _ _ _ _ _ _ _ _ _ _ _ _ _ _ _ _ _ _ _ _ _ _ _ _ _] -> w1352
                tunnel: [_ _ "<S,S>" ("string") _ _ _ _ _ w1603 _ _ _ _ _ _ _ _ _ _ _ _ _ _ _ _ _ w1918 _ _ _ w2041 w2112 _ _ w2203 _ _ w2301 _ _ _ _ _ _ _ _ _ _] -> w1315
                tunnel: w1312 -> [_ _ _ _ _ _ _ _ _ _ _ _ _ _ _ _ _ _ _ _ _ _ _ _ _ _ _ _ _ _ _ _ _ _ _ _ _ _ _ _ _ _ _ _ w2457 _ _ _]
                tunnel: w1308 -> [_ _ _ _ _ _ _ _ _ _ _ _ _ _ _ _ _ _ _ _ _ _ _ _ _ _ _ _ _ _ _ _ _ _ _ _ _ w2300 _ _ _ _ _ _ _ _ _ _]
                tunnel: w1307 -> [_ _ _ _ _ _ _ _ _ _ _ _ _ _ _ _ _ _ _ _ _ _ _ _ _ _ _ _ _ _ _ _ _ _ _ _ _ _ _ _ _ _ _ _ _ _ _ _]
                tunnel: w1306 -> [_ _ _ _ _ _ _ _ _ _ _ _ _ _ _ _ _ _ _ _ _ _ _ _ _ _ _ _ _ _ _ _ _ _ _ _ _ _ _ _ _ _ _ _ _ _ _ _]
                tunnel: [_ _ _ _ _ _ _ _ _ _ _ _ _ _ _ _ _ _ _ _ _ _ _ _ _ _ _ _ _ _ _ _ _ _ _ w2223 _ _ _ _ _ _ _ _ _ _ _ _] -> w1305
                tunnel: [_ _ _ _ _ _ _ _ _ _ _ _ _ _ _ _ _ _ _ _ _ _ _ _ _ _ _ _ _ _ _ _ _ _ _ w2228 _ _ _ _ _ _ _ _ _ _ _ _] -> w1304
                tunnel: w1303 -> [_ _ _ _ _ _ _ _ _ _ _ _ _ _ _ _ _ _ _ _ _ _ _ _ _ _ _ _ _ _ _ _ _ _ _ w2227 _ _ _ _ _ _ _ _ _ _ _ _]
                tunnel: w1302 -> [_ _ _ _ _ _ _ _ _ _ _ _ _ _ _ _ _ _ _ _ _ _ _ _ _ _ _ _ _ _ _ _ _ _ _ w2218 _ _ _ _ _ _ _ _ _ _ _ _]
                tunnel: w1295 -> [_ _ w1414 w1452 _ w1521 w1553 _ _ _ _ _ _ _ _ _ _ _ _ _ _ _ _ _ _ _ w1932 _ _ _ w2044 w2115 _ _ _ _ _ _ _ _ w2344 w2367 _ _ w2437 _ _ _]
                tunnel: w1294 -> [_ _ w1413 w1451 _ w1522 w1552 _ _ _ _ _ _ _ _ _ _ _ _ _ _ _ _ _ _ _ w1931 _ _ _ w2042 w2113 _ _ _ _ _ _ _ _ w2343 w2366 _ _ w2436 _ _ _]
                tunnel: w1293 -> [_ _ _ _ _ _ _ _ _ _ _ _ _ _ _ _ _ _ _ _ _ _ _ _ _ _ _ _ _ _ _ _ _ _ _ _ _ _ _ _ w2341 w2365 _ _ _ _ _ _]
                tunnel: w1289 -> [_ _ _ _ _ _ _ _ _ _ _ _ _ _ _ _ _ _ _ _ w1799 w1826 _ _ _ _ _ _ _ _ _ _ _ _ _ _ _ _ _ _ _ _ _ _ _ _ _ _]
                frame "Start1", Default {
                  w1387 = FALSE ("SelectionState")
                  n296 = xnode "Read/Write Control"("FPGA VI Reference In"=w1389, "error in"=w1388, "SelectionState"=w1387, "LR_reward_Laser_l1"=w1387, "LR_wrong_Laser_l1"=w1387, "LR_reward_Event_l1"=w1387, "LR_wrong_Event_l1"=w1387, "Left(F)_or_Right(T)"=w1387, "SelectionState"=w1387, "LR_reward_Laser_l2"=w1387, "LR_wrong_laser_l2"=w1387, "LR_reward_Event_l2"=w1387, "LR_wrong_Event_l2"=w1387, "LC_Event_l1"=w1387, "LC_Laser_l1"=w1387, "LC_Laser_l2"=w1387, "LC_Event_l2"=w1387, "CueLed_Event"=w1387) -> ("error out"=w1386:errorcluster)  [unwired: 1 out]
                  n297 = local write "error out"(w1386) -> ()
                }
                frame "Start2" {
                }
                frame "Start3" {
                  w1402 = u16 3 ("element")
                  w1400 = u16 0 ("element")
                  w1427 = u16 0 ("new element/subarray")
                  w1432 = 0.0 ("BTPR_avg_L")
                  w1435 = FALSE ("SolenoidReward")
                  w1433 = u16 0 ("BTPR_block")
                  w1436 = u16 0 ("nRewards_cur")
                  # "Goal:\nPrepare dataCurrent"
                  n298 = call "BRig_dataExp_FreeReward_c_L.vi"() -> ("output_FreeReward_c_L"=w1429:i32)  [unwired: 11 in]
                  n299 = call "BRig_dataExp_FreeReward_c_R.vi"() -> ("output_FreeReward_c_R"=w1428:i32)  [unwired: 11 in]
                  n300 = local write "nRewards_cur"(w1436) -> ()
                  n301 = local write "nRewards_total"(w1436) -> ()
                  n302 = local write "nRewards_Left"(w1436) -> ()
                  n303 = local write "nRewards_Right"(w1436) -> ()
                  n304 = local write "BUR_target"(w1436) -> ()
                  n305 = local write "TpB_target"(w1436) -> ()
                  n306 = local write "iBlock"(w1436) -> ()
                  n307 = local write "iTrial"(w1436) -> ()
                  n308 = local write "nTrial"(w1436) -> ()
                  n309 = local write "SolenoidReward"(w1435) -> ()
                  n310 = local write "allReward_L"(w1435) -> ()
                  n311 = local write "allReward_R"(w1435) -> ()
                  n312 = local write "BTPR_avg_L"(w1432) -> ()
                  n313 = local write "BTPR_avg_R"(w1432) -> ()
                  n314 = local write "T2R_avg_L"(w1432) -> ()
                  n315 = local write "T2R_avg_R"(w1432) -> ()
                  n316 = Replace Array Subset(array=w1431, new element #1=w1427, index #1=w1429, new element #2=w1427, index #2=w1428) -> (w1430:u16[])
                  n317 = call "BRig_dataRT_stats__T2R_cur.vi"() -> ("output_T2R_cur"=w1426:i32)  [unwired: 11 in]
                  n318 = call "BRig_dataRT_stats__BTPR_cur.vi"() -> ("output_BTPR_cur"=w1425:i32)  [unwired: 11 in]
                  n319 = call "BRig_dataRT_stats__T2R_avg_L.vi"() -> ("output_T2R_avg_L__x100"=w1420:i32)  [unwired: 11 in]
                  n320 = call "BRig_dataRT_stats__T2R_avg_R.vi"() -> ("output_T2R_avg_R__x100"=w1419:i32)  [unwired: 11 in]
                  n321 = call "BRig_dataRT_stats__BTPR_avg_L.vi"() -> ("output_BTPR_avg_L__x100"=w1424:i32)  [unwired: 11 in]
                  n322 = call "BRig_dataRT_stats__BTPR_avg_R.vi"() -> ("output_BTPR_avg_R__x100"=w1416:i32)  [unwired: 11 in]
                  n323 = call "BRig_dataRT_stats__nReward.vi"() -> ("output_nReward"=w1411:i32)  [unwired: 11 in]
                  n324 = call "BRig_dataRT_stats__nReward_left.vi"() -> ("output_nReward_left"=w1410:i32)  [unwired: 11 in]
                  n325 = call "BRig_dataRT_stats__nReward_right.vi"() -> ("output_nReward_right"=w1409:i32)  [unwired: 11 in]
                  n326 = local write "FreeReward_c_L"(w1427) -> ()
                  n327 = local write "FreeReward_c_R"(w1427) -> ()
                  n328 = local write "BTPR_block"(w1433) -> ()
                  n329 = local write "T2R_block"(w1433) -> ()
                  n330 = call "BRig_dataRT_stats__FreeReward_c_L.vi"() -> ("output_FreeReward_c_L"=w1405:i32)  [unwired: 11 in]
                  n331 = call "BRig_dataRT_stats__FreeReward_c_R.vi"() -> ("output_FreeReward_c_R"=w1404:i32)  [unwired: 11 in]
                  n332 = To Unsigned Word Integer(number=w1420) -> (unsigned 16bit integer=w1421:u16)
                  n333 = To Unsigned Word Integer(number=w1426) -> (unsigned 16bit integer=w1423:u16)
                  n334 = To Unsigned Word Integer(number=w1419) -> (unsigned 16bit integer=w1418:u16)
                  n335 = To Unsigned Word Integer(number=w1425) -> (unsigned 16bit integer=w1422:u16)
                  n336 = To Unsigned Word Integer(number=w1424) -> (unsigned 16bit integer=w1417:u16)
                  n337 = To Unsigned Word Integer(number=w1416) -> (unsigned 16bit integer=w1415:u16)
                  n338 = To Unsigned Word Integer(number=w1411) -> (unsigned 16bit integer=w1408:u16)
                  n339 = To Unsigned Word Integer(number=w1410) -> (unsigned 16bit integer=w1407:u16)
                  n340 = To Unsigned Word Integer(number=w1409) -> (unsigned 16bit integer=w1406:u16)
                  n341 = To Unsigned Word Integer(number=w1405) -> (unsigned 16bit integer=w1403:u16)
                  n342 = To Unsigned Word Integer(number=w1404) -> (unsigned 16bit integer=w1401:u16)
                  n343 = Build Array(w1402, w1423, w1400, w1402, w1422, w1400, w1402, w1421, w1400, w1402, w1418, w1400, w1402, w1417, w1400, w1402, w1415, w1400, w1402, w1408, w1400, w1402, w1407, w1400, w1402, w1406, w1400, w1402, w1403, w1400, w1402, w1401, w1400) -> (w1412:u16[])
                  n344 = RT FIFO Write(0:w1414, 1:w1412, 3:w1413) -> ()  [unwired: 2 in, 4 out]
                }
                frame "saveSettings1" {
                  w1454 = u16 3 ("element")
                  w1453 = u16 0 ("element")
                  n345 = call "BRig_dataRT_stats__nTrial.vi"() -> ("output_nTrial"=w1450:i32)  [unwired: 11 in]
                  n346 = call "BRig_dataRT_stats__iTrial.vi"() -> ("output_iTrial"=w1449:i32)  [unwired: 11 in]
                  n347 = call "BRig_dataRT_stats__iBlock.vi"() -> ("output_iBlock"=w1448:i32)  [unwired: 11 in]
                  n348 = call "BRig_dataRT_stats__nReward_cur.vi"() -> ("output_nReward_cur"=w1447:i32)  [unwired: 11 in]
                  n349 = call "BRig_dataRT_stats__TpB_target.vi"() -> ("output_TpB_target"=w1446:i32)  [unwired: 11 in]
                  n350 = call "BRig_dataRT_stats__BUR_target.vi"() -> ("output_BUR_target"=w1445:i32)  [unwired: 11 in]
                  n351 = call "BRig_dataRT_stats__DAB_nReward_HighProb.vi"() -> ("output_DAB_nReward_HighProb"=w1444:i32)  [unwired: 11 in]
                  n352 = call "BRig_dataRT_stats__DAB_nReward_LowProb.vi"() -> ("output_DAB_nReward_LowProb"=w1443:i32)  [unwired: 11 in]
                  n353 = call "BRig_dataRT_stats__DAB_nTimeout.vi"() -> ("output_DAB_nTimeout"=w1442:i32)  [unwired: 11 in]
                  n354 = To Unsigned Word Integer(number=w1448) -> (unsigned 16bit integer=w1462:u16)
                  n355 = To Unsigned Word Integer(number=w1450) -> (unsigned 16bit integer=w1464:u16)
                  n356 = To Unsigned Word Integer(number=w1447) -> (unsigned 16bit integer=w1461:u16)
                  n357 = To Unsigned Word Integer(number=w1449) -> (unsigned 16bit integer=w1463:u16)
                  n358 = To Unsigned Word Integer(number=w1446) -> (unsigned 16bit integer=w1460:u16)
                  n359 = To Unsigned Word Integer(number=w1445) -> (unsigned 16bit integer=w1459:u16)
                  n360 = To Unsigned Word Integer(number=w1444) -> (unsigned 16bit integer=w1457:u16)
                  n361 = To Unsigned Word Integer(number=w1443) -> (unsigned 16bit integer=w1456:u16)
                  n362 = To Unsigned Word Integer(number=w1442) -> (unsigned 16bit integer=w1455:u16)
                  n363 = Build Array(w1454, w1464, w1453, w1454, w1463, w1453, w1454, w1462, w1453, w1454, w1461, w1453, w1454, w1460, w1453, w1454, w1459, w1453, w1454, w1457, w1453, w1454, w1456, w1453, w1454, w1455, w1453) -> (w1458:u16[])
                  n364 = RT FIFO Write(0:w1452, 1:w1458, 3:w1451) -> ()  [unwired: 2 in, 4 out]
                }
                frame "setSettings_Laser" {
                  n365 = call "BRig_dataExp_LED_baseline_Cue.vi"() -> ("output_LED_baseline_Cue"=w1488:i32)  [unwired: 11 in]
                  n366 = call "BRig_dataExp_LED_baseline_l1.vi"() -> ("output_LED_baseline_l1"=w1489:i32)  [unwired: 11 in]
                  n367 = call "BRig_dataExp_LED_baseline_l2.vi"() -> ("output_LED_baseline_l2"=w1487:i32)  [unwired: 11 in]
                  n368 = call "BRig_dataExp_I_trialUntilReward.vi"() -> ("output_I_trialUntilReward"=w1474:i32)  [unwired: 11 in]
                  n369 = local read "FPGA_count2ms"() -> (w1497:dbl)
                  n370 = call "BRig_RT__Case_Exp__State_setLaserSettings__v2.vi"("input_FPGA_count2ms"=w1497, "input_dataExp"=w1472, "input_dataLC"=w1498) -> ("output_LR_nTotal_l1"=w1496:u32, "output_LR_nTotal_l2"=w1495:u32, "output_LR_reward_nDelay_l1"=w1494:u32, "output_LR_wrong_nDelay_l1"=w1493:u32, "output_LR_reward_nDelay_l2"=w1492:u32, "output_LR_wrong_nDelay_l2"=w1491:u32)  [unwired: 11 in]
                  n371 = Index Array(array=w1472, index #1=w1488, index #2=w1489, index #3=w1487, index #4=w1474) -> (element #1=w1486:u16, element #2=w1485:u16, element #3=w1484:u16, element #4=w1473:u16)  [unwired: 1 in, 1 out]
                  n372 = Not Equal To 0?(x=w1485) -> (x != 0?=w1482:bool)
                  n373 = Not Equal To 0?(x=w1486) -> (x != 0?=w1483:bool)
                  n374 = Not Equal To 0?(x=w1484) -> (x != 0?=w1481:bool)
                  n375 = Not Equal To 0?(x=w1473) -> (x != 0?=w1480:bool)
                  n376 = local read "LaserFiber_V_l1"() -> (w1478:dbl)
                  n377 = local read "LaserFiber_V_l2"() -> (w1476:dbl)
                  n378 = call "myRIO__convert__Voltage_to_FPGAvalue.vi"("input_voltage"=w1478) -> ("output_PortA"=w1477:u16)  [unwired: 9 in, 1 out]
                  n379 = call "myRIO__convert__Voltage_to_FPGAvalue.vi"("input_voltage"=w1476) -> ("output_PortA"=w1475:u16)  [unwired: 9 in, 1 out]
                  n380 = xnode "Read/Write Control"("FPGA VI Reference In"=w1499, "error in"=w1500, "LR_reward_nTotal_l1"=w1496, "LR_wrong_nTotal_l1"=w1496, "LR_reward_nTotal_l2"=w1495, "LR_wrong_nTotal_l2"=w1495, "LR_reward_nDelay_l1"=w1494, "LR_wrong_nDelay_l1"=w1493, "LR_reward_nDelay_l2"=w1492, "LR_wrong_nDelay_l2"=w1491, "CueLed_Baseline"=w1483, "L1Led_Baseline"=w1482, "L2Led_Baseline"=w1481, "ignoreWrong"=w1480, "AnaOut0_Pair"=w1477, "AnaOut1_Pair"=w1475) -> ("error out"=→"error out":errorcluster)  [unwired: 1 out]
                }
                frame "initBlock" {
                  w1504 = u16 0 ("element")
                  w1507 = u16 3
                  w1524 = u16 0 ("BTPR_block")
                  n381 = local write "nRewards_cur"(u16 0 ("nRewards_cur")) -> ()
                  n382 = local write "BTPR_block"(w1524) -> ()
                  n383 = local write "T2R_block"(w1524) -> ()
                  n384 = call "BRig_RT__Case_Exp__State_initBlock__v17.vi"("input_dataCurrent"=w1544, "input_dataExp"=w1543, "input_dataBlock"=w1540, "input_dataTrial"=w1538) -> ("output_iSpout"=w1529:u16, "output_speaker_amp_R"=w1533:u16, "output_iBlock"=w1513:u16, "output_speaker_freq_R"=w1534:u8, "output_BUR_target"=w1514:u16, "output_speaker_amp_L"=w1535:u16, "output_TpB_target"=w1515:u16, "output_speaker_freq_L"=w1536:u8, "output_dataCurrent"=w1542:u16[], "output_dataBlock"=w1539:u16[][], "output_dataTrial"=w1537:u16[][])  [unwired: 5 in]
                  n385 = Type Cast(type=enum16{"Left", "Right"}."Left", x=w1529) -> (*(type *) &x=w1526:enum16{"Left", "Right"})
                  n386 = Not Equal To 0?(x=w1529) -> (x != 0?=w1525:bool)
                  n387 = call "BRig_dataRT_stats__TpB_target.vi"() -> ("output_TpB_target"=w1516:i32)  [unwired: 11 in]
                  n388 = call "BRig_dataRT_stats__BUR_target.vi"() -> ("output_BUR_target"=w1517:i32)  [unwired: 11 in]
                  n389 = call "BRig_dataRT_stats__iBlock.vi"() -> ("output_iBlock"=w1518:i32)  [unwired: 11 in]
                  n390 = call "BRig_dataRT_stats__T2R_cur.vi"() -> ("output_T2R_cur"=w1511:i32)  [unwired: 11 in]
                  n391 = call "BRig_dataRT_stats__BTPR_cur.vi"() -> ("output_BTPR_cur"=w1510:i32)  [unwired: 11 in]
                  n392 = call "BRig_dataRT_stats__nReward_cur.vi"() -> ("output_nReward_cur"=w1506:i32)  [unwired: 11 in]
                  n393 = local write "cSpout"(w1526) -> ()
                  n394 = xnode "Read/Write Control"("FPGA VI Reference In"=w1532, "error in"=w1531, "Left(F)_or_Right(T)"=w1525, "audioFreq_L_kHz"=w1536, "audioAmp_L"=w1535, "audioFreq_R_kHz"=w1534, "audioAmp_R"=w1533) -> ("error out"=w1530:errorcluster)  [unwired: 1 out]
                  n395 = To Unsigned Word Integer(number=w1511) -> (unsigned 16bit integer=w1509:u16)
                  n396 = To Unsigned Word Integer(number=w1506) -> (unsigned 16bit integer=w1505:u16)
                  n397 = To Unsigned Word Integer(number=w1516) -> (unsigned 16bit integer=w1523:u16)
                  n398 = To Unsigned Word Integer(number=w1517) -> (unsigned 16bit integer=w1520:u16)
                  n399 = To Unsigned Word Integer(number=w1518) -> (unsigned 16bit integer=w1519:u16)
                  n400 = To Unsigned Word Integer(number=w1510) -> (unsigned 16bit integer=w1508:u16)
                  n401 = local write "error out"(w1530) -> ()
                  n402 = local write "iBlock"(w1513) -> ()
                  n403 = local write "BUR_target"(w1514) -> ()
                  n404 = local write "TpB_target"(w1515) -> ()
                  n405 = Build Array(w1507, w1523, w1515, w1507, w1520, w1514, w1507, w1519, w1513, w1507, w1509, w1504, w1507, w1508, w1504, w1507, w1505, w1504) -> (w1512:u16[])
                  n406 = RT FIFO Write(0:w1521, 1:w1512, 3:w1522) -> ()  [unwired: 2 in, 4 out]
                }
                frame "initTrial" {
                  w1549 = u16 3
                  n407 = xnode "Read/Write Control"("FPGA VI Reference In"=w1568, "error in"=w1559, "SelectionState"=FALSE) -> ("error out"=w1567:errorcluster)  [unwired: 1 out]
                  n408 = call "BRig_RT__Case_Exp__State_initTrial__v18.vi"("input_dataCurrent"=w1558, "input_dataBlock"=w1562, "input_dataTrial"=w1565, "input_dataExp"=w1546) -> ("output_iTrial"=w1547:u16, "output_nTrial"=w1548:u16, "output_SolenoidReward"=w1564:bool, "output_dataCurrent"=w1557:u16[], "output_dataBlock"=w1561:u16[][], "output_dataTrial"=w1560:u16[][])  [unwired: 6 in]
                  n409 = call "BRig_dataRT_stats__nTrial.vi"() -> ("output_nTrial"=w1551:i32)  [unwired: 11 in]
                  n410 = call "BRig_dataRT_stats__iTrial.vi"() -> ("output_iTrial"=w1550:i32)  [unwired: 11 in]
                  n411 = local write "iTrial"(w1547) -> ()
                  n412 = local write "nTrial"(w1548) -> ()
                  n413 = local write "SolenoidReward"(w1564) -> ()
                  n414 = To Unsigned Word Integer(number=w1551) -> (unsigned 16bit integer=w1556:u16)
                  n415 = To Unsigned Word Integer(number=w1550) -> (unsigned 16bit integer=w1554:u16)
                  n416 = local write "error out"(w1567) -> ()
                  n417 = Build Array(w1549, w1556, w1548, w1549, w1554, w1547) -> (w1555:u16[])
                  n418 = RT FIFO Write(0:w1553, 1:w1555, 3:w1552) -> ()  [unwired: 2 in, 4 out]
                }
                frame "initTrial2" {
                  n419 = call "BRig_RT__Case_Exp__State_initTrial2__v17.vi"("input_dataCurrent"=w1575, "input_dataTrial"=w1592, "input_dataExp"=w1574, "input_dataBlock"=w1590, "input_dataLC"=w1591) -> ("output_L_Wrong_Laser_l2"=w1582:bool, "output_L_Wrong_Event_l2"=w1583:bool, "output_L_Power_l1"=w1581:dbl, "output_L_Reward_Laser_l2"=w1584:bool, "output_L_Power_l2"=w1580:dbl, "output_L_Reward_Event_l2"=w1585:bool, "output_dataCurrent"=w1570:u16[], "output_dataTrial"=w1576:u16[][], "output_L_Reward_Event_l1"=w1589:bool, "output_L_Reward_Laser_l1"=w1588:bool, "output_L_Wrong_Event_l1"=w1587:bool, "output_L_Wrong_Laser_l1"=w1586:bool)  [unwired: 3 in]
                  n420 = local write "L_Power_l1"(w1581) -> ()
                  n421 = call "myRIO__convert__Voltage_to_FPGAvalue.vi"("input_voltage"=w1581) -> ("output_PortC"=w1578:i16)  [unwired: 9 in, 1 out]
                  n422 = local write "L_Power_l2"(w1580) -> ()
                  n423 = call "myRIO__convert__Voltage_to_FPGAvalue.vi"("input_voltage"=w1580) -> ("output_PortC"=w1579:i16)  [unwired: 9 in, 1 out]
                  n424 = xnode "Read/Write Control"("FPGA VI Reference In"=w1596, "error in"=w1595, "AnaOut_0"=w1578, "AnaOut_1"=w1579, "LR_reward_Event_l1"=w1589, "LR_reward_Laser_l1"=w1588, "LR_wrong_Event_l1"=w1587, "LR_wrong_Laser_l1"=w1586, "LR_reward_Event_l2"=w1585, "LR_reward_Laser_l2"=w1584, "LR_wrong_Event_l2"=w1583, "LR_wrong_laser_l2"=w1582) -> ("error out"=w1593:errorcluster)  [unwired: 1 out]
                  n425 = local write "error out"(w1593) -> ()
                  n426 = call "BRig_dataCurrent_DAB_flipLR.vi"() -> ("output_DAB_flipLR"=w1573:i32)  [unwired: 11 in]
                  n427 = call "BRig_arrTrig_init.vi"() -> ("output_arrTrig"=w1577:bool[])  [unwired: 11 in]
                  n428 = Index Array(array=w1570, index=w1573) -> (element=w1572:u16)
                  n429 = Not Equal To 0?(x=w1572) -> (x != 0?=w1571:bool)
                  n430 = local write "DAB_flipLR"(w1571) -> ()
                }
                frame "initTrial4" {
                  # "Dual Armed Bandit?"
                  # "resetOccurrence?\ndataAnalog"
                  n431 = local read "FPGA_count2ms"() -> (w1605:dbl)
                  n432 = local read "lick_Rising(F)_or_Falling(T)"() -> (w1601:bool)
                  n433 = call "BRig_dataExp_I_anySelect.vi"() -> ("output_I_anySelect"=w1600:i32)  [unwired: 11 in]
                  n434 = Index Array(array=w1598, index=w1600) -> (element=w1599:u16)
                  n435 = local read "Recording"() -> (w1607:bool)
                  n436 = call "BRig_RT_comm_tcp_write_RTwrite__RunState_Trial_start.vi"("input_dataCurrent"=w1604) -> ("output_strCmd"=w1603:string)  [unwired: 10 in]
                  n437 = Not Equal To 0?(x=w1599) -> (x != 0?=w1597:bool)
                  n438 = call "BRig_RT__Case_Exp__State_initTrial4.vi"("input_Recording"=w1607, "input_FPGA_count2ms"=w1605, "input_dataTrial"=w1608) -> ("output_Solenoid_nTotal"=w1606:u32, "output_dataTrial"=w1602:u16[][])  [unwired: 7 in]
                  n439 = case shown="False" w1597 {
                    tunnel: w1613 -> [w1622 w1627]
                    tunnel: w1612 -> [w1621 w1626]
                    tunnel: [w1620 w1625] -> w1611
                    tunnel: w1607 -> [w1619 w1624]
                    tunnel: w1606 -> [w1618 _]
                    tunnel: w1601 -> [w1617 w1623]
                    frame False {
                      n440 = xnode "Read/Write Control"("FPGA VI Reference In"=w1622, "error in"=w1621, "Solenoid_nTotal_L"=w1618, "Solenoid_nTotal_R"=w1618, "A6_Act"=w1619, "Rising(F)_or_Falling(T)"=w1617) -> ("error out"=w1620:errorcluster)  [unwired: 1 out]
                    }
                    frame True {
                      n441 = xnode "Read/Write Control"("FPGA VI Reference In"=w1627, "error in"=w1626, "A6_Act"=w1624, "Rising(F)_or_Falling(T)"=w1623) -> ("error out"=w1625:errorcluster)  [unwired: 1 out]
                    }
                  }
                  n442 = local write "error out"(w1611) -> ()
                }
                frame "initTrial_LC_ENL1" {
                  n443 = call "BRig_RT__Case_Exp__State_initTrial__LC_ENL__v18.vi"("input_arrTrig"=w1636, "input_dataTrial"=w1635, "input_dataExp"=w1628, "input_dataLC"=w1633, "input_dataCurrent"=w1629) -> ("output_dataTrial"=w1631:u16[][], "output_dataCurrent"=w1632:u16[], "output_arrTrig"=w1630:bool[])  [unwired: 4 in]
                }
                frame "initTrial_LC_Cue1" {
                  n444 = call "BRig_RT__Case_Exp__State_initTrial__LC_Cue__v18.vi"("input_arrTrig"=w1642, "input_dataTrial"=w1644, "input_dataExp"=w1638, "input_dataLC"=w1640, "input_dataCurrent"=w1639) -> ("output_dataTrial"=w1643:u16[][], "output_dataCurrent"=w1646:u16[], "output_arrTrig"=w1641:bool[])  [unwired: 4 in]
                }
                frame "initTrial_LC_Sel" {
                  n445 = call "BRig_RT__Case_Exp__State_initTrial__LC_Select__v18.vi"("input_arrTrig"=w1650, "input_dataTrial"=w1652, "input_dataExp"=w1648, "input_dataLC"=w1654, "input_dataCurrent"=w1656) -> ("output_dataTrial"=w1651:u16[][], "output_dataCurrent"=w1655:u16[], "output_arrTrig"=w1649:bool[])  [unwired: 4 in]
                  n446 = xnode "Read/Write Control"("FPGA VI Reference In"=w1659, "error in"=w1658, "A6_Act"=FALSE) -> ("error out"=w1660:errorcluster)  [unwired: 1 out]
                  n447 = local write "error out"(w1660) -> ()
                }
                frame "ENL1_pre" {
                  n448 = call "BRig_RT__Case_Exp__State_ENLPre__v4.vi"("input_arrTrig"=w1665, "input_ENL2"=FALSE, "input_I_lick"=w1671, "input_dataExp"=w1663, "input_dataTrial"=w1668, "input_dataCurrent"=w1669) -> ("output_arrTrig"=w1664:bool[], "output_dataTrial"=w1667:u16[][], "output_dataCurrent"=w1662:u16[], "output_state"=w1670:T2)  [unwired: 2 in]
                }
                frame "ENL2_pre" {
                  n449 = call "BRig_RT__Case_Exp__State_ENLPre__v4.vi"("input_arrTrig"=w1675, "input_ENL2"=TRUE, "input_I_lick"=w1682, "input_dataExp"=w1676, "input_dataTrial"=w1679, "input_dataCurrent"=w1680) -> ("output_arrTrig"=w1674:bool[], "output_dataTrial"=w1678:u16[][], "output_dataCurrent"=w1683:u16[], "output_state"=w1681:T2)  [unwired: 2 in]
                }
                frame "ENL1" {
                  n450 = call "BRig_RT__Case_Exp__State_ENL__v3.vi"("input_dataCurrent"=w1698, "input_dataTrial"=w1688, "input_ENL2"=FALSE, "input_arrTrig"=w1692, "input_state"=w1691, "I_lick"=w1690) -> ("output_l2_laserOn"=w1693:bool, "output_l2_laserEvent"=w1694:bool, "output_l1_laserOn"=w1695:bool, "output_state"=w1689:T2, "output_l1_laserEvent"=w1696:bool, "output_dataCurrent"=w1697:u16[], "output_dataTrial"=w1687:u16[][])  [unwired: 7 in]
                }
                frame "ENL2" {
                  n451 = call "BRig_RT__Case_Exp__State_ENL__v3.vi"("input_dataCurrent"=w1714, "input_dataTrial"=w1704, "input_ENL2"=TRUE, "input_arrTrig"=w1708, "input_state"=w1707, "I_lick"=w1706) -> ("output_l2_laserOn"=w1709:bool, "output_l2_laserEvent"=w1710:bool, "output_l1_laserOn"=w1711:bool, "output_state"=w1705:T2, "output_l1_laserEvent"=w1712:bool, "output_dataCurrent"=w1713:u16[], "output_dataTrial"=w1703:u16[][])  [unwired: 7 in]
                }
                frame "ENL1Penalty_pre" {
                  n452 = call "BRig_dataCurrent_c_generic.vi"() -> ("output_count_generic"=w1730:i32)  [unwired: 11 in]
                  n453 = call "BRig_dataCurrent_T_generic.vi"() -> ("output_T_generic"=w1728:i32)  [unwired: 11 in]
                  n454 = call "BRig_dataExp_T_ENLPenalty.vi"() -> ("output_ENL_penalty"=w1723:i32)  [unwired: 11 in]
                  n455 = Index Array(array=w1724, index=w1723) -> (element=w1727:u16)
                  n456 = Replace Array Subset(array=w1725, new element #1=u16 0 ("new element/subarray"), index #1=w1730, new element #2=w1727, index #2=w1728) -> (w1726:u16[])
                }
                frame "ENL1Penalty" {
                  n457 = call "BRig_RT__Case_Exp__generic__incrementCountTilThreshold.vi"("input_dataCurrent"=w1733) -> ("output_dataCurrent"=w1732:u16[], "output_underThreshold"=w1731:bool)  [unwired: 9 in]
                  n458 = Select(t=w1736, s=w1731, f=myRIO_BRig_RT__Case_Exp_stateList."ENL1_pre" ("Enum")) -> (s? t:f=w1734:T2)
                }
                frame "Cue1_pre" {
                  n459 = call "BRig_RT__Case_Exp__State_CuePre__v5.vi"("input_dataCurrent"=w1751, "input_dataTrial"=w1748, "input_dataExp"=w1742, "input_Cue2"=FALSE ("input_ENL2"), "input_I_lick"=w1750, "input_arrTrig"=w1746) -> ("output_state"=w1749:T2, "output_arrTrig"=w1745:bool[], "output_dataCurrent"=w1743:u16[], "output_dataTrial"=w1747:u16[][])  [unwired: 10 in]
                }
                frame "Cue2_pre" {
                  # "Two cues?"
                  n460 = call "BRig_dataExp_I_Cue2.vi"() -> ("output_I_Cue2"=w1765:i32)  [unwired: 11 in]
                  n461 = call "BRig_dataExp_Audio_pattern_R.vi"() -> ("output_Audio_sp__R"=w1762:i32)  [unwired: 11 in]
                  n462 = call "BRig_dataExp_Audio_amp_R.vi"() -> ("output_Audio_amp__R"=w1761:i32)  [unwired: 11 in]
                  n463 = call "BRig_dataExp_Audio_freq_R.vi"() -> ("output_Audio_freq__R"=w1760:i32)  [unwired: 11 in]
                  n464 = Index Array(array=w1754, index #1=w1765, index #2=w1762, index #3=w1761, index #4=w1760) -> (element #1=w1764:u16, element #2=w1757:u16, element #3=w1758:u16, element #4=w1759:u16)
                  n465 = call "BRig_RT__Case_Exp__State_CuePre__v5.vi"("input_dataCurrent"=w1774, "input_dataTrial"=w1771, "input_dataExp"=w1754, "input_Cue2"=TRUE ("input_ENL2"), "input_I_lick"=w1773, "input_arrTrig"=w1768) -> ("output_state"=w1772:T2, "output_arrTrig"=w1767:bool[], "output_dataCurrent"=w1769:u16[], "output_dataTrial"=w1770:u16[][])  [unwired: 10 in]
                  n466 = Not Equal To 0?(x=w1764) -> (x != 0?=w1763:bool)
                  n467 = case shown="True" w1763 {
                    tunnel: w1759 -> [_ w1786]
                    tunnel: w1758 -> [_ w1785]
                    tunnel: w1757 -> [_ w1784]
                    tunnel: w1756 -> [_ w1783]
                    tunnel: w1755 -> [_ w1782]
                    frame False {
                    }
                    frame True {
                      n468 = To Unsigned Byte Integer(number=w1786) -> (unsigned 8bit integer=w1787:u8)
                      n469 = case shown="0, Default" w1784 {
                        tunnel: w1785 -> [w1791 w1794 w1796]
                        tunnel: w1787 -> [w1790 w1795 w1797]
                        tunnel: [w1791 u16 0 ("Numeric") w1796] -> w1781
                        tunnel: [w1790 u8 0 w1797] -> w1780
                        tunnel: [u8 0 w1795 w1797] -> w1778
                        tunnel: [u16 0 ("Numeric") w1794 w1796] -> w1779
                        frame 0, Default {
                          # "left only"
                        }
                        frame 1 {
                          # "right only"
                        }
                        frame 2 {
                          # "left and right"
                        }
                      }
                      n470 = xnode "Read/Write Control"("FPGA VI Reference In"=w1783, "error in"=w1782, "audioFreq_L_kHz"=w1780, "audioAmp_L"=w1781, "audioFreq_R_kHz"=w1778, "audioAmp_R"=w1779) -> ("error out"=w1777:errorcluster)  [unwired: 1 out]
                      n471 = local write "error out"(w1777) -> ()
                    }
                  }
                }
                frame "Cue1" {
                  n472 = call "BRig_RT__Case_Exp__State_Cue__v3.vi"("input_dataCurrent"=w1817, "input_dataTrial"=w1805, "input_dataExp"=w1799, "input_Cue2"=FALSE, "input_arrTrig"=w1813, "input_state"=w1815, "I_lick"=w1816) -> ("output_l2_laserOn"=w1809:bool, "output_l2_laserEvent"=w1810:bool, "output_SelectionState"=w1808:bool, "output_l1_laserOn"=w1811:bool, "output_state"=w1814:T2, "output_l1_laserEvent"=w1812:bool, "output_dataCurrent"=w1800:u16[], "output_dataTrial"=w1804:u16[][], "output_CueLed"=w1803:bool, "output_Audio_L"=w1802:bool, "output_Audio_R"=w1801:bool)  [unwired: 2 in]
                  n473 = case shown="True" w1808 {
                    selector: w1808 -> [_ w1823]
                    tunnel: w1807 -> [_ w1822]
                    tunnel: w1806 -> [_ w1821]
                    frame False {
                    }
                    frame True {
                      n474 = xnode "Read/Write Control"("FPGA VI Reference In"=w1821, "error in"=w1822, "SelectionState"=w1823) -> ("error out"=w1824:errorcluster)  [unwired: 1 out]
                      n475 = local write "error out"(w1824) -> ()
                    }
                  }
                }
                frame "Cue2" {
                  n476 = call "BRig_RT__Case_Exp__State_Cue__v3.vi"("input_dataCurrent"=w1844, "input_dataTrial"=w1832, "input_dataExp"=w1826, "input_Cue2"=TRUE, "input_arrTrig"=w1840, "input_state"=w1842, "I_lick"=w1843) -> ("output_l2_laserOn"=w1836:bool, "output_l2_laserEvent"=w1837:bool, "output_SelectionState"=w1835:bool, "output_l1_laserOn"=w1838:bool, "output_state"=w1841:T2, "output_l1_laserEvent"=w1839:bool, "output_dataCurrent"=w1827:u16[], "output_dataTrial"=w1831:u16[][], "output_CueLed"=w1830:bool, "output_Audio_L"=w1829:bool, "output_Audio_R"=w1828:bool)  [unwired: 2 in]
                  n477 = case shown="True" w1835 {
                    selector: w1835 -> [_ w1850]
                    tunnel: w1834 -> [_ w1849]
                    tunnel: w1833 -> [_ w1848]
                    frame False {
                    }
                    frame True {
                      n478 = xnode "Read/Write Control"("FPGA VI Reference In"=w1848, "error in"=w1849, "SelectionState"=w1850) -> ("error out"=w1851:errorcluster)  [unwired: 1 out]
                      n479 = local write "error out"(w1851) -> ()
                    }
                  }
                }
                frame "Cue1Penalty_pre" {
                  n480 = call "BRig_dataCurrent_c_generic.vi"() -> ("output_count_generic"=w1864:i32)  [unwired: 11 in]
                  n481 = call "BRig_dataCurrent_T_generic.vi"() -> ("output_T_generic"=w1862:i32)  [unwired: 11 in]
                  n482 = call "BRig_dataExp_T_CuePenalty.vi"() -> ("output_T_CuePenalty"=w1853:i32)  [unwired: 11 in]
                  n483 = Index Array(array=w1854, index=w1853) -> (element=w1852:u16)
                  n484 = Replace Array Subset(array=w1861, new element #1=u16 0 ("new element/subarray"), index #1=w1864, new element #2=w1852, index #2=w1862) -> (w1860:u16[])
                }
                frame "Cue1Penalty" {
                  n485 = call "BRig_RT__Case_Exp__generic__incrementCountTilThreshold.vi"("input_dataCurrent"=w1867) -> ("output_dataCurrent"=w1866:u16[], "output_underThreshold"=w1865:bool)  [unwired: 9 in]
                  n486 = Select(t=w1868, s=w1865, f=myRIO_BRig_RT__Case_Exp_stateList."ENL1_pre" ("Enum")) -> (s? t:f=w1869:T2)
                }
                frame "Selection_pre" {
                  n487 = xnode "Read/Write Control"("FPGA VI Reference In"=w1890, "error in"=w1891) -> ("error out"=w1889:errorcluster, "SelectReward"=w1886:bool, "SelectWrong"=w1887:bool)  [unwired: 1 out]
                  n488 = call "BRig_RT__Case_Exp__State_SelectPre__v2.vi"("input_dataCurrent"=w1888, "input_SelectWrong"=w1887, "input_SelectReward"=w1886, "input_dataExp"=w1876, "input_LickL"=w1878, "input_LickR"=w1877, "input_arrTrig"=w1879) -> ("output_state"=w1885:T2, "output_dataCurrent"=w1884:u16[], "output_l1_laserEvent"=w1883:bool, "output_l1_laserOn"=w1882:bool, "output_l2_laserOn"=w1880:bool, "output_l2_laserEvent"=w1881:bool)  [unwired: 3 in]
                  n489 = local write "error out"(w1889) -> ()
                }
                frame "Selection" {
                  n490 = xnode "Read/Write Control"("FPGA VI Reference In"=w1915, "error in"=w1914) -> ("error out"=w1913:errorcluster, "SelectReward"=w1910:bool, "SelectWrong"=w1911:bool)  [unwired: 1 out]
                  n491 = call "BRig_RT__Case_Exp__State_Selection__v2.vi"("input_state"=w1912, "input_dataCurrent"=w1905, "input_dataTrial"=w1896, "input_dataExp"=w1904, "input_arrTrig"=w1903, "input_SelectWrong"=w1911, "input_SelectReward"=w1910, "input_LickR"=w1909, "input_LickL"=w1908) -> ("output_l2_laserOn"=w1899:bool, "output_l2_laserEvent"=w1900:bool, "output_l1_laserOn"=w1901:bool, "output_l1_laserEvent"=w1902:bool, "output_state"=w1907:T2, "output_dataCurrent"=w1906:u16[], "output_dataTrial"=w1895:u16[][], "output_allReward_L"=w1897:bool, "output_allReward_R"=w1898:bool)  [unwired: 2 in]
                  n492 = local write "allReward_L"(w1897) -> ()
                  n493 = local write "allReward_R"(w1898) -> ()
                  n494 = local write "error out"(w1913) -> ()
                }
                frame "SelectReward_pre" {
                  # "Dual Armed\nBandit?"
                  n495 = call "BRig_dataExp_I_anySelect.vi"() -> ("output_I_anySelect"=w1936:i32)  [unwired: 11 in]
                  n496 = Index Array(array=w1934, index=w1936) -> (element=w1935:u16)
                  n497 = call "BRig_RT__Case_Exp__State_RewardPre__v11.vi"("input_dataCurrent"=w1948, "input_dataExp"=w1934, "input_dataBlock"=w1947, "input_dataTrial"=w1945, "input_dataLC"=w1923) -> ("output_T_Reward"=w1942:u16, "output_c_nReward_total_R"=w1927:u16, "output_c_nReward_total_L"=w1926:u16, "output_dataCurrent"=w1921:u16[], "output_DAB_L=L"=w1924:bool, "output_DAB_R=HighPorb"=w1925:bool, "output_dataBlock"=w1946:u16[][], "output_c_nReward_total"=w1929:u16, "output_nReward"=w1928:u16, "output_dataTrial"=w1919:u16[][])  [unwired: 1 in]
                  n498 = local read "FPGA_count2ms"() -> (w1941:dbl)
                  n499 = Not Equal To 0?(x=w1935) -> (x != 0?=w1933:bool)
                  n500 = case shown="True" w1933 {
                    tunnel: [w1955 w1985] -> w1930
                    tunnel: w1929 -> [w1954 w1982]
                    tunnel: w1928 -> [w1953 w1981]
                    tunnel: w1927 -> [w1952 w1984]
                    tunnel: w1926 -> [w1951 w1983]
                    tunnel: w1925 -> [_ w1975]
                    tunnel: w1924 -> [_ w1976]
                    tunnel: w1921 -> [w1950 w1970]
                    tunnel: [w1950 w1968] -> w1920
                    frame False {
                      w1959 = u16 3
                      n501 = call "BRig_dataRT_stats__nReward_left.vi"() -> ("output_nReward_left"=w1956:i32)  [unwired: 11 in]
                      n502 = call "BRig_dataRT_stats__nReward_right.vi"() -> ("output_nReward_right"=w1957:i32)  [unwired: 11 in]
                      n503 = call "BRig_dataRT_stats__nReward_cur.vi"() -> ("output_nReward_cur"=w1958:i32)  [unwired: 11 in]
                      n504 = call "BRig_dataRT_stats__nReward.vi"() -> ("output_nReward"=w1961:i32)  [unwired: 11 in]
                      n505 = To Unsigned Word Integer(number=w1956) -> (unsigned 16bit integer=w1964:u16)
                      n506 = To Unsigned Word Integer(number=w1957) -> (unsigned 16bit integer=w1963:u16)
                      n507 = To Unsigned Word Integer(number=w1958) -> (unsigned 16bit integer=w1962:u16)
                      n508 = To Unsigned Word Integer(number=w1961) -> (unsigned 16bit integer=w1960:u16)
                      n509 = local write "nRewards_Right"(w1952) -> ()
                      n510 = local write "nRewards_Left"(w1951) -> ()
                      n511 = local write "nRewards_cur"(w1953) -> ()
                      n512 = local write "nRewards_total"(w1954) -> ()
                      n513 = Build Array(w1959, w1964, w1951, w1959, w1963, w1952, w1959, w1962, w1953, w1959, w1960, w1954) -> (w1955:u16[])
                    }
                    frame True {
                      w1987 = u16 3
                      n514 = call "BRig_dataRT_stats__nReward_left.vi"() -> ("output_nReward_left"=w1980:i32)  [unwired: 11 in]
                      n515 = call "BRig_dataRT_stats__nReward_right.vi"() -> ("output_nReward_right"=w1979:i32)  [unwired: 11 in]
                      n516 = call "BRig_dataRT_stats__DAB_nReward_HighProb.vi"() -> ("output_DAB_nReward_HighProb"=w1978:i32)  [unwired: 11 in]
                      n517 = call "BRig_dataRT_stats__DAB_nReward_LowProb.vi"() -> ("output_DAB_nReward_LowProb"=w1977:i32)  [unwired: 11 in]
                      n518 = call "BRig_dataRT_stats__nReward_cur.vi"() -> ("output_nReward_cur"=w1986:i32)  [unwired: 11 in]
                      n519 = call "BRig_dataRT_stats__nReward.vi"() -> ("output_nReward"=w1989:i32)  [unwired: 11 in]
                      n520 = Select(t=w1980, s=w1976, f=w1979) -> (s? t:f=w1973:i32)
                      n521 = Select(t=w1978, s=w1975, f=w1977) -> (s? t:f=w1974:i32)
                      n522 = To Unsigned Word Integer(number=w1973) -> (unsigned 16bit integer=w1992:u16)
                      n523 = To Unsigned Word Integer(number=w1974) -> (unsigned 16bit integer=w1991:u16)
                      n524 = To Unsigned Word Integer(number=w1986) -> (unsigned 16bit integer=w1990:u16)
                      n525 = To Unsigned Word Integer(number=w1989) -> (unsigned 16bit integer=w1988:u16)
                      n526 = local write "nRewards_cur"(w1981) -> ()
                      n527 = local write "nRewards_total"(w1982) -> ()
                      n528 = call "BRig_dataCurrent_s_Selection.vi"() -> ("output_s_Selection"=w1969:i32)  [unwired: 11 in]
                      n529 = call "BRig_dataCurrent_I_giveReward.vi"() -> ("output_I_giveReward"=w1972:i32)  [unwired: 11 in]
                      n530 = Build Array(w1987, w1992, w1983, w1987, w1991, w1984, w1987, w1990, w1981, w1987, w1988, w1982) -> (w1985:u16[])
                      n531 = Index Array(array=w1970, index=w1972) -> (element=w1966:u16)
                      n532 = Not Equal To 0?(x=w1966) -> (x != 0?=w1971:bool)
                      n533 = local write "SolenoidReward"(w1971) -> ()
                      n534 = Subtract(x=u16 2 ("new element/subarray"), y=w1966) -> (x-y=w1965:u16)
                      n535 = Replace Array Subset(array=w1970, new element=w1965, index=w1969) -> (w1968:u16[])
                    }
                  }
                  n536 = To Double Precision Float(number=w1942) -> (double precision float=w1940:dbl)
                  n537 = Multiply(x=w1941, y=w1940) -> (x*y=w1938:dbl)
                  n538 = Round Toward +Infinity(x=w1938) -> (ceil(x): smallest int >= x=w1939:dbl)
                  n539 = To Unsigned Long Integer(number=w1939) -> (unsigned 32bit integer=w1937:u32)
                  n540 = RT FIFO Write(0:w1932, 1:w1930, 3:w1931) -> ()  [unwired: 2 in, 4 out]
                  n541 = xnode "Read/Write Control"("FPGA VI Reference In"=w1944, "error in"=w1943, "Solenoid_nTotal_L"=w1937, "Solenoid_nTotal_R"=w1937) -> ()  [unwired: 2 out]
                  n542 = call "BRig_RT_comm_tcp_write_RTwrite__RunState_Trial_selResult__v3.vi"("input_dataTrial"=w1919, "iReward_or_iError"=TRUE, "input_dataCurrent"=w1920) -> ("output_strCmd"=w1918:string)  [unwired: 8 in]
                }
                frame "SelectReward" {
                  n543 = call "BRig_dataCurrent_c_generic.vi"() -> ("output_count_generic"=w2005:i32)  [unwired: 11 in]
                  n544 = Index Array(array=w2006, index=w2005) -> (element=w2004:u16)
                  n545 = call "BRig_RT__Case_Exp__State_Reward.vi"("input_dataCurrent"=w2006, "input_state"=w2009, "input_dataTrial"=w1997, "input_dataLC"=w1998, "input_dataExp"=w2007) -> ("output_state"=w2008:T2, "output_dataCurrent"=w2010:u16[], "output_L_event_l1"=w1993:bool, "output_L_trig_l1"=w1994:bool, "output__L"=w2003:bool, "output_L_trig_l2"=w1996:bool, "output_L_event_l2"=w1995:bool, "output__R"=w2002:bool)  [unwired: 3 in]
                  n546 = Equal To 0?(x=w2004) -> (x = 0?=w2001:bool)
                  n547 = And(x=w2003, y=w2001) -> (x .and. y?=w2000:bool)
                  n548 = And(x=w2002, y=w2001) -> (x .and. y?=w1999:bool)
                }
                frame "SelectRewardPost_pre" {
                  n549 = call "BRig_dataExp_T_RewardPost.vi"() -> ("output_T_RewardPost"=w2015:i32)  [unwired: 11 in]
                  n550 = call "BRig_dataCurrent_c_generic.vi"() -> ("output_count_generic"=w2021:i32)  [unwired: 11 in]
                  n551 = call "BRig_dataCurrent_T_generic.vi"() -> ("output_T_generic"=w2020:i32)  [unwired: 11 in]
                  n552 = Index Array(array=w2016, index=w2015) -> (element=w2014:u16)
                  n553 = Replace Array Subset(array=w2018, new element #1=u16 0 ("new element/subarray"), index #1=w2021, new element #2=w2014, index #2=w2020) -> (w2017:u16[])
                }
                frame "SelectRewardPost" {
                  n554 = call "BRig_RT__Case_Exp__generic__incrementCountTilThreshold.vi"("input_dataCurrent"=w2026) -> ("output_dataCurrent"=w2024:u16[], "output_underThreshold"=w2025:bool)  [unwired: 9 in]
                  n555 = Select(t=w2028, s=w2025, f=myRIO_BRig_RT__Case_Exp_stateList."endTrial1" ("Enum")) -> (s? t:f=w2027:T2)
                }
                frame "SelectWrong_pre" {
                  # "Dual Armed\nBandit?"
                  n556 = call "BRig_dataExp_I_anySelect.vi"() -> ("output_I_anySelect"=w2038:i32)  [unwired: 11 in]
                  n557 = Index Array(array=w2039, index=w2038) -> (element=w2040:u16)
                  n558 = call "BRig_RT__Case_Exp__State_WrongOrTimeout_Pre__v11.vi"("input_dataCurrent"=w2056, "input_WorTO"=FALSE, "input_dataLC"=w2034, "input_dataBlock"=w2054, "input_dataTrial"=w2052, "input_dataExp"=w2039) -> ("output_T2R"=w2035:bool, "output_T2R_or_BTPR"=w2036:u16, "output_dataCurrent"=w2050:u16[], "output_dataBlock"=w2053:u16[][], "output_dataTrial"=w2049:u16[][], "output_BTPRavg"=w2045:dbl, "output_T2Ravg"=w2046:dbl, "output_R(F)_or_L(T)"=w2047:bool, "output_haveNewAvg"=w2048:bool)  [unwired: 1 out]
                  n559 = Not Equal To 0?(x=w2040) -> (x != 0?=w2037:bool)
                  n560 = case shown="False" w2037 {
                    tunnel: w2048 -> [_ w2072]
                    tunnel: w2047 -> [_ w2071]
                    tunnel: w2046 -> [_ w2070]
                    tunnel: w2045 -> [_ w2069]
                    tunnel: [w2061 w2067] -> w2043
                    tunnel: w2036 -> [w2059 w2063]
                    tunnel: w2035 -> [_ w2065]
                    frame True {
                      n561 = call "BRig_dataRT_stats__DAB_nTimeout.vi"() -> ("output_DAB_nTimeout"=w2058:i32)  [unwired: 11 in]
                      n562 = To Unsigned Word Integer(number=w2058) -> (unsigned 16bit integer=w2060:u16)
                      n563 = Build Array(u16 3, w2060, w2059) -> (w2061:u16[])
                    }
                    frame False {
                      n564 = case shown="False" w2065 {
                        tunnel: w2063 -> [w2074 w2076]
                        tunnel: [w2073 w2075] -> w2066
                        frame False {
                          n565 = call "BRig_dataRT_stats__BTPR_cur.vi"() -> ("output_BTPR_cur"=w2073:i32)  [unwired: 11 in]
                          n566 = local write "BTPR_block"(w2074) -> ()
                        }
                        frame True {
                          n567 = call "BRig_dataRT_stats__T2R_cur.vi"() -> ("output_T2R_cur"=w2075:i32)  [unwired: 11 in]
                          n568 = local write "T2R_block"(w2076) -> ()
                        }
                      }
                      n569 = To Unsigned Word Integer(number=w2066) -> (unsigned 16bit integer=w2064:u16)
                      n570 = case shown="True" w2072 {
                        tunnel: w2071 -> [_ w2096]
                        tunnel: w2070 -> [_ w2086]
                        tunnel: w2069 -> [_ w2082]
                        tunnel: u16 3 -> [w2080 w2089]
                        tunnel: w2064 -> [w2079 w2085]
                        tunnel: w2063 -> [w2078 w2088]
                        tunnel: [w2077 w2087] -> w2067
                        frame False {
                          n571 = Build Array(w2080, w2079, w2078) -> (w2077:u16[])
                        }
                        frame True {
                          w2081 = 100.0 ("y")
                          n572 = case shown="False" w2096 {
                            tunnel: w2086 -> [w2099 w2104]
                            tunnel: w2082 -> [w2100 w2103]
                            tunnel: [w2097 w2102] -> w2095
                            tunnel: [w2098 w2101] -> w2094
                            frame False {
                              n573 = local write "BTPR_avg_R"(w2100) -> ()
                              n574 = call "BRig_dataRT_stats__BTPR_avg_R.vi"() -> ("output_BTPR_avg_R__x100"=w2098:i32)  [unwired: 11 in]
                              n575 = local write "T2R_avg_R"(w2099) -> ()
                              n576 = call "BRig_dataRT_stats__T2R_avg_R.vi"() -> ("output_T2R_avg_R__x100"=w2097:i32)  [unwired: 11 in]
                            }
                            frame True {
                              n577 = call "BRig_dataRT_stats__BTPR_avg_L.vi"() -> ("output_BTPR_avg_L__x100"=w2101:i32)  [unwired: 11 in]
                              n578 = local write "BTPR_avg_L"(w2103) -> ()
                              n579 = local write "T2R_avg_L"(w2104) -> ()
                              n580 = call "BRig_dataRT_stats__T2R_avg_L.vi"() -> ("output_T2R_avg_L__x100"=w2102:i32)  [unwired: 11 in]
                            }
                          }
                          n581 = Multiply(x=w2086, y=w2081) -> (x*y=w2083:dbl)
                          n582 = Multiply(x=w2082, y=w2081) -> (x*y=w2084:dbl)
                          n583 = To Unsigned Word Integer(number=w2083) -> (unsigned 16bit integer=w2090:u16)
                          n584 = To Unsigned Word Integer(number=w2084) -> (unsigned 16bit integer=w2091:u16)
                          n585 = To Unsigned Word Integer(number=w2094) -> (unsigned 16bit integer=w2092:u16)
                          n586 = To Unsigned Word Integer(number=w2095) -> (unsigned 16bit integer=w2093:u16)
                          n587 = Build Array(w2089, w2093, w2090, w2089, w2092, w2091, w2089, w2085, w2088) -> (w2087:u16[])
                        }
                      }
                    }
                  }
                  n588 = RT FIFO Write(0:w2044, 1:w2043, 3:w2042) -> ()  [unwired: 2 in, 4 out]
                  n589 = call "BRig_RT_comm_tcp_write_RTwrite__RunState_Trial_selResult__v3.vi"("input_dataTrial"=w2049, "iReward_or_iError"=FALSE, "input_dataCurrent"=w2050) -> ("output_strCmd"=w2041:string)  [unwired: 8 in]
                }
                frame "SelectTimeout_pre" {
                  # "Dual Armed\nBandit?"
                  n590 = call "BRig_dataExp_I_anySelect.vi"() -> ("output_I_anySelect"=w2109:i32)  [unwired: 11 in]
                  n591 = Index Array(array=w2110, index=w2109) -> (element=w2111:u16)
                  n592 = call "BRig_RT__Case_Exp__State_WrongOrTimeout_Pre__v11.vi"("input_dataCurrent"=w2127, "input_WorTO"=TRUE, "input_dataLC"=w2105, "input_dataBlock"=w2125, "input_dataTrial"=w2123, "input_dataExp"=w2110) -> ("output_T2R"=w2106:bool, "output_T2R_or_BTPR"=w2107:u16, "output_dataCurrent"=w2121:u16[], "output_dataBlock"=w2124:u16[][], "output_dataTrial"=w2120:u16[][], "output_BTPRavg"=w2116:dbl, "output_T2Ravg"=w2117:dbl, "output_R(F)_or_L(T)"=w2118:bool, "output_haveNewAvg"=w2119:bool)  [unwired: 1 out]
                  n593 = Not Equal To 0?(x=w2111) -> (x != 0?=w2108:bool)
                  n594 = case shown="False" w2108 {
                    tunnel: w2119 -> [_ w2143]
                    tunnel: w2118 -> [_ w2142]
                    tunnel: w2117 -> [_ w2141]
                    tunnel: w2116 -> [_ w2140]
                    tunnel: [w2132 w2138] -> w2114
                    tunnel: w2107 -> [w2130 w2134]
                    tunnel: w2106 -> [_ w2136]
                    frame True {
                      n595 = call "BRig_dataRT_stats__DAB_nTimeout.vi"() -> ("output_DAB_nTimeout"=w2129:i32)  [unwired: 11 in]
                      n596 = To Unsigned Word Integer(number=w2129) -> (unsigned 16bit integer=w2131:u16)
                      n597 = Build Array(u16 3, w2131, w2130) -> (w2132:u16[])
                    }
                    frame False {
                      n598 = case shown="False" w2136 {
                        tunnel: w2134 -> [w2145 w2147]
                        tunnel: [w2144 w2146] -> w2137
                        frame False {
                          n599 = call "BRig_dataRT_stats__BTPR_cur.vi"() -> ("output_BTPR_cur"=w2144:i32)  [unwired: 11 in]
                          n600 = local write "BTPR_block"(w2145) -> ()
                        }
                        frame True {
                          n601 = call "BRig_dataRT_stats__T2R_cur.vi"() -> ("output_T2R_cur"=w2146:i32)  [unwired: 11 in]
                          n602 = local write "T2R_block"(w2147) -> ()
                        }
                      }
                      n603 = To Unsigned Word Integer(number=w2137) -> (unsigned 16bit integer=w2135:u16)
                      n604 = case shown="True" w2143 {
                        tunnel: w2142 -> [_ w2167]
                        tunnel: w2141 -> [_ w2157]
                        tunnel: w2140 -> [_ w2153]
                        tunnel: u16 3 -> [w2151 w2160]
                        tunnel: w2135 -> [w2150 w2156]
                        tunnel: w2134 -> [w2149 w2159]
                        tunnel: [w2148 w2158] -> w2138
                        frame False {
                          n605 = Build Array(w2151, w2150, w2149) -> (w2148:u16[])
                        }
                        frame True {
                          w2152 = 100.0 ("y")
                          n606 = case shown="False" w2167 {
                            tunnel: w2157 -> [w2170 w2175]
                            tunnel: w2153 -> [w2171 w2174]
                            tunnel: [w2168 w2173] -> w2166
                            tunnel: [w2169 w2172] -> w2165
                            frame False {
                              n607 = local write "BTPR_avg_R"(w2171) -> ()
                              n608 = call "BRig_dataRT_stats__BTPR_avg_R.vi"() -> ("output_BTPR_avg_R__x100"=w2169:i32)  [unwired: 11 in]
                              n609 = local write "T2R_avg_R"(w2170) -> ()
                              n610 = call "BRig_dataRT_stats__T2R_avg_R.vi"() -> ("output_T2R_avg_R__x100"=w2168:i32)  [unwired: 11 in]
                            }
                            frame True {
                              n611 = call "BRig_dataRT_stats__BTPR_avg_L.vi"() -> ("output_BTPR_avg_L__x100"=w2172:i32)  [unwired: 11 in]
                              n612 = local write "BTPR_avg_L"(w2174) -> ()
                              n613 = local write "T2R_avg_L"(w2175) -> ()
                              n614 = call "BRig_dataRT_stats__T2R_avg_L.vi"() -> ("output_T2R_avg_L__x100"=w2173:i32)  [unwired: 11 in]
                            }
                          }
                          n615 = Multiply(x=w2157, y=w2152) -> (x*y=w2154:dbl)
                          n616 = Multiply(x=w2153, y=w2152) -> (x*y=w2155:dbl)
                          n617 = To Unsigned Word Integer(number=w2154) -> (unsigned 16bit integer=w2161:u16)
                          n618 = To Unsigned Word Integer(number=w2155) -> (unsigned 16bit integer=w2162:u16)
                          n619 = To Unsigned Word Integer(number=w2165) -> (unsigned 16bit integer=w2163:u16)
                          n620 = To Unsigned Word Integer(number=w2166) -> (unsigned 16bit integer=w2164:u16)
                          n621 = Build Array(w2160, w2164, w2161, w2160, w2163, w2162, w2160, w2156, w2159) -> (w2158:u16[])
                        }
                      }
                    }
                  }
                  n622 = RT FIFO Write(0:w2115, 1:w2114, 3:w2113) -> ()  [unwired: 2 in, 4 out]
                  n623 = call "BRig_RT_comm_tcp_write_RTwrite__RunState_Trial_selResult__v3.vi"("input_dataTrial"=w2120, "iReward_or_iError"=FALSE, "input_dataCurrent"=w2121) -> ("output_strCmd"=w2112:string)  [unwired: 8 in]
                }
                frame "SelectWrong" {
                  n624 = call "BRig_RT__Case_Exp__generic__incrementCountTilThreshold.vi"("input_dataCurrent"=w2178) -> ("output_dataCurrent"=w2176:u16[], "output_underThreshold"=w2177:bool)  [unwired: 9 in]
                  n625 = Select(t=w2180, s=w2177, f=myRIO_BRig_RT__Case_Exp_stateList."endTrial1" ("Enum")) -> (s? t:f=w2179:T2)
                }
                frame "SelectTimeout" {
                  n626 = call "BRig_RT__Case_Exp__generic__incrementCountTilThreshold.vi"("input_dataCurrent"=w2188) -> ("output_dataCurrent"=w2187:u16[], "output_underThreshold"=w2186:bool)  [unwired: 9 in]
                  n627 = Select(t=w2190, s=w2186, f=myRIO_BRig_RT__Case_Exp_stateList."endTrial1" ("Enum")) -> (s? t:f=w2189:T2)
                }
                frame "endTrial1" {
                  n628 = call "BRig_RT_comm_tcp_write_RTwrite__RunState_Trial_end.vi"("input_dataCurrent"=w2204) -> ("output_strCmd"=w2203:string)  [unwired: 10 in]
                  n629 = call "BRig_RT__Case_Exp__State_endTrial__v10.vi"("input_dataBlock"=w2200, "input_timeStamp_start"=w2205, "input_dataTrial"=w2212, "input_dataCurrent"=w2204) -> ("output_BTPRavg"=w2197:dbl, "output_T2Ravg"=w2198:dbl, "output_dataTrial"=w2211:u16[][], "output_dataCurrent"=w2206:u16[], "output_R(F)_or_L(T)"=w2199:bool, "output_runTime"=→"T_ExpRun_min":dbl)  [unwired: 2 in]
                  n630 = xnode "Read/Write Control"("FPGA VI Reference In"=w2208, "error in"=w2207, "SelectionState"=FALSE) -> ("error out"=w2209:errorcluster)  [unwired: 1 out]
                  n631 = case shown="False" w2199 {
                    tunnel: w2198 -> [w2214 w2217]
                    tunnel: w2197 -> [w2215 w2216]
                    frame False {
                      n632 = local write "BTPR_avg_R"(w2215) -> ()
                      n633 = local write "T2R_avg_R"(w2214) -> ()
                    }
                    frame True {
                      n634 = local write "BTPR_avg_L"(w2216) -> ()
                      n635 = local write "T2R_avg_L"(w2217) -> ()
                    }
                  }
                  n636 = local write "error out"(w2209) -> ()
                }
                frame "endTrial2" {
                  n637 = case shown="True" w2227 {
                    tunnel: [w2235 _] -> w2228
                    tunnel: [w2234 w2237] -> w2223
                    tunnel: w2222 -> [w2232 w2245]
                    tunnel: w2221 -> [w2233 w2243]
                    tunnel: [w2233 w2242] -> w2220
                    tunnel: [w2232 w2244] -> w2219
                    tunnel: w2218 -> [_ w2236]
                    frame False {
                      # "Receive commands"
                      n638 = call "BRig_RT__Case_Exp__UploadClosedLoop__v3.vi"() -> ("all rows"=w2235:i64[][], "output_haveCmd"=w2234:bool)  [unwired: 10 in]
                    }
                    frame True {
                      # "Parse commands and update"
                      n639 = Array Size(array=w2236) -> (size(s)=w2241:i32[])
                      n640 = Index Array(array=w2241, index=0) -> (element=w2239:i32)
                      n641 = Not Equal To 0?(x=w2239) -> (x != 0?=w2238:bool)
                      n642 = case shown="False" w2238 {
                        selector: w2238 -> [w2249 w2251]
                        tunnel: w2245 -> [w2247 w2255]
                        tunnel: [w2247 w2254] -> w2244
                        tunnel: w2243 -> [w2246 w2253]
                        tunnel: [w2246 w2252] -> w2242
                        tunnel: [w2249 w2251] -> w2237
                        tunnel: w2236 -> [_ w2250]
                        frame False {
                          w2248 = TRUE ("input_setValues")
                          # "Update"
                          n643 = call "BRig_RT_panel_cue_v1,18.vi"("input_setValues"=w2248, "input_dataExp"=w2247) -> ()  [unwired: 9 in, 1 out]
                          n644 = call "BRig_RT_panel_ExpStruct_v1,18.vi"("input_setValues"=w2248, "input_dataExp"=w2247) -> ()  [unwired: 9 in, 1 out]
                          n645 = call "BRig_RT_panel_Laser1_v1,18.vi"("input_setValues"=w2248, "input_dataExp"=w2247, "input_dataLC"=w2246) -> ()  [unwired: 7 in, 2 out]
                          n646 = call "BRig_RT_panel_Laser2_v1,13.vi"("input_setValues"=w2248, "input_dataExp"=w2247, "input_dataLC"=w2246) -> ()  [unwired: 7 in, 2 out]
                        }
                        frame True {
                          # "Parse"
                          n647 = call "BRig_RT__Case_Exp__UploadClosedLoop__updateSettings.vi"("input_newSettings"=w2250, "input_dataLC"=w2253, "input_dataExp"=w2255) -> ("output_dataLC"=w2252:u16[], "output_dataExp"=w2254:u16[])  [unwired: 7 in]
                        }
                      }
                    }
                  }
                  n648 = Select(t=myRIO_BRig_RT__Case_Exp_stateList."endTrial2", s=w2223, f=myRIO_BRig_RT__Case_Exp_stateList."endTrial3" ("Enum")) -> (s? t:f=w2224:T2)
                }
                frame "endTrial3" {
                  # "Two cues?"
                  # "Dual Armed Bandit?"
                  n649 = call "BRig_dataExp_I_anySelect.vi"() -> ("output_I_anySelect"=w2263:i32)  [unwired: 11 in]
                  n650 = call "BRig_dataExp_I_Cue2.vi"() -> ("output_I_Cue2"=w2261:i32)  [unwired: 11 in]
                  n651 = call "BRig_RT__Case_Exp__endTrial_checkFreeReward__v17.vi"("input_dataBlock"=w2266, "input_dataExp"=w2257, "input_dataTrial"=w2275, "input_dataCurrent"=w2276) -> ("output_state"=w2267:T2, "output_endBlock"=w2265:bool)  [unwired: 6 in]
                  n652 = Index Array(array=w2257, index #1=w2263, index #2=w2261) -> (element #1=w2262:u16, element #2=w2260:u16)  [unwired: 1 in, 1 out]
                  n653 = Not Equal To 0?(x=w2262) -> (x != 0?=w2259:bool)
                  n654 = Not Equal To 0?(x=w2260) -> (x != 0?=w2258:bool)
                  n655 = local read "STOP_endTrial"() -> (w2274:bool)
                  n656 = Or(x=w2259, y=w2258) -> (x .or. y?=w2256:bool)
                  n657 = local read "STOP_abort"() -> (w2273:bool)
                  n658 = case shown="True" w2256 {
                    tunnel: w2257 -> [w2278 w2279]
                    tunnel: [w2278 w2280] -> w2264
                    frame False {
                    }
                    frame True {
                      # "Get latest\nlaserSwitch"
                      n659 = call "BRig_dataExp_Loop_c_ExpStruct.vi"() -> ("output_Loop_c_ExpStruct"=w2286:i32)  [unwired: 11 in]
                      n660 = call "BRig_dataExp_LaserSwitch.vi"() -> ("output_LaserSwitch"=w2282:i32)  [unwired: 11 in]
                      n661 = Replace Array Subset(array=w2279, new element=u16 2 ("new element/subarray"), index=w2286) -> (w2284:u16[])
                      n662 = call "BRig_RT_panel_ExpStruct_v1,14.vi"("input_setValues"=FALSE, "input_dataExp"=w2284) -> ("output_dataExp"=w2283:u16[])  [unwired: 9 in]
                      n663 = Index Array(array=w2283, index=w2282) -> (element=w2281:u16)
                      n664 = Replace Array Subset(array=w2279, new element=w2281, index=w2282) -> (w2280:u16[])
                    }
                  }
                  n665 = local read "START"() -> (w2271:bool)
                  n666 = Not(x=w2271) -> (.not. x?=w2272:bool)
                  n667 = Compound Arithmetic op=OR(w2274, w2272, w2273, w2265) -> (w2270:bool)
                  n668 = Select(t=myRIO_BRig_RT__Case_Exp_stateList."saveData_dataBlock" ("Enum"), s=w2270, f=w2267) -> (s? t:f=w2268:T2)
                }
                frame "endBlock" {
                  # "Get latest\nlaserSwitch"
                  n669 = call "BRig_dataExp_Loop_c_ExpStruct.vi"() -> ("output_Loop_c_ExpStruct"=w2295:i32)  [unwired: 11 in]
                  n670 = call "BRig_dataExp_LaserSwitch.vi"() -> ("output_LaserSwitch"=w2290:i32)  [unwired: 11 in]
                  n671 = local read "START"() -> (w2314:bool)
                  n672 = local read "STOP_endBlock"() -> (w2310:bool)
                  n673 = local read "STOP_endTrial"() -> (w2312:bool)
                  n674 = local read "STOP_abort"() -> (w2311:bool)
                  n675 = Replace Array Subset(array=w2288, new element=u16 2 ("new element/subarray"), index=w2295) -> (w2293:u16[])
                  n676 = call "BRig_RT_panel_ExpStruct_v1,18.vi"("input_setValues"=FALSE, "input_dataExp"=w2293) -> ("output_dataExp"=w2292:u16[])  [unwired: 9 in]
                  n677 = Index Array(array=w2292, index=w2290) -> (element=w2289:u16)
                  n678 = Not(x=w2314) -> (.not. x?=w2313:bool)
                  n679 = Select(t=myRIO_BRig_RT__Case_Exp_stateList."commUpload_dataTrial" ("Enum"), s=w2300, f=myRIO_BRig_RT__Case_Exp_stateList."initBlock" ("Enum")) -> (s? t:f=w2297:T2)
                  n680 = Replace Array Subset(array=w2288, new element=w2289, index=w2290) -> (w2291:u16[])
                  n681 = Compound Arithmetic op=OR(w2313, w2310, w2312, w2311) -> (w2304:bool)
                  n682 = Select(t=myRIO_BRig_RT__Case_Exp_stateList."endExp" ("Enum"), s=w2304, f=w2297) -> (s? t:f=w2315:T2)
                  n683 = Select(t="<S,E>" ("string"), s=w2304, f="") -> (s? t:f=w2301:string)
                }
                frame "endExp" {
                  n684 = xnode "Read/Write Control"("FPGA VI Reference In"=w2319, "error in"=w2318, "A6_Act"=FALSE) -> ("error out"=w2320:errorcluster)  [unwired: 1 out]
                  n685 = local write "error out"(w2320) -> ()
                }
                frame "commUpload_dataTrial" {
                }
                frame "saveData_dataBlock" {
                  n686 = Increment(x=w2349) -> (x+1=w2347:u16)
                  n687 = Replace Array Subset(array=w2341, new element=u16 2 ("new element/subarray"), index=0) -> (w2335:u16[])
                  n688 = Index Array(array=w2333, index (row)=0) -> (element=w2336:u16[])  [unwired: 1 in]
                  n689 = for {
                    tunnel: w2336 -> [w2359] mode=indexing
                    shift-right: [w2358] -> w2334
                    shift-left: w2335 -> [w2362]
                    i -> [w2361]
                    n690 = Increment(x=w2361) -> (x+1=w2360:i32)
                    n691 = Replace Array Subset(array=w2362, new element=w2359, index=w2360) -> (w2358:u16[])
                  }
                  n692 = RT FIFO Write(0:w2344, 1:w2334, 3:w2343) -> (11:w2346:errorcluster)  [unwired: 2 in, 3 out]
                  n693 = Unbundle By Name(w2346) -> ("code"=w2345:i32)
                  n694 = Greater?(x=w2347, y=u16 3) -> (0:w2355:bool)
                  n695 = Equal To 0?(x=w2345) -> (x = 0?=w2342:bool)
                  n696 = Or(x=w2355, y=w2342) -> (x .or. y?=w2354:bool)
                  n697 = Select(t=myRIO_BRig_RT__Case_Exp_stateList."endBlock" ("Enum"), s=w2354, f=w2350) -> (s? t:f=w2348:T2)
                }
                frame "saveData_dataTrial" {
                  n698 = Increment(x=w2380) -> (x+1=w2379:u16)
                  n699 = Replace Array Subset(array=w2365, new element=u16 1 ("new element/subarray"), index=0) -> (w2369:u16[])
                  n700 = Index Array(array=w2364, index (row)=0) -> (element=w2370:u16[])  [unwired: 1 in]
                  n701 = for {
                    tunnel: w2370 -> [w2389] mode=indexing
                    shift-right: [w2388] -> w2368
                    shift-left: w2369 -> [w2392]
                    i -> [w2391]
                    n702 = Increment(x=w2391) -> (x+1=w2390:i32)
                    n703 = Replace Array Subset(array=w2392, new element=w2389, index=w2390) -> (w2388:u16[])
                  }
                  n704 = RT FIFO Write(0:w2367, 1:w2368, 3:w2366) -> (11:w2375:errorcluster)  [unwired: 2 in, 3 out]
                  n705 = Unbundle By Name(w2375) -> ("code"=w2374:i32)
                  n706 = Equal To 0?(x=w2374) -> (x = 0?=w2363:bool)
                  n707 = Greater?(x=w2379, y=u16 3) -> (0:w2377:bool)
                  n708 = Or(x=w2377, y=w2363) -> (x .or. y?=w2376:bool)
                  n709 = Select(t=myRIO_BRig_RT__Case_Exp_stateList."endTrial2" ("Enum"), s=w2376, f=w2381) -> (s? t:f=w2382:T2)
                }
                frame "dummyState" {
                  n710 = call "BRig_dataCurrent_iTrial.vi"() -> ("output_iTrial"=w2399:i32)  [unwired: 11 in]
                  n711 = Index Array(array=w2400, index=w2399) -> (element=w2398:u16)
                  n712 = Equal?(x=w2398, y=u16 1) -> (x = y?=w2396:bool)
                  n713 = Equal To 0?(x=w2407) -> (x = 0?=w2408:bool)
                  n714 = Select(t=u16 13, s=w2396, f=u16 15) -> (s? t:f=w2393:u16)
                  n715 = Select(t=w2393, s=w2408, f=w2407) -> (s? t:f=w2406:u16)
                  n716 = Decrement(x=w2406) -> (x-1=w2405:u16)
                  n717 = Equal To 0?(x=w2405) -> (x = 0?=w2404:bool)
                  n718 = Select(t=myRIO_BRig_RT__Case_Exp_stateList."initTrial" ("Enum"), s=w2404, f=w2402) -> (s? t:f=w2401:T2)
                }
                frame "dummyState_endBlock" {
                  n719 = call "BRig_dataCurrent_iTrial.vi"() -> ("output_iTrial"=w2423:i32)  [unwired: 11 in]
                  n720 = Index Array(array=w2417, index=w2423) -> (element=w2413:u16)
                  n721 = Equal?(x=w2413, y=u16 1) -> (x = y?=w2421:bool)
                  n722 = Equal To 0?(x=w2414) -> (x = 0?=w2425:bool)
                  n723 = Select(t=u16 1, s=w2421, f=u16 3) -> (s? t:f=w2418:u16)
                  n724 = Select(t=w2418, s=w2425, f=w2414) -> (s? t:f=w2424:u16)
                  n725 = Decrement(x=w2424) -> (x-1=w2415:u16)
                  n726 = Equal To 0?(x=w2415) -> (x = 0?=w2416:bool)
                  n727 = Select(t=myRIO_BRig_RT__Case_Exp_stateList."initBlock" ("Enum"), s=w2416, f=w2427) -> (s? t:f=w2426:T2)
                }
                frame "FreeReward_pre" {
                  w2463 = u16 0 ("new element/subarray")
                  # "Duration = MTrig duration"
                  # "Duration = Reward Time"
                  n728 = call "BRig_dataCurrent_FreeReward_c.vi"() -> ("output_FreeReward_c"=w2464:i32)  [unwired: 11 in]
                  n729 = call "BRig_dataCurrent_iSpout.vi"() -> ("output_iSpout"=w2461:i32)  [unwired: 11 in]
                  n730 = call "BRig_dataCurrent_c_generic.vi"() -> ("output_count_generic"=w2470:i32)  [unwired: 11 in]
                  n731 = call "BRig_dataCurrent_T_generic.vi"() -> ("output_T_generic"=w2469:i32)  [unwired: 11 in]
                  n732 = Index Array(array=w2462, index=w2461) -> (element=w2460:u16)
                  n733 = call "BRig_dataMTrig_Solenoid_T_L.vi"() -> ("output_Solenoid_T_L"=w2459:i32)  [unwired: 11 in]
                  n734 = call "BRig_dataMTrig_Solenoid_T_R.vi"() -> ("output_Solenoid_T_R"=w2458:i32)  [unwired: 11 in]
                  n735 = local read "FPGA_count2ms"() -> (w2440:dbl)
                  n736 = call "BRig_dataTrial_T_Reward.vi"() -> ("output_T_Reward"=w2465:i32)  [unwired: 11 in]
                  n737 = Equal To 0?(x=w2460) -> (x = 0?=w2442:bool)
                  n738 = Select(t=w2459, s=w2442, f=w2458) -> (s? t:f=w2456:i32)
                  n739 = Index Array(array=w2466, index (row)=0 ("disabled index (row)"), index (col)=w2465) -> ()  [unwired: 1 out]
                  n740 = Index Array(array=w2457, index=w2456) -> (element=w2453:u16)
                  n741 = Replace Array Subset(array=w2462, new element #1=w2463, index #1=w2464, new element #2=w2463, index #2=w2470, new element #3=w2453, index #3=w2469) -> (w2468:u16[])
                  n742 = To Double Precision Float(number=w2453) -> (double precision float=w2441:dbl)
                  n743 = Multiply(x=w2441, y=w2440) -> (x*y=w2454:dbl)
                  n744 = call "BRig_dataExp_FreeReward_c_L.vi"() -> ("output_FreeReward_c_L"=w2447:i32)  [unwired: 11 in]
                  n745 = call "BRig_dataExp_FreeReward_c_R.vi"() -> ("output_FreeReward_c_R"=w2448:i32)  [unwired: 11 in]
                  n746 = Round Toward +Infinity(x=w2454) -> (ceil(x): smallest int >= x=w2455:dbl)
                  n747 = Select(t=w2447, s=w2442, f=w2448) -> (s? t:f=w2444:i32)
                  n748 = To Unsigned Long Integer(number=w2455) -> (unsigned 32bit integer=w2450:u32)
                  n749 = xnode "Read/Write Control"("FPGA VI Reference In"=w2452, "error in"=w2451, "Solenoid_nTotal_L"=w2450, "Solenoid_nTotal_R"=w2450) -> ()  [unwired: 2 out]
                  n750 = Index Array(array=w2445, index=w2444) -> (element=w2443:u16)
                  n751 = Increment(x=w2443) -> (x+1=w2433:u16)
                  n752 = case shown="True" w2442 {
                    tunnel: w2433 -> [w2474 w2476]
                    tunnel: [w2473 w2475] -> w2435
                    frame True {
                      n753 = local write "FreeReward_c_L"(w2474) -> ()
                      n754 = call "BRig_dataRT_stats__FreeReward_c_L.vi"() -> ("output_FreeReward_c_L"=w2473:i32)  [unwired: 11 in]
                    }
                    frame False {
                      n755 = local write "FreeReward_c_R"(w2476) -> ()
                      n756 = call "BRig_dataRT_stats__FreeReward_c_R.vi"() -> ("output_FreeReward_c_R"=w2475:i32)  [unwired: 11 in]
                    }
                  }
                  n757 = To Unsigned Word Integer(number=w2435) -> (unsigned 16bit integer=w2434:u16)
                  n758 = Build Array(u16 3, w2434, w2433) -> (w2439:u16[])
                  n759 = Replace Array Subset(array=w2445, new element=w2433, index=w2444) -> (w2446:u16[])
                  n760 = RT FIFO Write(0:w2437, 1:w2439, 3:w2436) -> ()  [unwired: 2 in, 4 out]
                }
                frame "FreeReward" {
                  n761 = call "BRig_dataCurrent_iSpout.vi"() -> ("output_iSpout"=w2487:i32)  [unwired: 11 in]
                  n762 = call "BRig_dataCurrent_c_generic.vi"() -> ("output_count_generic"=w2481:i32)  [unwired: 11 in]
                  n763 = Index Array(array=w2488, index #1=w2487, index #2=w2481) -> (element #1=w2486:u16, element #2=w2480:u16)
                  n764 = Equal To 0?(x=w2486) -> (x = 0?=w2484:bool)
                  n765 = Equal To 0?(x=w2480) -> (x = 0?=w2479:bool)
                  n766 = Not(x=w2484) -> (.not. x?=w2485:bool)
                  n767 = call "BRig_RT__Case_Exp__generic__incrementCountTilThreshold.vi"("input_dataCurrent"=w2488) -> ("output_dataCurrent"=w2489:u16[], "output_underThreshold"=w2478:bool)  [unwired: 9 in]
                  n768 = Select(t=w2492, s=w2478, f=myRIO_BRig_RT__Case_Exp_stateList."FreeRewardPost_pre" ("Enum")) -> (s? t:f=w2490:T2)
                  n769 = And(x=w2478, y=w2479) -> (x .and. y?=w2477:bool)
                  n770 = And(x=w2477, y=w2484) -> (x .and. y?=w2482:bool)
                  n771 = And(x=w2477, y=w2485) -> (x .and. y?=w2483:bool)
                }
                frame "FreeRewardPost" {
                  n772 = call "BRig_RT__Case_Exp__generic__incrementCountTilThreshold.vi"("input_dataCurrent"=w2499) -> ("output_dataCurrent"=w2498:u16[], "output_underThreshold"=w2497:bool)  [unwired: 9 in]
                  n773 = Select(t=w2502, s=w2497, f=myRIO_BRig_RT__Case_Exp_stateList."initTrial" ("Enum")) -> (s? t:f=w2500:T2)
                }
                frame "FreeRewardPost_pre" {
                  n774 = call "BRig_dataExp_T_RewardPost.vi"() -> ("output_T_RewardPost"=w2512:i32)  [unwired: 11 in]
                  n775 = call "BRig_dataCurrent_c_generic.vi"() -> ("output_count_generic"=w2515:i32)  [unwired: 11 in]
                  n776 = call "BRig_dataCurrent_T_generic.vi"() -> ("output_T_generic"=w2514:i32)  [unwired: 11 in]
                  n777 = Index Array(array=w2509, index=w2512) -> (element=w2511:u16)
                  n778 = Replace Array Subset(array=w2510, new element #1=u16 0 ("new element/subarray"), index #1=w2515, new element #2=w2511, index #2=w2514) -> (w2508:u16[])
                }
              }
              n779 = call "BRig_RT_panel_manualTriggering_v0,90.vi"("input_dataMTrig"=w1312) -> ("output_Solenoid_R"=w1323:bool, "output_Solenoid_L"=w1322:bool, "output_dataMTrig"=w1355:u16[], "output_Audio_L"=w1354:bool, "output_Audio_R"=w1353:bool, "output_CueLed"=w1351:bool, "output_Laser_l1"=w1327:bool, "output_Laser_l2"=w1347:bool)  [unwired: 11 in]
              n780 = call "BRig_RT__Case_Exp__comm_tcp__data_other.vi"("input_strState"=w1315, "input_strAccum"=w1316, "input_error"=w1317, "input_hTCP"=w1318, "input_I_connected_TCP"=w1319) -> ("output_strAccum"=w1298:string, "output_error"=w1297:errorcluster, "output_hTCP"=w1299:refnum<k5>, "output_I_connect_TCP"=w1300:bool)  [unwired: 3 in]
              n781 = Or(x="STOP_abort", y=w1339) -> (x .or. y?=w1301:bool)
              n782 = Or(x=w1352, y=w1351) -> (x .or. y?=w1330:bool)
              n783 = local read "Laser1_LED"() -> (w1288:bool)
              n784 = local read "Laser2_LED"() -> (w1287:bool)
              n785 = Or(x=w1354, y=w1369) -> (x .or. y?=w1329:bool)
              n786 = Or(x=w1368, y=w1353) -> (x .or. y?=w1328:bool)
              n787 = Or(x=w1326, y=w1327) -> (x .or. y?=w1346:bool)
              n788 = Or(x=w1350, y=w1347) -> (x .or. y?=w1348:bool)
              n789 = call "BRig_RT__Case_Exp__recordLick.vi"("input_dataLick"=w1338, "input_lick__R"=w1332, "input_lick__L"=w1333, "input_lick"=w1334, "intput_state__trialStart"=w1292, "intput_state__trialEnd"=w1337, "input_dataCurrent"=w1336) -> ("output_dataLick"=w1331:u16[][], "output_dataCurrent"=w1335:u16[])  [unwired: 7 in]
              n790 = xnode "Read/Write Control"("FPGA VI Reference In"=w1367, "error in"=w1366, "L1Led_ON"=w1288, "L2Led_ON"=w1287, "Solenoid_trig_L"=w1321, "Solenoid_trig_R"=w1320, "A3_SL"=w1322, "A1_SR"=w1323, "LC_Event_l1"=w1345, "LC_Laser_l1"=w1346, "LC_Event_l2"=w1349, "LC_Laser_l2"=w1348, "CueLed_Event"=w1330, "audioTrigger_L"=w1329, "audioTrigger_R"=w1328) -> ("FPGA VI Reference Out"=w1373:refnum<k20>, "error out"=w1372:errorcluster, "fpga_laser1"=w1286:bool, "fpga_laser2"=w1285:bool, "fpga_solenoid_L"=w1284:bool, "fpga_solenoid_R"=w1283:bool, "AnaIn_0"=w1313:i16, "AnaIn_1"=w1314:i16)
              n791 = local write "Laser1"(w1286) -> ()
              n792 = local write "Laser2"(w1285) -> ()
              n793 = local write "Solenoid L"(w1284) -> ()
              n794 = local write "Solenoid R"(w1283) -> ()
              n795 = call "BRig_RT__Case_Exp__recordAnalogInput__PortC__fifo__1value.vi"("input_iOccurence"=w1343, "resetOccurrence"=w1342, "input_dataCurrent"=w1336, "input_iState_start"=w1292, "rt fifo"=w1291, "input_iState_end"=w1337, "input_fifo_error"=w1290, "input_AI1"=w1314, "input_AI0"=w1313) -> ("output_fifo_error"=w1296:errorcluster, "output_iOccurrence"=w1344:u16)  [unwired: 8 in, 1 out]
              n796 = call "BRig_RT_timeLoop_Exp__noStateLimit.vi"("input_error"=w1296, "input_Threshold_reset"="input_Threshold_reset", "input_Threshold"=w1358, "input_timestamp"=w1359, "input_state"=w1292) -> ("output_Threshold"=w1356:bool, "output_duration"=→"tLoop":dbl)  [unwired: 4 in, 1 out]
              "Threshold" <- w1356
              n797 = node-c288() -> ()  [unwired: 1 in, 1 out]
            }
            "stop_TimedLoop" <- w897
            n798 = while {
              tunnel: w841 -> [w965]
              tunnel: w840 -> [w964]
              shift-right: [w959] -> _
              shift-left: 0 ("element") -> [w960]
              shift-right: [w955] -> _
              shift-left: w846 -> [w961]
              tunnel: [w958] -> w843
              tunnel: [w957] -> w842
              tunnel: w839 -> [w954]
              tunnel: w838 -> [w953]
              tunnel: [w952] -> w837
              tunnel: [w951] -> w836
              shift-right: [w949] -> _
              shift-left: FALSE -> [w950]
              stop <- w948 stop-if-true
              # "If buffer is full, send to Host"
              # "Collect analog input data in groups of 8"
              # "Receive latest analog input"
              # "This non-timed loop receives AnalogInput\ndata and passes it to the Host"
              # "timed out?"
              n799 = RT FIFO Read(0:w965, 3:w964) -> (8:w958:refnum<k33>, 9:w962:u16, 10:w969:bool, 11:w966:errorcluster)  [unwired: 2 in, 1 out]
              n800 = Unbundle By Name(w966) -> ("code"=w970:i32)
              n801 = Not(x=w969) -> (.not. x?=w968:bool)
              n802 = Equal To 0?(x=w970) -> (x = 0?=w967:bool)
              n803 = And(x=w967, y=w968) -> (x .and. y?=w963:bool)
              n804 = Select(t=w966, s=w967, f=w964) -> (s? t:f=w957:errorcluster)
              n805 = case shown="True" w963 {
                tunnel: w962 -> [_ w1001]
                tunnel: w961 -> [w993 w1003]
                tunnel: w960 -> [w992 w1000]
                tunnel: [w993 w1002] -> w955
                tunnel: [w992 w996] -> w959
                tunnel: [_ w994] -> w956
                frame False {
                }
                frame True {
                  n806 = Replace Array Subset(array=w1003, new element=w1001, index=w1000) -> (w1002:u16[])
                  n807 = Increment(x=w1000) -> (x+1=w998:i32)
                  n808 = Less?(x=w1000, y=7 ("dimension size")) -> (x < y?=w995:bool)
                  n809 = Select(t=w998, s=w995, f=0) -> (s? t:f=w996:i32)
                  n810 = Not(x=w995) -> (.not. x?=w994:bool)
                }
              }
              n811 = case shown="True" w956 {
                tunnel: w955 -> [_ w982]
                tunnel: w954 -> [w973 w981]
                tunnel: w953 -> [w972 w980]
                tunnel: [w973 w978] -> w952
                tunnel: [w972 w977] -> w951
                tunnel: w950 -> [w971 w975]
                tunnel: [w971 w974] -> w949
                frame False {
                }
                frame True {
                  n812 = for {
                    N: 8 -> [_]
                    tunnel: w982 -> [w989] mode=indexing
                    tunnel: w981 -> [w991]
                    tunnel: w980 -> [w990]
                    shift-right: [w984] -> w976
                    shift-left: FALSE -> [w988]
                    tunnel: [w987] -> w978
                    tunnel: [w986] -> w977
                    n813 = shared-variable-write(w991, w990, w989) -> (w987:refnum<k21>, w986:errorcluster, w985:bool)  [unwired: 1 in]
                    n814 = Or(x=w988, y=w985) -> (x .or. y?=w984:bool)
                  }
                  n815 = Or(x=w975, y=w976) -> (x .or. y?=w974:bool)
                }
              }
              n816 = local read "stop_TimedLoop"() -> (w948:bool)
            }
            n817 = while {
              shift-right: [w1074] -> _
              shift-left: 0 -> [w1063]
              tunnel: w894 -> [w1081]
              tunnel: w886 -> [w1083]
              shift-right: [w1070] -> _
              shift-left: 0 -> [w1065]
              shift-right: [w1075] -> _
              shift-left: w833 -> [w1082]
              shift-right: [w1071] -> _
              shift-left: w861 -> [w1084]
              shift-right: [w1078] -> w883
              shift-left: w855 -> [w1091]
              shift-right: [w1079] -> w877
              shift-left: w854 -> [w1085]
              tunnel: w858 -> [w1068]
              tunnel: w862 -> [w1067]
              shift-right: [w1056] -> _
              shift-left: w828 -> [w1062]
              shift-right: [w1055] -> _
              shift-left: 0 -> [w1061]
              tunnel: w831 -> [w1059]
              tunnel: w830 -> [w1060]
              tunnel: [w1054] -> w825
              tunnel: [w1053] -> w824
              stop <- w1092 stop-if-true
              # "This non-timed loop received Trial/Block status information\nand passes it on the Host. This includes stats such as\nnumber of total rewards or target trials per block"
              # "nColumns dataBlock"
              # "nColumns dataTrial"
              # "buffer_dataTrial"
              # "buffer_dataBlock"
              # "buffer_dataTrial"
              # "buffer_dataBlock"
              n818 = local read "stop_TimedLoop"() -> (w1092:bool)
              n819 = Not Equal To 0?(x=w1065) -> (x != 0?=w1066:bool)
              n820 = Not Equal To 0?(x=w1061) -> (x != 0?=w1052:bool)
              n821 = case shown="True" w1066 {
                tunnel: w1084 -> [w1244 w1247]
                tunnel: w1065 -> [w1245 w1249]
                tunnel: w1083 -> [_ w1258]
                tunnel: [w1245 w1246] -> w1072
                tunnel: [w1244 w1247] -> w1073
                frame False {
                }
                frame True {
                  n822 = Array Subset(array=w1247, length (row)=w1249) -> (w1260:u16[][])  [unwired: 3 in]
                  n823 = call "BRig_dataBlock_iBlock.vi"() -> ("output_iBlock"=w1255:i32)  [unwired: 11 in]
                  n824 = Index Array(array=w1247, index (row)=0, index (col)=w1255) -> (element=w1254:u16)
                  n825 = To Double Precision Float(number=w1260) -> (double precision float=w1259:dbl[][])
                  n826 = Not Equal?(x=u16 1, y=w1254) -> (x != y?=w1252:bool)
                  n827 = call-poly <vilib>:"Write To Spreadsheet File.vi"("delimiter (\\t)"="," ("delimiter (\\t)"), "append to file? (new file:F)"=w1252, "2D data"=w1259, "file path (dialog if empty)"=w1258) -> ("new file path (Not A Path if cancelled)"=w1251:path)  [unwired: 4 in]
                  n828 = call <vilib>:"Is Path and Not Empty.vi"("path"=w1251) -> ("Is Path and Not Empty?"=w1250:bool)  [unwired: 4 in]
                  n829 = Select(t=0, s=w1250, f=w1249) -> (s? t:f=w1246:i32)
                }
              }
              n830 = case shown="True" w1052 {
                tunnel: w1062 -> [w1096 w1105]
                tunnel: w1061 -> [w1095 w1098]
                tunnel: [w1095 w1104] -> w1057
                tunnel: [w1096 w1105] -> w1058
                tunnel: w1060 -> [w1094 w1113]
                tunnel: w1059 -> [w1093 w1112]
                tunnel: [w1094 w1103] -> w1054
                tunnel: [w1093 w1102] -> w1053
                frame False {
                }
                frame True {
                  n831 = Decrement(x=w1098) -> (x-1=w1097:i32)
                  n832 = Multiply(x=w1097, y=2 ("index")) -> (x*y=w1099:i32)
                  n833 = Increment(x=w1099) -> (x+1=w1100:i32)
                  n834 = Index Array(array=w1105, index #1=w1099, index #2=w1100) -> (element #1=w1111:u16, element #2=w1107:u16)
                  n835 = shared-variable-write(w1113, w1112, w1111) -> (w1108:refnum<k21>, w1109:errorcluster, w1110:bool)  [unwired: 1 in]
                  n836 = case shown="False" w1110 {
                    selector: w1110 -> [_ w1122]
                    tunnel: w1109 -> [w1119 w1120]
                    tunnel: w1108 -> [w1118 w1121]
                    tunnel: w1107 -> [w1117 _]
                    tunnel: [w1116 w1122] -> w1106
                    tunnel: [w1115 w1121] -> w1103
                    tunnel: [w1114 w1120] -> w1102
                    frame False {
                      n837 = shared-variable-write(w1118, w1119, w1117) -> (w1115:refnum<k21>, w1114:errorcluster, w1116:bool)  [unwired: 1 in]
                    }
                    frame True {
                    }
                  }
                  n838 = Select(t=w1098, s=w1106, f=w1097) -> (s? t:f=w1104:i32)
                }
              }
              n839 = RT FIFO Read(0:w1091, 3:w1085) -> (8:w1078:refnum<k33>, 9:w1069:u16[], 10:w1089:bool, 11:w1086:errorcluster)  [unwired: 2 in, 1 out]
              n840 = Unbundle By Name(w1086) -> ("code"=w1090:i32)
              n841 = Not(x=w1089) -> (.not. x?=w1088:bool)
              n842 = Equal To 0?(x=w1090) -> (x = 0?=w1087:bool)
              n843 = And(x=w1087, y=w1088) -> (x .and. y?=w1080:bool)
              n844 = Select(t=w1086, s=w1087, f=w1085) -> (s? t:f=w1079:errorcluster)
              n845 = Not Equal To 0?(x=w1063) -> (x != 0?=w1064:bool)
              n846 = case shown="True" w1064 {
                tunnel: w1082 -> [w1227 w1230]
                tunnel: w1063 -> [w1228 w1232]
                tunnel: w1081 -> [_ w1241]
                tunnel: [w1228 w1229] -> w1076
                tunnel: [w1227 w1230] -> w1077
                frame False {
                }
                frame True {
                  n847 = Array Subset(array=w1230, length (row)=w1232) -> (w1243:u16[][])  [unwired: 3 in]
                  n848 = call "BRig_dataTrial_nTrial.vi"() -> ("output_nTrial"=w1238:i32)  [unwired: 11 in]
                  n849 = Index Array(array=w1230, index (row)=0, index (col)=w1238) -> (element=w1237:u16)
                  n850 = To Double Precision Float(number=w1243) -> (double precision float=w1242:dbl[][])
                  n851 = Not Equal?(x=u16 1, y=w1237) -> (x != y?=w1235:bool)
                  n852 = call-poly <vilib>:"Write To Spreadsheet File.vi"("delimiter (\\t)"="," ("delimiter (\\t)"), "append to file? (new file:F)"=w1235, "2D data"=w1242, "file path (dialog if empty)"=w1241) -> ("new file path (Not A Path if cancelled)"=w1234:path)  [unwired: 4 in]
                  n853 = call <vilib>:"Is Path and Not Empty.vi"("path"=w1234) -> ("Is Path and Not Empty?"=w1233:bool)  [unwired: 4 in]
                  n854 = Select(t=0, s=w1233, f=w1232) -> (s? t:f=w1229:i32)
                }
              }
              n855 = case shown="True" w1080 {
                tunnel: w1077 -> [w1129 w1149]
                tunnel: w1076 -> [w1128 w1147]
                tunnel: [w1129 w1148] -> w1075
                tunnel: [w1128 w1146] -> w1074
                tunnel: w1073 -> [w1127 w1145]
                tunnel: w1072 -> [w1126 w1143]
                tunnel: [w1127 w1144] -> w1071
                tunnel: [w1126 w1142] -> w1070
                tunnel: w1069 -> [_ w1150]
                tunnel: w1068 -> [_ w1141]
                tunnel: w1067 -> [_ w1140]
                tunnel: w1058 -> [w1124 w1133]
                tunnel: w1057 -> [w1123 w1132]
                tunnel: [w1124 w1131] -> w1056
                tunnel: [w1123 w1130] -> w1055
                frame False {
                  n856 = Wait (ms)(milliseconds to wait=u32 10) -> ()  [unwired: 1 out]
                }
                frame True {
                  n857 = Index Array(array=w1150, index=0) -> (element=w1134:u16)
                  n858 = Equal?(x=w1134, y=u16 1) -> (x = y?=w1135:bool)
                  n859 = Equal?(x=w1134, y=u16 2) -> (x = y?=w1137:bool)
                  n860 = Or(x=w1135, y=w1137) -> (x .or. y?=w1136:bool)
                  n861 = case shown="False" w1136 {
                    tunnel: w1150 -> [w1158 w1206]
                    tunnel: w1149 -> [w1162 w1199]
                    tunnel: [w1162 w1198] -> w1148
                    tunnel: w1147 -> [w1161 w1197]
                    tunnel: [w1161 w1196] -> w1146
                    tunnel: w1145 -> [w1160 w1203]
                    tunnel: [w1160 w1201] -> w1144
                    tunnel: w1143 -> [w1159 w1202]
                    tunnel: [w1159 w1200] -> w1142
                    tunnel: w1141 -> [_ w1205]
                    tunnel: w1140 -> [_ w1204]
                    tunnel: w1135 -> [_ w1195]
                    tunnel: w1134 -> [w1163 _]
                    tunnel: w1133 -> [w1155 w1194]
                    tunnel: w1132 -> [w1156 w1193]
                    tunnel: [w1154 w1194] -> w1131
                    tunnel: [w1153 w1193] -> w1130
                    frame False {
                      n862 = Equal?(x=w1163, y=u16 3) -> (x = y?=w1152:bool)
                      n863 = case shown="True" w1152 {
                        tunnel: w1158 -> [_ w1170]
                        tunnel: w1156 -> [w1164 w1169]
                        tunnel: w1155 -> [w1165 w1168]
                        tunnel: [w1165 w1167] -> w1154
                        tunnel: [w1164 w1166] -> w1153
                        frame False {
                        }
                        frame True {
                          w1177 = 3 ("y")
                          n864 = Array Size(array=w1170) -> (size(s)=w1171:i32)
                          n865 = To Double Precision Float(number=w1171) -> (double precision float=w1172:dbl)
                          n866 = To Double Precision Float(number=w1177) -> (double precision float=w1176:dbl)
                          n867 = Divide(x=w1172, y=w1176) -> (x/y=w1173:dbl)
                          n868 = Round Toward -Infinity(1:w1173) -> (0:w1174:dbl)
                          n869 = To Long Integer(number=w1174) -> (32bit integer=w1175:i32)
                          n870 = for {
                            N: w1175 -> [_]
                            tunnel: w1177 -> [w1192]
                            tunnel: w1170 -> [w1189]
                            shift-right: [w1178] -> w1166
                            shift-left: w1169 -> [w1184]
                            shift-right: [w1179] -> w1167
                            shift-left: w1168 -> [w1186]
                            i -> [w1191]
                            n871 = Multiply(x=2 ("index"), y=w1184) -> (x*y=w1183:i32)
                            n872 = Multiply(x=w1191, y=w1192) -> (x*y=w1190:i32)
                            n873 = Increment(x=w1190) -> (x+1=w1188:i32)
                            n874 = Increment(x=w1188) -> (x+1=w1187:i32)
                            n875 = Increment(x=w1184) -> (x+1=w1178:i32)
                            n876 = Index Array(array=w1189, index #1=w1188, index #2=w1187) -> (element #1=w1181:u16, element #2=w1180:u16)
                            n877 = Increment(x=w1183) -> (x+1=w1182:i32)
                            n878 = Replace Array Subset(array=w1186, new element #1=w1181, index #1=w1183, new element #2=w1180, index #2=w1182) -> (w1179:u16[])
                          }
                        }
                      }
                    }
                    frame True {
                      n879 = case shown="True" w1195 {
                        tunnel: w1206 -> [w1214 w1226]
                        tunnel: w1205 -> [w1212 _]
                        tunnel: w1204 -> [_ w1221]
                        tunnel: w1203 -> [w1216 w1220]
                        tunnel: w1202 -> [w1215 w1222]
                        tunnel: [w1216 w1219] -> w1201
                        tunnel: [w1215 w1218] -> w1200
                        tunnel: w1199 -> [w1211 w1223]
                        tunnel: [w1209 w1223] -> w1198
                        tunnel: w1197 -> [w1208 w1217]
                        tunnel: [w1207 w1217] -> w1196
                        frame True {
                          n880 = Array Subset(array=w1214, index=1, length=w1212) -> (w1210:u16[])
                          n881 = Increment(x=w1208) -> (x+1=w1207:i32)
                          n882 = Replace Array Subset(array=w1211, new element=w1210, index (row)=w1208) -> (w1209:u16[][])  [unwired: 1 in]
                        }
                        frame False {
                          n883 = Array Subset(array=w1226, index=1, length=w1221) -> (w1224:u16[])
                          n884 = Increment(x=w1222) -> (x+1=w1218:i32)
                          n885 = Replace Array Subset(array=w1220, new element=w1224, index (row)=w1222) -> (w1219:u16[][])  [unwired: 1 in]
                        }
                      }
                    }
                  }
                }
              }
            }
            n886 = node-c288(w946) -> ()  [unwired: 1 out]
            n887 = RT FIFO Delete(0:w883, 2:TRUE ("force destroy? (F)"), 3:w877) -> ()  [unwired: 1 out]
            n888 = RT FIFO Delete(0:w843, 2:TRUE ("force destroy? (F)"), 3:w842) -> ()  [unwired: 1 out]
            n889 = flat-sequence {
              tunnel: w917 -> [w1262]
              tunnel: w916 -> [w1265]
              tunnel: w915 -> [w1264]
              tunnel: w914 -> [w1263]
              tunnel: w913 -> [w1267]
              tunnel: w911 -> [_]
              tunnel: w834 -> [w1269]
              tunnel: w881 -> [w1268]
              tunnel: [w1261] -> w892
              tunnel: w877 -> [_]
              tunnel: w910 -> [w1280]
              tunnel: w909 -> [w1279]
              tunnel: w908 -> [w1278]
              tunnel: [w1277] -> w907
              tunnel: [w1276] -> w906
              tunnel: [w1271] -> w902
              tunnel: w892 -> [w1270]
              frame #0 {
                # "Store"
                n890 = call "BRig_RT__Case_Exp__storeData__endExp__v5__p1.vi"("input_dataCurrent"=w1263, "input_dataLC"=w1268, "input_dataExp"=w1269, "input_dataExp_end"=w1264, "input_dataLC_end"=w1265) -> ("output_True"=w1266:bool)  [unwired: 10 in]
                n891 = call "BRig_RT__Case_Exp__storeData__endExp__v5__p2.vi"("input_dataCurrent"=w1263, "input_dataLick"=w1267, "input_True"=w1266, "input_dataMTrig"=w1262) -> ("output_True"=w1261:bool)  [unwired: 11 in]
              }
              frame #1 {
                # "Send"
                n892 = local read "Data Set Prefix"() -> (w1272:string)
                n893 = call "BRig_RT_comm_webdav_upload_all__v3.vi"("input_I_connected_webdav"=w1278, "input_fileName_prefix"=w1272, "input_hSession"=w1279, "input_error"=w1280, "input_True"=w1270) -> ("output_hSession"=w1276:T4, "error out"=w1277:errorcluster, "output_nFilenames"=w1273:i32, "output_arrFilenames"=w1274:string[], "output_uploaded"=w1275:bool[], "output_strCmd"=w1271:string)  [unwired: 5 in]
                n894 = call "BRig_RT_comm_webdav_upload_all_warnUser.vi"("input_n"=w1273, "input_arrFilenames"=w1274, "input_arrUploaded"=w1275) -> ()  [unwired: 9 in]
              }
            }
            n895 = flat-sequence {
              tunnel: w926 -> [w1281]
              tunnel: [w1281] -> w912
              frame #0 {
                w1282 = FALSE ("START")
                n896 = local write "START"(w1282) -> ()
                n897 = local write "STOP_endTrial"(w1282) -> ()
                n898 = local write "STOP_endBlock"(w1282) -> ()
              }
            }
            n899 = xnode "Read/Write Control"("FPGA VI Reference In"=w943, "error in"=w912, "Counts_Reset"=TRUE, "audioTrigger_L"=w929, "audioFreq_L_kHz"=w927, "audioAmp_L"=w928, "audioTrigger_R"=w929, "audioFreq_R_kHz"=w927, "audioAmp_R"=w928, "A3_SL"=w929, "A1_SR"=w929, "A6_Act"=w929) -> ("FPGA VI Reference Out"=w942:refnum<k20>, "error out"=w911:errorcluster)
            n900 = call "BRig_RT__Case_Exp__comm_tcp__data_other.vi"("input_strState"=w902, "input_strAccum"="" ("f"), "input_error"=w903, "input_hTCP"=w904, "input_I_connected_TCP"=w905) -> ("output_error"=w898:errorcluster, "output_hTCP"=w899:refnum<k5>, "output_I_connect_TCP"=w900:bool)  [unwired: 3 in, 1 out]
          }
        }
        n901 = local read "STOP_abort"() -> (w328:bool)
      }
    }
  }
  n902 = flat-sequence {
    tunnel: w96 -> [w2530]
    tunnel: w95 -> [w2532]
    tunnel: w89 -> [w2531]
    tunnel: [w2531] -> w101
    tunnel: [w2530] -> w100
    tunnel: [w2529] -> w99
    tunnel: w74 -> [w2528]
    tunnel: [w2528] -> w98
    tunnel: w75 -> [w2527]
    tunnel: [w2527] -> w97
    tunnel: w82 -> [w2525]
    tunnel: w81 -> [w2524]
    tunnel: w80 -> [w2523]
    tunnel: w76 -> [w2526]
    tunnel: [w2526] -> w94
    tunnel: w93 -> [_]
    tunnel: [w2525] -> w88
    tunnel: [w2524] -> w87
    tunnel: [w2523] -> w86
    tunnel: w101 -> [w2552]
    tunnel: w100 -> [w2551]
    tunnel: w99 -> [w2550]
    tunnel: [w2549] -> _
    tunnel: w98 -> [w2548]
    tunnel: w97 -> [w2547]
    tunnel: w94 -> [w2546]
    tunnel: w88 -> [w2545]
    tunnel: w87 -> [w2544]
    tunnel: w86 -> [w2543]
    frame #0 {
      # "Stop FPGA\nSend QUIT to Host"
      n903 = case shown="True" w2531 {
        tunnel: w2530 -> [_ w2541]
        tunnel: w2532 -> [w2538 w2540]
        tunnel: [w2538 w2539] -> w2529
        frame False {
        }
        frame True {
          n904 = xnode "Read/Write Control"("FPGA VI Reference In"=w2541, "error in"=w2540, "FPGA_Stop"=TRUE) -> ("error out"=w2539:errorcluster)  [unwired: 1 out]
        }
      }
      n905 = case shown="True" w2525 {
        tunnel: w2524 -> [_ w2537]
        tunnel: w2523 -> [_ w2536]
        frame False {
        }
        frame True {
          w2533 = "<S,Q><S,Q><S,Q><S,Q>" ("input_packet")
          n906 = call "BRig_RT_comm_tcp_write_RTwrite.vi"("input_error"=w2536, "input_packet"=w2533, "input_hTCP"=w2537) -> ("output_error"=w2535:errorcluster, "output_hTCP"=w2534:refnum<k5>)  [unwired: 5 in, 2 out]
          n907 = call "BRig_RT_comm_tcp_write_RTwrite.vi"("input_error"=w2535, "input_packet"=w2533, "input_hTCP"=w2534) -> ()  [unwired: 5 in, 4 out]
        }
      }
    }
    frame #1 {
      # "Disconnect FPGA\nDisconnect comm webdav"
      n908 = case shown="True" w2552 {
        tunnel: w2550 -> [w2557 w2560]
        tunnel: w2551 -> [_ w2559]
        tunnel: [w2557 w2558] -> w2549
        frame False {
        }
        frame True {
          n909 = xnode "Close FPGA VI Reference"("FPGA VI Reference In"=w2559, "error in"=w2560) -> ("error out"=w2561:errorcluster)
          n910 = call <vilib>:"Reset myRIO.vi"("error in (no error)"=w2561) -> ("error out"=w2558:errorcluster)  [unwired: 10 in]
        }
      }
      n911 = case shown="True" w2545 {
        tunnel: w2544 -> [_ w2554]
        tunnel: w2543 -> [_ w2553]
        frame False {
        }
        frame True {
          n912 = TCP Close Connection(connection ID=w2554, error in (no error)=w2553) -> ()  [unwired: 1 in, 2 out]
        }
      }
      n913 = case shown="True" w2548 {
        tunnel: w2547 -> [_ w2556]
        tunnel: w2546 -> [_ w2555]
        frame False {
        }
        frame True {
          n914 = call <vilib>:"Close Session.vi"("session handle"=w2556, "error in (no error)"=w2555) -> ()  [unwired: 13 in, 1 out]
        }
      }
    }
  }
  n915 = Flush Stream(8:w1, 11:w2) -> (0:w3:errorcluster, 3:w4:refnum<k21>)  [unwired: 2 in, 1 out]
  n916 = Flush Stream(8:w13, 11:w14) -> (0:w15:errorcluster, 3:w16:refnum<k21>)  [unwired: 2 in, 1 out]
  n917 = Destroy Stream Endpoint(8:w3, 11:w4) -> ()  [unwired: 1 out]
  n918 = Destroy Stream Endpoint(8:w15, 11:w16) -> ()  [unwired: 1 out]
